vi "FS-EPR(FDMR)-main.vi"() -> ()   [LabVIEW 2022 SP3]
doc: "Demonstrates the fundamentals of the State Machine design pattern in LabVIEW. A state machine, in its simplest form, is a case structure within a while loop, with a state enum wired to a shift register on the loop to define the execution of different cases (or \"states\") of the case structure on different iterations of the loop."
uses:
  Subsystem modules/Messenger service/MessengerLib.lvlib
  Datatypes/TopStates.ctl
  Subsystem modules/Magnet module/ctl/Magnet Orders.ctl
  Subsystem modules/Magnet module/Magnet module.lvlib
  Subsystem modules/Magnet module/ctl/MSG to magnet.ctl
  Subsystem modules/Servo drive module/ctl/Axis names.ctl
  Subsystem modules/Servo drive module/Servo drive module.lvlib
  Subsystem modules/Servo drive module/ctl/Servo MSG.ctl
  Subsystem modules/Servo drive module/ctl/Servo commands.ctl
  Subsystem modules/Magnet module/ctl/SetField data.ctl
  Subsystem modules/Magnet module/ctl/RampingOutput.ctl
  Subsystem modules/Magnet module/ctl/Magnet mode.ctl
  Subsystem modules/Magnet module/ctl/Overall status.ctl
  Subsystem modules/Magnet module/ctl/TM Revision.ctl
  Subsystem modules/Servo drive module/ctl/Servo constants.ctl
  Subsystem modules/Servo drive module/ctl/Servo variables.ctl
  Subsystem modules/Servo drive module/ctl/Servo state.ctl
  Subsystem modules/Servo drive module/ctl/Status variable change.ctl
  Datatypes/Connected modules.ctl
  Subsystem modules/THz module/ctl/THz Message for module.ctl
  Subsystem modules/THz module/THz source modeule.lvlib
  Subsystem modules/Lock-in module/ctl/MFLI_command enum.ctl
  Subsystem modules/Lock-in module/Lock-in module.lvlib
  Subsystem modules/Lock-in module/ctl/MFLI_message for module.ctl
  Subsystem modules/Sample rotator/ctl/Rotator commands.ctl
  Subsystem modules/Sample rotator/SampleRotator.lvlib
  Subsystem modules/Magnet module/ctl/Magnet mode public.ctl
  Subsystem modules/Magnet module/ctl/Actual magnet state.ctl
  Subsystem modules/Sample rotator/ctl/Axis status.ctl
  Subsystem modules/Sample rotator/ctl/Positoin to set.ctl
  Subsystem modules/Sample rotator/ctl/Motion Properties.ctl
  Subsystem modules/Lock-in module/ctl/MFLI parameters.ctl
  <instrlib>/Zurich Instruments LabOne/Public/Data/ziTypeDemodSampleSingle.ctl
  <instrlib>/Zurich Instruments LabOne/Zurich Instruments LabOne.lvlib
  <instrlib>/Zurich Instruments LabOne/Public/ziTypeHandle.ctl
  Subsystem modules/THz module/ctl/THz sweep parameters.ctl
  Subsystem modules/Sample rotator/ctl/MSG to Rotator.ctl
  Subsystem modules/Temperature control module/ctl/TC sensors.ctl
  Subsystem modules/Temperature control module/Temperature controller.lvlib
  Subsystem modules/Temperature control module/ctl/MSG for VTI.ctl
  Subsystem modules/Magnet module/ctl/Cryostat temperature sensors.ctl
  Datatypes/experiment state.ctl
  Subsystem modules/Temperature control module/ctl/TC commands.ctl
  Subsystem modules/Lock-in module/ctl/ACQ info.ctl
  Datatypes/SampleHolders.ctl
  <userlib>/_OpenG.lib/variantconfig/variantconfig.llb/openg_variant_configuration_file.lvlib
  <vilib>/Utility/config.llb/NI_LVConfig.lvlib
  Datatypes/Instr Info.ctl
  Subsystem modules/Lock-in module/ctl/MFLI_parameter and value.ctl
  Datatypes/Single servo status.ctl
  Datatypes/Measurement info.ctl
  Subsystem modules/Temperature control module/ctl/Set point.ctl
  Datatypes/THz parameters.ctl
  Subsystem modules/Lock-in module/ctl/MFLI_node.ctl
  <vilib>/Utility/sysdir.llb/System Directory Type.ctl
  Datatypes/FDMR plus result.ctl
  Subsystem modules/Sample rotator/ctl/Rotator all.ctl
  Datatypes/FDMR+ script line.ctl
  Subsystem modules/Lock-in module/ctl/ADQ data.ctl
  Subsystem modules/THz module/ctl/THz commands enum.ctl
  <vilib>/Analysis/NI_AALPro.lvlib
  <vilib>/Analysis/2dsp.llb/Decimate (single shot, DBL).vi
  Subsystem modules/Lock-in module/ctl/OSC sampling rate.ctl
  Subsystem modules/Source meter/ctls/SMU status.ctl
  Subsystem modules/Source meter/Source meter.lvlib
  Subsystem modules/Source meter/ctls/SMU Commands.ctl
  Subsystem modules/Source meter/ctls/MSG to SMU.ctl
  Subsystem modules/THz module/ctl/THz MW generator constants.ctl
  Datatypes/Magnet controls.ctl
  Datatypes/Servo controls.ctl
  Subsystem modules/Temperature control module/ctl/Set temperature.ctl
  Subsystem modules/Source meter/ctls/SMU settings.ctl
  Datatypes/FDMR script generator options.ctl
  Datatypes/Rotator controls.ctl
  Datatypes/Acquisition controls.ctl
panel:
  out "Instr status":T1 caption="Connected instuments"
  out "Acummulated data":sgl[][](array[numeric])
  out "Lock-in data":T2
  out "FDMR plus results":T3[](array[typedef])
  out "tdms FDMR file ref":refnum<k34>
  out "Controls referencies":T4
  out "Tmp [K]":T5={"1st stage"=34.4, "2nd stage"=3.82, "InMag"=4.12, "OutMag"=4.31, "Plate"=7.68, "Switch"=8.53, "VTI"=55.04, "Sample"=59.48}
  out "Busy":bool
  in  "Stop":bool
  out "Magnetic\nfield state":bool
  out "data time":timestamp
  out "New data":bool
  out "Instr control refs":refnum<vi>[](array[refnum])
  out "Tmp reched time":dbl format="%<%H:%M:%S>T"
  out "VTI tmp reached":bool
  out "Running experiment":bool
  out "Temperature log ref":refnum<file>
  out "1 round\ntime":u32
  out "loggersRef":refnum<file>
  in  "Tab Control":T6(tab)
  out "Drift[K/min]":dbl[](array[numeric])
  in  "Log folder":path=path "C:/HFEPR logs"
  in  "Disconnect":bool
  in  "Select module":T7(ring)
  out "Logger":string[](array[string])
  in  "Re-connect instruments":bool
  in  "System config file path":path=path "M:/Instrument/HFEPR spectrometer/Software developement/Multi-EPR plus ultra/SystemData/config.ini"
  out "Instr info":T8 {"PwrMonitor"."Last update" format="%<%H:%M:%S>T"; "VTI"."Last update" format="%<%H:%M:%S>T"; "PMD"."Last update" format="%<%H:%M:%S>T"; "SMU"."Last update" format="%<%H:%M:%S>T"; "Servo"."Last update" format="%<%H:%M:%S>T"; "Rotator"."Axes"."Actuator" items=["Linear", "Roatator", "Goniometer"]; "Rotator"."Name" items=["ANC350res", "ANC350num", "ANC350fps", "Unknown"]; "Rotator"."Last update" format="%<%H:%M:%S>T"; "THz"."Last update" format="%<%H:%M:%S>T"; "MFLI"."Last update" format="%<%H:%M:%S>T"; "Magnet"."Last update" format="%<%H:%M:%S>T"}
  in  "Use previous settings":bool=TRUE
  out "Temperature monitor":T12(graph)
  in  "Real instruments":bool=TRUE
  in  "Password is admin":string
  in  "VTI control":T13={"VTI space [K]"=1.0, "Sample [K]"=0.0, "Heater3 [K]"=1.8, "Heater4 [K]"=1.8, "Out 1 [%]"=0.0, "Out 2 [%]"=0.0, "Range out 1"=1} {"Range out 1" items=["Off", "Range 1 (On)", "Range 2", "Range 3", "Range 4", "Range 5"]; "Heater4 [K]" min=1.8 max=300.0; "Heater3 [K]" min=1.8 max=300.0}
  in  "Acquisition controls":T14={"ACQ parameters"={"Filter order"=7.0, "Filter tau [ms]"=10.0, "F_Mod [kHz]"=1.0, "Amp_Mod [mV]"=10.0, "Enable output"=0, "Phase [°]"=0.0}, "ACQ shot btn"=FALSE, "Modulation [A]"=0.0, "In50"=FALSE, "Out50"=FALSE, "DemEn"=FALSE, "Actual [G]"=0.0, "Sample holder"=enum."Simple", "Desired [G]"=0.0, "Adj mod"=FALSE, "Auto-modulation"=TRUE, "Autorange"=FALSE, "AuxIn0 [V]"=0.0, "AuxIn1 [V]"=0.0} {"AuxIn1 [V]" format="%#_3g"; "AuxIn0 [V]" format="%#_3g"; "Desired [G]" format="%.1g"; "ACQ parameters"."Enable output" items=["Disable", "Enable"]; "ACQ parameters"."Amp_Mod [mV]" min=0.0 max=10000.0; "ACQ parameters"."F_Mod [kHz]" min=0.1 max=500.0; "ACQ parameters"."Filter order" min=1.0 max=9.0 step=1.0; "ACQ parameters"."Filter tau [ms]" min=0.0 max=1000.0}
  in  "VID control":T17={"AMC"=9, "Multip"=1, "Base frequency [GHz]"=0.0, "End frequency [GHz]"=0.0, "Im frequency [MHz]"=1500.0, "Sweep up [ms]"=0.0, "Reset trigger?"=FALSE} {"Multip" items=["1"=1, "2"=2, "3"=3, "4"=4, "6"=6, "8"=8, "9"=9]; "AMC" items=["9"=9, "12"=12]; "End frequency [GHz]" min=0.00018 max=20000.0; "Base frequency [GHz]" min=162.0 max=252.0}
  in  "Servo controls":T18={"Y left"=FALSE, "Y right"=FALSE, "X backward"=FALSE, "X forward"=FALSE, "Zdown"=FALSE, "Zup"=FALSE, "Step\n[mm]"=5.0, "QO table"={"ZLdown"=FALSE, "ZLup"=FALSE, "ZRup"=FALSE, "ZRdown"=FALSE, "ZMdown"=FALSE, "ZMup"=FALSE}, "X"=0.0, "Y"=0.0, "ZL"=0.0, "ZR"=0.0, "ZM"=0.0, "Measure Position btn"=FALSE, "Eject position btn"=FALSE, "Stop servo btn"=FALSE, "Save position btn"=FALSE} {"Step\n[mm]" min=0.0 max=600.0 step=5.0}
  in  "Magnet controls":T19 {"Output\n[T]" scale=0.0..16.0; "Field\n[T]" scale=0.0..16.0; "Desired ramp\nrate [mT/s]" max=7.544966; "Set Field [T]" max=16.0}
  out "lookup":cluster{"X (Vrms)":dbl, "Y (Vrms)":dbl}(graph) caption="Waveform Chart - Dark"
  in  "SMU controls":T21={"Apply"=FALSE, "Measurement settings"={"Source Mode "=1, "Source Level"=0.1, "Source Limit"=0.3, "Measure Function"=0, "Remote sense"=TRUE, "Clear buffer?"=FALSE, "Beep"=TRUE, "High Capacity"=TRUE, "Terminals"=0, "PLCs"=1.0, "Fast measurement"=FALSE}, "Value"=0.1006, "Stop"=FALSE, "Record"=FALSE, "B[T]"=0.0, "Refresh"=FALSE} {"Value" format="%#_3e"; "Measurement settings"."Measure Function" items=["Volts", "Current", "Auto Resistance", "Manual Resistance", "Digitize Voltage", "Digitize Current"]; "Measurement settings"."Source Level" max=0.3; "Measurement settings"."Source Mode" items=["Voltage", "Current"]; "Measurement settings"."Terminals" items=["Front", "Rear"]}
  in  "Rotator controls":T22={"Motion properties"={"Frequency [Hz]"=1000.0, "MaxErr [µm|m°]"=100.0, "DC voltage [V]"=0.0, "Amplitude [V]"=25.0, "Position [mm|°]"=0.0, "EoF"=FALSE, "EoB"=FALSE, "Error"=FALSE, "Target [mm|°]"=0.0}, "Set position"={"Relative?"=FALSE, "Position [°]"=0.0, "Safe to move?"=FALSE}, "Actual \nangle[°]"=0.0, "Rot set properties btn"=FALSE, "Rot set position btn"=FALSE, "Stop btn"=FALSE, "EoF"=FALSE, "EoB"=FALSE, "Error"=FALSE} {"Motion properties"."Amplitude [V]" min=0.0 max=60.0 step=1.0; "Motion properties"."DC voltage [V]" min=0.0 max=60.0 step=1.0; "Motion properties"."MaxErr [µm|m°]" min=1.0 max=1000.0 step=1.0; "Motion properties"."Frequency [Hz]" min=0.1 max=5000.0 step=10.0}
  in  "Save data option":bool
  in  "Load from editor btn":bool
  out "Line":i32
  in  "Script array":T25[](array[typedef])=[{"F_start [GHz]"=180.0, "F_end [GHz]"=196.0, "Field [T]"=6.8, "Points [-]"=8000, "Sampling Rate"=13, "ModA [G]"=4.0, "ModF [kHz]"=40.1, "Time const [ms]"=0.5, "Angle [°]"=-1.0, "Tmp [K]"=55.0, "Wait [min]"=5.0, "Repeat [-]"=127, "Comment"="example comment", "Execute"=TRUE, "Auto-mod"=FALSE}] {"Sampling Rate" items=["117 ks/S"=9, "58.6 kS/s"=10, "29.3 kS/s"=11, "14.6 kS/s"=12, "7.32 kS/s"=13, "3.66 kS/s"=14, "1.83 kS/s"=15]; "Angle [°]" min=-1.0 max=330.0; "ModA [G]" min=0.0 max=50.0; "Repeat [-]" min=0 max=1048576; "Points [-]" min=4096 max=5000000 step=1; "Field [T]" min=-16.0 max=16.0}
  out "Live spectrum":dbl[][](graph) caption="Live Spectrum"
  in  "Folder path":path
  in  "Sample name":string="Unknown"
  in  "Run FDMR+ btn":bool
  in  "Direct stop meas. btn":bool
  out "Infobar":T27={"Remains"=0.0, "T_sample [K]"=59.48, "Last log"="Measurement has finished at 11:20:43", "Experiment state"=enum."Setup", "Field [T]"=6.8, "Sample holder"=enum."Simple", "Started"=timestamp(38104 s since 1904-01-01)} {"Started" format="%<%H:%M:%S>T"; "Remains" format="%<%H:%M:%S>t"}
  out "Accumulated Spectrum":dbl[][](graph)
  out "Round":i32
  in  "Load from measurement btn":bool
  in  "Save script btn":bool
  in  "Clear script btn":bool
  in  "Generate script btn":bool
  in  "Generator options":T29
  in  "Editor script":T25[](array[typedef]) {"Sampling Rate" items=["117 ks/S"=9, "58.6 kS/s"=10, "29.3 kS/s"=11, "14.6 kS/s"=12, "7.32 kS/s"=13, "3.66 kS/s"=14, "1.83 kS/s"=15]; "Angle [°]" min=-1.0 max=330.0; "ModA [G]" min=0.0 max=50.0; "Repeat [-]" max=1048576; "Points [-]" min=4096 max=5000000 step=1; "Field [T]" min=-16.0 max=16.0}
  in  "Prototype line":T25={"F_start [GHz]"=380.0, "F_end [GHz]"=400.0, "Field [T]"=0.0, "Points [-]"=1, "Sampling Rate"=15, "ModA [G]"=100.0, "ModF [kHz]"=10.0, "Time const [ms]"=1.0, "Angle [°]"=-1.0, "Tmp [K]"=295.0, "Wait [min]"=0.0, "Repeat [-]"=1, "Comment"="", "Execute"=FALSE, "Auto-mod"=FALSE} {"Sampling Rate" items=["117 ks/S"=9, "58.6 kS/s"=10, "29.3 kS/s"=11, "14.6 kS/s"=12, "7.32 kS/s"=13, "3.66 kS/s"=14, "1.83 kS/s"=15]; "Angle [°]" min=-1.0 max=330.0; "ModA [G]" min=0.0 max=50.0; "Repeat [-]" max=1048576; "Points [-]" min=4096 max=5000000 step=1; "Field [T]" min=-16.0 max=16.0}
  out "Opend review file path":path
  out "Current review graph parameters":T25={"F_start [GHz]"=380.0, "F_end [GHz]"=400.0, "Field [T]"=0.0, "Points [-]"=1, "Sampling Rate"=15, "ModA [G]"=1.0, "ModF [kHz]"=10.0, "Time const [ms]"=1.0, "Angle [°]"=-1.0, "Tmp [K]"=295.0, "Wait [min]"=0.0, "Repeat [-]"=0, "Comment"="", "Execute"=FALSE, "Auto-mod"=FALSE} {"Sampling Rate" items=["117 ks/S"=9, "58.6 kS/s"=10, "29.3 kS/s"=11, "14.6 kS/s"=12, "7.32 kS/s"=13, "3.66 kS/s"=14, "1.83 kS/s"=15]; "Time const [ms]" min=-1.0 max=330.0; "ModF [kHz]" min=0.2 max=120.0; "Repeat [-]" max=1048576; "Points [-]" max=50; "Wait [min]" max=1048576.0; "Field [T]" min=-16.0 max=16.0}
  out "Previous graph":sgl[][](graph)
  out "Current graph":sgl[][](graph)
  in  "Open measurement":bool
  in  "Data to show":u16(ring) items=["Empty", "Empty", "Empty", "Empty", "Empty", "Empty", "Empty", "Empty", "Empty", "Empty"]
  # "Action part"
  # "Status part"
  # "Option 1:\nchoice primary and secondary sweep\n\nOption 2:\nChoice measurement mode, and appropriate cluster will apear. Other clusters wil be hidden.\n\n\nOption 3:\nChoice measurement mode.\nInternal parts of single cluster will (dis)apear if needed.\n\nNote:\nPosibility to do an orientation/temperature deppendency."
  # "Tmp [K]"
  # "Position [mm]"
  # "Z"
  # "X/Y"
  # "This software was developed for HFEPR spectrometer in 2019 (2020) at CEITEC BUT by members of MOTES research group.\n\nQuick guide:\n1) Re-connect to all instruments.\n2) Check if necessary instruments are ready. (At least VTI, VDI, Lock-In, and Magnet has to work)\n3) Go to Adjustment tab and set up Lock-in parameters as well as VDI multipiers.\n4) Go to EPR measurement tab, select folder path, fill the sample description.\n5) Fill at least 1 line of the script and press Run script button.\n\n6) In case of a bug please report this to software developer or make a note into developement diary loaceted at:\n    RG-1-12/Instriments/HFEPR spectrometer/Software developement.\n\nLast update: 07.02. 2020 - Script editor is working, measurement review not yet.\n\nSpecial thanks to: Luke Skywalker, my mom, Tonda's mom, Pilsner, God, Oleksi, Vinicius, Petr from parallel universe.\n\n \nTODO: Invisible controls: referencies for: adjustment controls, meas results, loggerRef,"
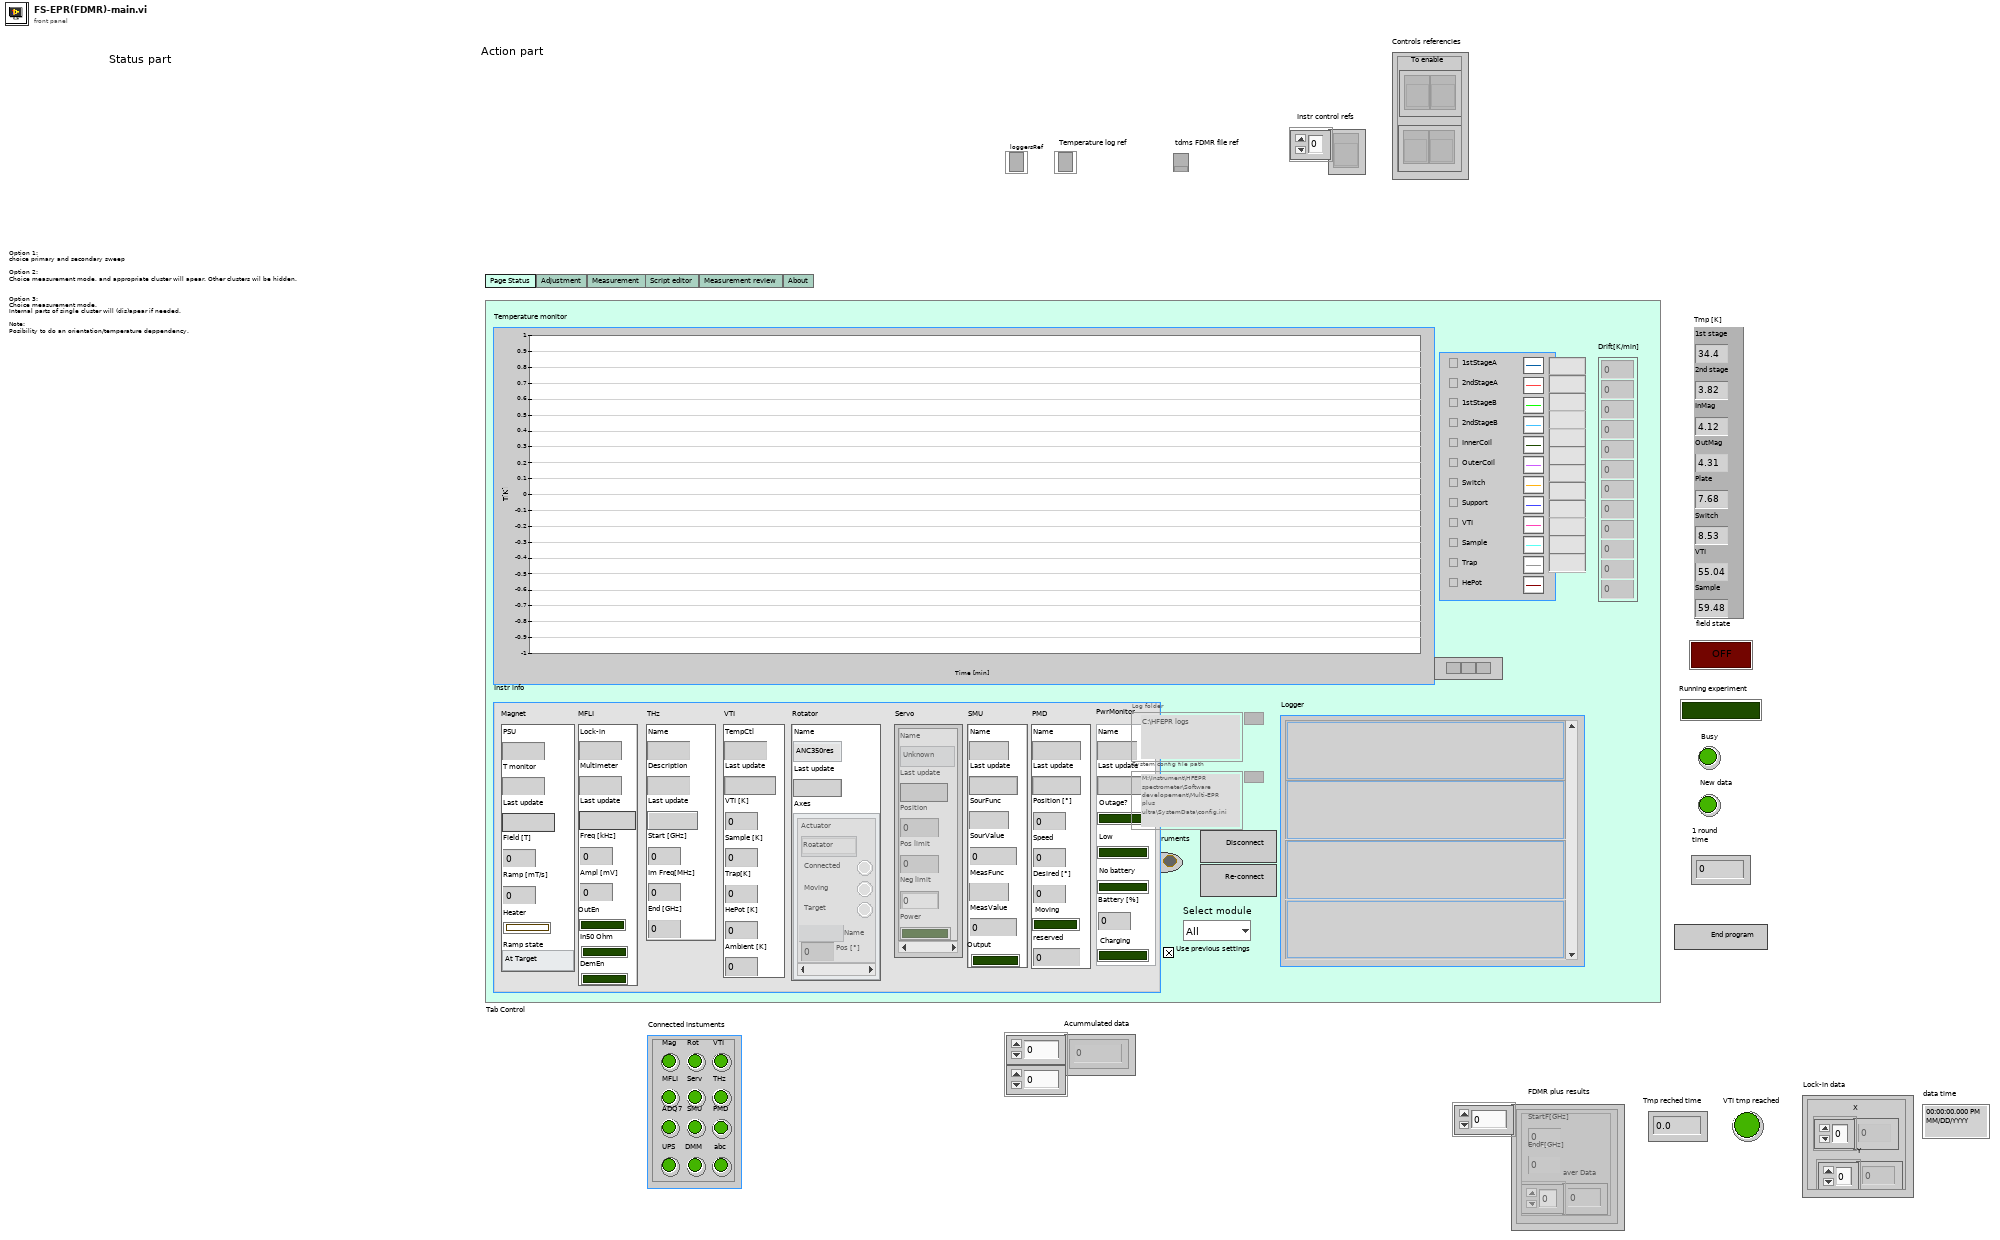
[diagram p1: front panel]
types:
  T1 = typedef "Connected modules.ctl" = cluster{"Mag":bool, "Rot":bool, "VTI":bool, "MFLI":bool, "Serv":bool, "THz":bool, "ADQ7":bool, "SMU":bool, "PMD":bool, "UPS":bool, "DMM":bool, "abc":bool}
  T2 = typedef "Lock-in module.lvlib/ADQ data.ctl" = cluster{"X":sgl[], "Y":sgl[]}
  T3 = typedef "FDMR plus result.ctl" = cluster{"StartF[GHz]":dbl, "EndF[GHz]":dbl, "aver Data":dbl[]}
  T4 = cluster{"To disable":refnum<vi>[], "To enable":refnum<vi>[]}
  T5 = cluster{"1st stage":dbl, "2nd stage":dbl, "InMag":dbl, "OutMag":dbl, "Plate":dbl, "Switch":dbl, "VTI":dbl, "Sample":dbl}
  T6 = enum32{"Page Status", "Adjustment", "Measurement", "Script editor", "Measurement review", "About"}
  T7 = enum16{"All", "None", "ACQ", "THz", "MAG", "SERV", "ROT", "VTI", "SMU"}
  T8 = typedef "Instr Info.ctl" = cluster{"Magnet":cluster{"PSU":string, "T monitor":string, "Last update":timestamp, "Field [T]":dbl, "Ramp [mT/s]":dbl, "Heater":bool, "Ramp state":T9}, "MFLI":cluster{"Lock-in":string, "Multimeter":string, "Last update":timestamp, "Freq [kHz]":dbl, "Ampl [mV]":dbl, "OutEn":bool, "In50 Ohm":bool, "DemEn":bool}, "THz":cluster{"Name":string, "Description":string, "Last update":timestamp, "Start [GHz]":dbl, "Im Freq[MHz]":dbl, "End [GHz]":dbl}, "VTI":cluster{"TempCtl":string, "Last update":timestamp, "VTI [K]":dbl, "Sample [K]":dbl, "Trap[K]":dbl, "HePot [K]":dbl, "Ambient [K]":dbl}, "Rotator":cluster{"Name":i32, "Last update":timestamp, "Axes":cluster{"Pos [°]":dbl, "Moving":bool, "Name":string, "Actuator":u16, "Target":bool, "Connected":bool}[]}, "Servo":T10[], "SMU":cluster{"Name":string, "Last update":timestamp, "SourFunc":string, "SourValue":dbl, "MeasFunc":string, "MeasValue":dbl, "Output":bool}, "PMD":cluster{"Name":string, "Last update":timestamp, "Position [°]":dbl, "Speed":dbl, "Desired [°]":dbl, "Moving":bool, "reserved":dbl}, "PwrMonitor":cluster{"Name":string, "Last update":timestamp, "Outage?":bool, "Low":bool, "No battery":bool, "Battery [%]":u8, "Charging":bool}}
  T9 = typedef "Magnet module.lvlib/RampingOutput.ctl" = enum16{"At Target", "Go up", "Go down"}
  T10 = typedef "Single servo status.ctl" = cluster{"Name":T11, "Last update":timestamp, "Position":dbl, "Pos limit":dbl, "Neg limit":dbl, "Power":bool}
  T11 = typedef "Servo drive module.lvlib/Axis names.ctl" = enum16{"Unknown", "AxisX", "AxisY", "AxisZ_left", "AxisZ_middle", "AxisZ_right"}
  T12 = cluster{"[0]":dbl, "[1]":dbl, "[2]":dbl, "[3]":dbl, "[4]":dbl, "[5]":dbl, "[6]":dbl, "[7]":dbl, "[8]":dbl, "[9]":dbl, "[10]":dbl, "[11]":dbl}
  T13 = typedef "Temperature controller.lvlib/Set temperature.ctl" = cluster{"VTI space [K]":dbl, "Sample [K]":dbl, "Heater3 [K]":dbl, "Heater4 [K]":dbl, "Out 1 [%]":dbl, "Out 2 [%]":dbl, "Range out 1":u16}
  T14 = typedef "Acquisition controls.ctl" = cluster{"ACQ parameters":T15, "ACQ shot btn":bool, "Modulation [A]":dbl, "In50":bool, "Out50":bool, "DemEn":bool, "Actual [G]":dbl, "Sample holder":T16, "Desired [G]":dbl, "Adj mod":bool, "Auto-modulation":bool, "Autorange":bool, "AuxIn0 [V]":dbl, "AuxIn1 [V]":dbl}
  T15 = typedef "Lock-in module.lvlib/MFLI parameters.ctl" = cluster{"Filter order":dbl, "Filter tau [ms]":dbl, "F_Mod [kHz]":dbl, "Amp_Mod [mV]":dbl, "Enable output":u16, "Phase [°]":dbl}
  T16 = typedef "SampleHolders.ctl" = enum16{"Simple", "Carousel", "Chip", "Rotator", "Liquid"}
  T17 = typedef "THz parameters.ctl" = cluster{"AMC":u16, "Multip":u16, "Base frequency [GHz]":dbl, "End frequency [GHz]":dbl, "Im frequency [MHz]":dbl, "Sweep up [ms]":dbl, "Reset trigger?":bool}
  T18 = typedef "Servo controls.ctl" = cluster{"Y left":bool, "Y right":bool, "X backward":bool, "X forward":bool, "Zdown":bool, "Zup":bool, "Step\n[mm]":dbl, "QO table":cluster{"ZLdown":bool, "ZLup":bool, "ZRup":bool, "ZRdown":bool, "ZMdown":bool, "ZMup":bool}, "X":dbl, "Y":dbl, "ZL":dbl, "ZR":dbl, "ZM":dbl, "Measure Position btn":bool, "Eject position btn":bool, "Stop servo btn":bool, "Save position btn":bool}
  T19 = typedef "Magnet controls.ctl" = cluster{"Set Field [T]":dbl, "Desired ramp\nrate [mT/s]":dbl, "Custom\nramp":bool, "Mode switch":bool, "Pause ramp":bool, "Field\n[T]":dbl, "Output\n[T]":dbl, "Equalize":bool, "Discharge":bool, "Switch \ntmp [K]":dbl, "Direction":bool}
  T20 = typedef "SMU settings.ctl" = cluster{"Source Mode ":u16, "Source Level":dbl, "Source Limit":dbl, "Measure Function":u16, "Remote sense":bool, "Clear buffer?":bool, "Beep":bool, "High Capacity":bool, "Terminals":u16, "PLCs":dbl, "Fast measurement":bool}
  T21 = cluster{"Apply":bool, "Measurement settings":T20, "Value":dbl, "Stop":bool, "Record":bool, "B[T]":dbl, "Refresh":bool}
  T22 = typedef "Rotator controls.ctl" = cluster{"Motion properties":T23, "Set position":T24, "Actual \nangle[°]":dbl, "Rot set properties btn":bool, "Rot set position btn":bool, "Stop btn":bool, "EoF":bool, "EoB":bool, "Error":bool}
  T23 = typedef "Motion Properties.ctl" = cluster{"Frequency [Hz]":dbl, "MaxErr [µm|m°]":dbl, "DC voltage [V]":dbl, "Amplitude [V]":dbl, "Position [mm|°]":dbl, "EoF":bool, "EoB":bool, "Error":bool, "Target [mm|°]":dbl}
  T24 = typedef "Positoin to set.ctl" = cluster{"Relative?":bool, "Position [°]":dbl, "Safe to move?":bool}
  T25 = typedef "FDMR+ script line.ctl" = cluster{"F_start [GHz]":dbl, "F_end [GHz]":dbl, "Field [T]":dbl, "Points [-]":u32, "Sampling Rate":T26, "ModA [G]":dbl, "ModF [kHz]":dbl, "Time const [ms]":dbl, "Angle [°]":dbl, "Tmp [K]":dbl, "Wait [min]":dbl, "Repeat [-]":i32, "Comment":string, "Execute":bool, "Auto-mod":bool}
  T26 = typedef "OSC sampling rate.ctl" = u16
  T27 = typedef "Measurement info.ctl" = cluster{"Remains":dbl, "T_sample [K]":dbl, "Last log":string, "Experiment state":T28, "Field [T]":dbl, "Sample holder":T16, "Started":timestamp}
  T28 = typedef "experiment state.ctl" = enum16{"Setup", "Preparation", "Stabilization", "Begin", "Acquisition", "Save"}
  T29 = typedef "FDMR script generator options.ctl" = cluster{"Field step [T]":dbl, "Angle step[°]":dbl, "Tmp step [K]":dbl, "Iterations[-]":u16, "Script generator option":bool}
  T30 = typedef "TopStates.ctl" = enum16{"Initialize GUI", "Wait for Event", "Check message", "Check measurement", "Stop", "Restart"}
  T31 = typedef "MessengerLib.lvlib/Messenger referencies.ctl" = cluster{"TOP":refnum<queue>, "Instr_M":refnum<queue>, "Field_C":refnum<queue>, "Tmp_M":refnum<queue>, "Tmp_C":refnum<queue>, "Table_C":refnum<queue>, "MW_C":refnum<queue>, "Data_Aq":refnum<queue>, "Mod_M":refnum<queue>, "Field_M":refnum<queue>, "Pwr_M":refnum<queue>, "Angle_C":refnum<queue>, "Sample_C":refnum<queue>, "Reserved":refnum<queue>}
  T32 = enum16{"All", "None", "ACQ", "THz", "MAG", "SERV", "ROT", "VTI"}
  T33 = enum8{"Enabled", "Disabled", "Disabled and Grayed Out"}
  T34 = typedef "Magnet module.lvlib/Magnet mode public.ctl" = enum16{"Persistant", "Ramping"}
  T35 = typedef "Magnet module.lvlib/SetField data.ctl" = cluster{"Field [T]":dbl, "Ramp [T/s]":dbl, "Custom Ramp?":bool, "Mode":T34}
  T36 = typedef "Magnet module.lvlib/Magnet Orders.ctl" = enum16{"Ignore", "Connect", "Update", "Switch mode", "Set field", "Stop ramping", "Equalize output", "Zero output", "Flip polarity", "Blackout", "Set timer", "Eval temperatures", "Disconnect"}
  T37 = typedef "Magnet module.lvlib/MSG to magnet.ctl" = cluster{"Command":T36, "Data":variant}
  T38 = typedef "Servo drive module.lvlib/Servo commands.ctl" = enum16{"Initialize", "Update", "Move by", "Move to", "Stop", "Ignore", "Disconnect", "End"}
  T39 = typedef "Servo drive module.lvlib/Servo MSG.ctl" = cluster{"Command":T38, "Data":variant}
  T40 = typedef "Source meter.lvlib/MSG to SMU.ctl" = cluster{"Command":T41, "Data":variant}
  T41 = typedef "Source meter.lvlib/SMU Commands.ctl" = enum16{"Ignore", "Connect", "Update", "Set measurement", "Start measurement", "Get actual results", "Stop measurement", "Disconnect", "End"}
  T42 = typedef "SampleRotator.lvlib/MSG to Rotator.ctl" = cluster{"Command":T43, "Data":variant}
  T43 = typedef "SampleRotator.lvlib/Rotator commands.ctl" = enum16{"Ignore", "Initialize", "Initialize axes", "Update", "Set parameters", "Stop movement", "Set position", "Disconnect", "End"}
  T44 = typedef "THz source modeule.lvlib/THz commands enum.ctl" = enum16{"Ignore", "Connect", "Update", "Set parameters", "Disconnect", "End"}
  T45 = typedef "THz source modeule.lvlib/THz sweep parameters.ctl" = cluster{"Start [GHz]":dbl, "End [GHz] ":dbl, "Sweep up\ntime [ms]":dbl, "Sweep down\ntime [ms]":dbl, "Intermidiate [MHz]":dbl, "Reset trigger":bool}
  T46 = typedef "THz source modeule.lvlib/THz Message for module.ctl" = cluster{"Command":T44, "Data":variant}
  T47 = typedef "Lock-in module.lvlib/MFLI_parameter and value.ctl" = cluster{"parameter":T48, "value":dbl}
  T48 = typedef "Lock-in module.lvlib/MFLI_node.ctl" = enum16{"None", "filter_order [-]", "filter_constant [ms]", "in_diff", "in_autorange", "in_imp50", "in_AC", "osc_freq [kHz]", "out_ampl [V]", "out_autorange", "out_imp50", "enable output", "enamble ampl", "scope_enable", "scope_rate", "scope_len", "scope_trigEn", "AuxOut_amplify", "Phase_deg", "AuxOut_select"}
  T49 = typedef "Lock-in module.lvlib/MFLI_command enum.ctl" = enum16{"Initialize", "Update", "Set parameters", "Set module", "Set individual parameters", "Get point", "Get array", "Disconnect", "End", "Ignore"}
  T50 = typedef "Lock-in module.lvlib/MFLI_message for module.ctl" = cluster{"Command":T49, "Data":variant}
  T51 = typedef "Temperature controller.lvlib/Set point.ctl" = cluster{"Heater":string, "Tmp [K]":dbl}
  T52 = typedef "Temperature controller.lvlib/TC commands.ctl" = enum16{"Initialize", "Update", "Stop tmp change", "Set temperature", "Set point", "Disconnect", "End", "Ignore"}
  T53 = typedef "Temperature controller.lvlib/MSG for VTI.ctl" = cluster{"Command":T52, "Data":variant}
  T54 = typedef "THz source modeule.lvlib/THz MW generator constants.ctl" = cluster{"Lower limit [GHz]":dbl, "Upper limit [GHz]":dbl, "Device name":string, "Connection":string, "Description":string, "Connected":bool, "Last settings":string, "Operation mode":enum16{"Disabled", "CW", "Arbitrary", "Sweep"}, "Enable ch 1":bool, "Enable ch 2":bool}
  T55 = typedef "Magnet module.lvlib/TM Revision.ctl" = cluster{"Instr Serial Number":string, "Instr Driver Revision":string, "Instr Firmware Revision":string, "Instr Model Number":string}
  T56 = typedef "Magnet module.lvlib/Overall status.ctl" = cluster{"Desired":T35, "Actual":T57}
  T57 = typedef "Magnet module.lvlib/Actual magnet state.ctl" = cluster{"Mode":T58, "Ramping output":T9, "Ready for change":bool, "Switch heater":bool, "Cooler Overheat":bool, "Coil overheat":bool, "Energized":bool, "Output [T]":dbl, "Field [T]":dbl, "Ramp[T/s]":dbl, "Switch\ntemperature [K]":dbl, "Voltage [V]":dbl, "Current direction":bool}
  T58 = typedef "Magnet module.lvlib/Magnet mode.ctl" = enum16{"Persistant", "Switching", "Ramping", "Quenched"}
  T59 = typedef "Magnet module.lvlib/Cryostat temperature sensors.ctl" = cluster{"First stage A [K]":dbl, "Second stage A [K]":dbl, "Firs stage B [K]":dbl, "Second stage B [K]":dbl, "Inner magnet [K]":dbl, "Outer Magnet [K]":dbl, "Switch [K]":dbl, "Support plate [K]":dbl, "Time stamp":dbl}
  T60 = typedef "Lock-in module.lvlib/ACQ info.ctl" = cluster{"In50":bool, "InAC":bool, "InDiff":bool, "Out50":bool, "OutEN":bool, "OutF[Hz]":dbl, "OutA[V]":dbl, "DemEN":bool, "Const[ms]":dbl, "Order[-]":i32, "Phase [°]":dbl}
  T61 = enum32{"Page Status", "Adjustment", "EPR measurement", "About"}
  T62 = typedef "Zurich Instruments LabOne.lvlib/ziTypeDemodSampleSingle.ctl" = cluster{"Timestamps (ticks)":u64, "X (Vrms)":dbl, "Y (Vrms)":dbl, "Osc Phase (deg)":dbl, "Freq (Hz)":dbl, "DIO":u32, "AuxIn0 (V)":dbl, "AuxIn1 (V)":dbl, "Trigger":u32}
  T63 = typedef "Zurich Instruments LabOne.lvlib/ziTypeHandle.ctl" = cluster{"handleValid":bool, "Conn":u64, "Path Prefix":string, "Handle":u64, "Connected":bool, "Clockbase(s)":dbl}
  T64 = typedef "Source meter.lvlib/SMU status.ctl" = cluster{"VISA name":refnum<visa-resource-name>, "Connected":bool, "Name":string, "Message":string, "Error message":string, "Min voltage":dbl, "Max voltage":dbl, "Min Current":dbl, "Max Current":dbl, "Measurement value":dbl, "Source Voltage":dbl, "Measurement":bool, "Source Current":dbl, "Source Mode":u16, "Measure Function":u16}
  T65 = typedef "Temperature controller.lvlib/TC sensors.ctl" = cluster{"VTI space":dbl, "Sample":dbl, "He pot":dbl, "Trap":dbl, "Ambient":dbl, "SetP_VTI":dbl, "SetP_Smp":dbl, "SetP_Pot":dbl, "SetP_Trap":dbl, "Range out 1":u16, "Out 1 [%]":dbl, "Out 2 [%]":dbl}
  T66 = typedef "Servo drive module.lvlib/Servo state.ctl" = cluster{"Servo variables":T67, "Servo constants":T68, "Connection":variant}
  T67 = typedef "Servo drive module.lvlib/Servo variables.ctl" = cluster{"Terget reached":bool, "Connected":bool, "Power ON":bool, "Operation mode":bool, "Actual position":dbl, "Target position":dbl}
  T68 = typedef "Servo drive module.lvlib/Servo constants.ctl" = cluster{"Name":T11, "Pos position limit [mm]":dbl, "Neg position limit [mm]":dbl, "Pos velocity limit":dbl, "Neg velocity limit":dbl, "Acceleration limit":dbl}
  T69 = typedef "Servo drive module.lvlib/Status variable change.ctl" = cluster{"Property":string, "Value":variant, "Name":T11}
  T70 = typedef "SampleRotator.lvlib/Rotator all.ctl" = cluster{"Controller info":cluster{"deviceNumber":i32, "DeviceType":i32, "ID":u32, "Serial":string, "Address":string, "connected":bool}, "Handle":u64, "FW-Version":i32, "Features":u32, "Axes":T71[], "Path to DLL":path}
  T71 = typedef "SampleRotator.lvlib/Axis status.ctl" = cluster{"Axis status":cluster{"Connected":bool, "Enabled":bool, "Moving":bool, "Target":bool, "EndForward":bool, "EndBackarwd":bool, "Error":bool}, "Position [°]":dbl, "Frequency [Hz]":dbl, "Voltage [V]":dbl, "Capacitance[uF]":dbl, "Name":string, "ActuatorType":u16, "DC offset [V]":dbl, "Tolerance [m°]":dbl, "Index":u8}
  T72 = enum16{"None", "Unity norm", "Mean norm", "Standardization"}
  T73 = enum16{"open", "open or create", "create or replace", "create", "open (read-only)"}
  T74 = typedef "NI_LVConfig.lvlib/Config Data RefNum.ctl" = refnum<k1>
  T75 = typedef "System Directory Type.ctl" = i32
  T76 = typedef "Mudules status.ctl" = cluster{"Mag":bool, "Rot":bool, "VTI":bool, "MFLI":bool, "Serv":bool, "THz":bool, "ADQ7":bool, "SMU":bool, "PMD":bool, "UPS":bool, "DMM":bool, "abc":bool}
  T77 = typedef "Magnet module.lvlib/Magnet config constants.ctl" = cluster{"Switch resistant [K]":dbl, "Switch superconducting [K]":dbl, "First stage critical temperature [K]":dbl, "Second stage critical temperature [K]":dbl, "Inner magnet critical temperature [K]":dbl, "Outer magnet critical temperature [K]":dbl, "Field Constant [T/A]":dbl, "Maximum Current [A]":dbl, "Maximum field [T]":dbl, "Maximum source ramp [A/s]":dbl, "Source precision [T]":dbl, "Ramp limits [A/s]":dbl[], "Field limits [T]":dbl[], "SMS":refnum<visa-resource-name>, "LSC218":refnum<visa-resource-name>}
  T78 = typedef "MessengerLib.lvlib/MSG to TOP.ctl" = cluster{"Module":T79, "Response":string, "Data":variant, "Time":timestamp}
  T79 = typedef "Module name.ctl" = enum16{"Emty", "Magnet", "VTI", "Excitation", "Servo", "Acquisition", "Rotator", "Digitizer", "SMU2450", "Carousel", "Multimeter", "Tmp monitor", "Power monitor"}
  T80 = cluster{"PSU":string, "T monitor":string, "Last update":timestamp, "Field [T]":dbl, "Ramp [mT/s]":dbl, "Heater":bool, "Ramp state":T9}
  T81 = cluster{"TC":string, "Last update":timestamp, "VTI [K]":dbl, "Sample [K]":dbl, "Trap[K]":dbl, "HePot [K]":dbl, "Ambient [K]":dbl}
  T82 = cluster{"Name":string, "Description":string, "Last update":timestamp, "Start [GHz]":dbl, "Im Freq[MHz]":dbl, "End [GHz]":dbl}
  T83 = cluster{"Lock-in":string, "Multimeter":string, "Last update":timestamp, "Freq [kHz]":dbl, "Ampl [mV]":dbl, "OutEn":bool, "In50 Ohm":bool, "DemEn":bool}
  T84 = cluster{"Name":string, "Last update":timestamp, "SourFunc":string, "SourValue":dbl, "MeasFunc":string, "MeasValue":dbl, "Output":bool}
  T85 = cluster{"TempCtl":string, "Last update":timestamp, "VTI [K]":dbl, "Sample [K]":dbl, "Trap[K]":dbl, "HePot [K]":dbl, "Ambient [K]":dbl}
  T86 = cluster{"Name":i32, "Last update":timestamp, "Axes":cluster{"Pos [°]":dbl, "Moving":bool, "Name":string, "Actuator":u16, "Target":bool, "Connected":bool}[]}
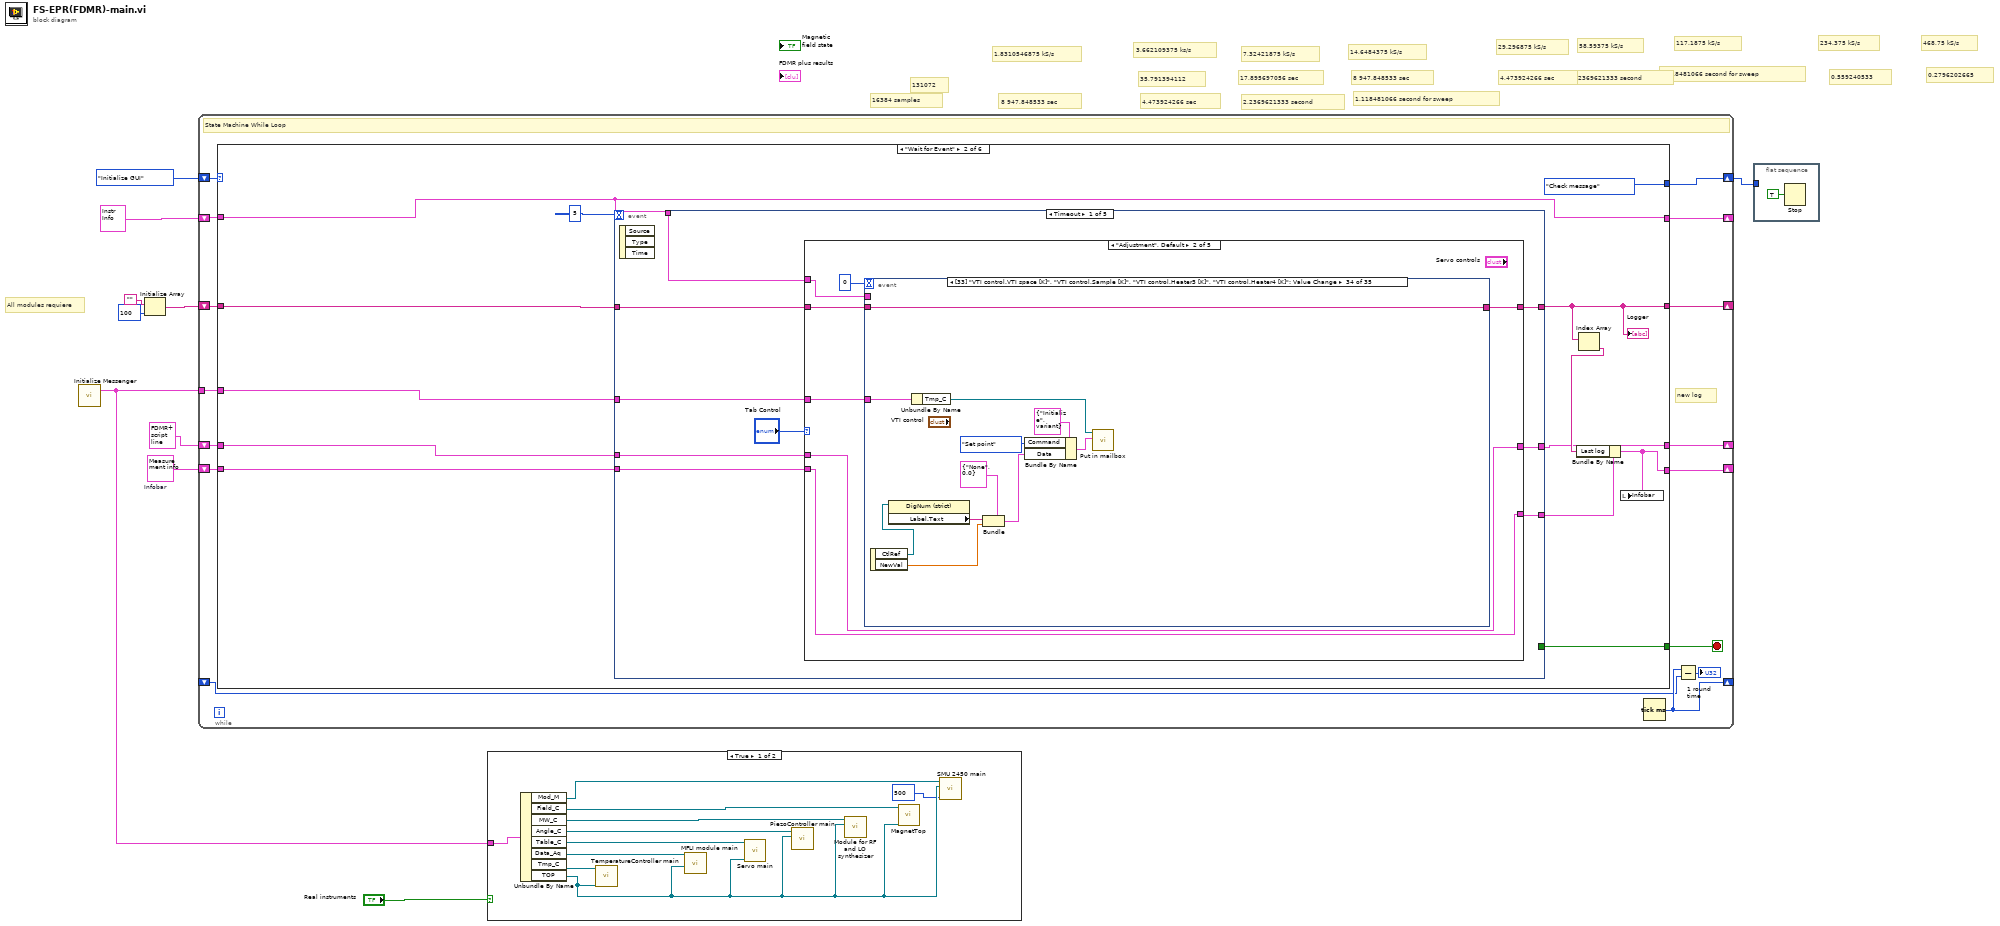
[diagram p0: block diagram]
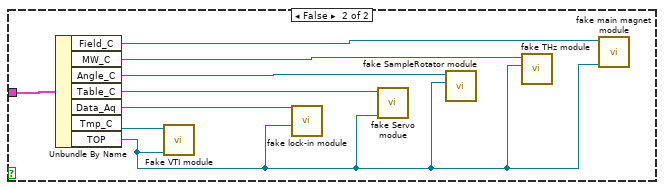
[diagram p2: hidden frame]
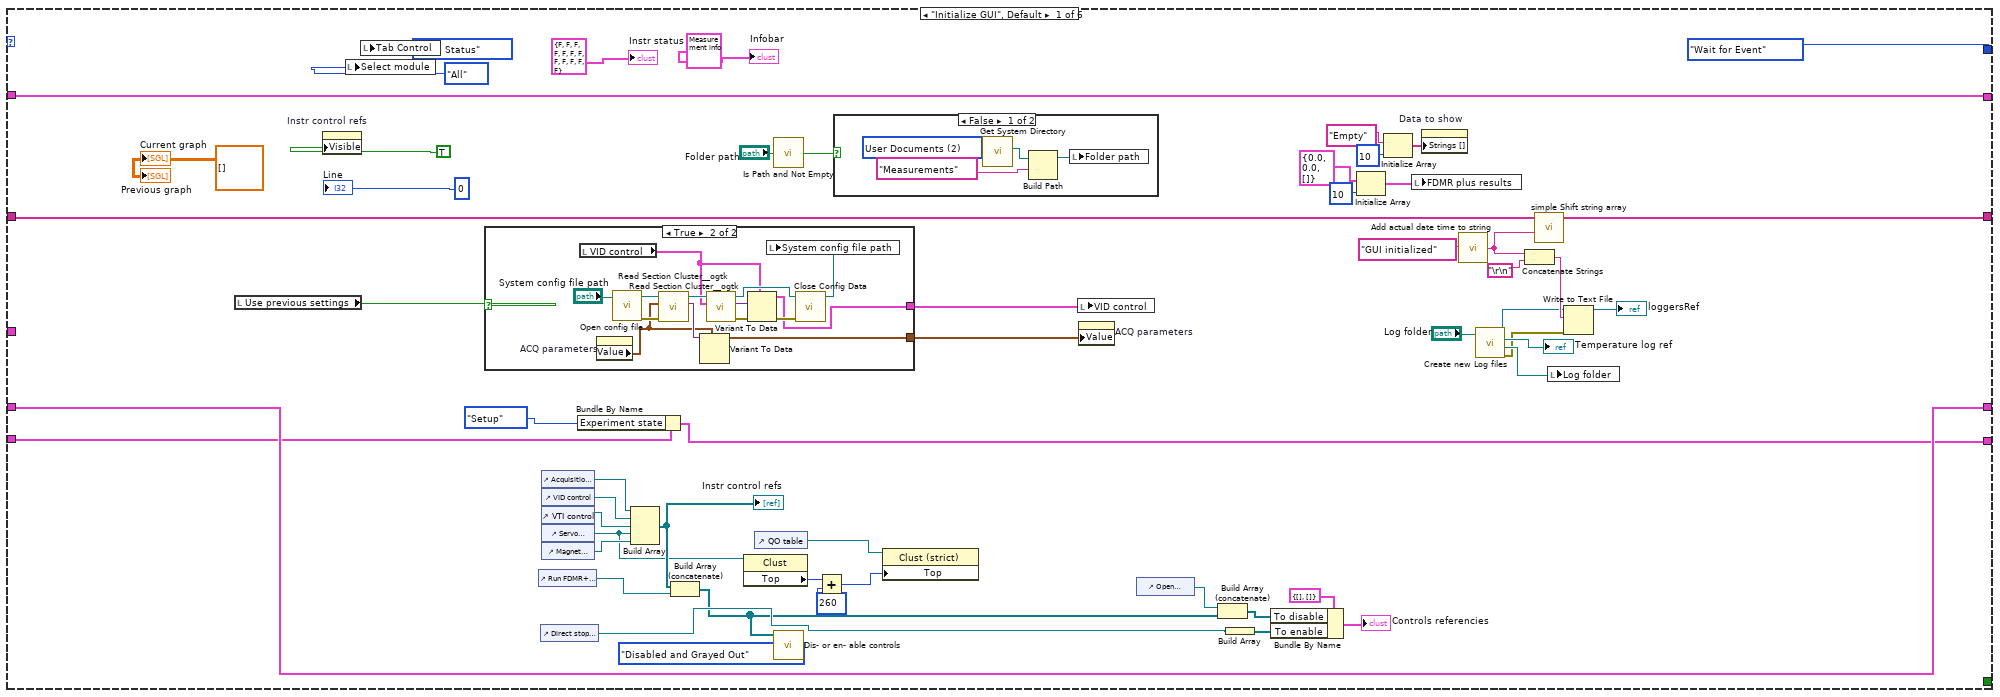
[diagram p3: hidden frame]
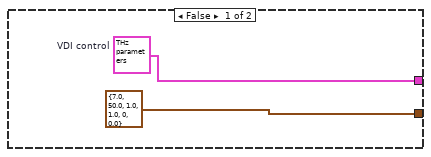
[diagram p5: hidden frame]
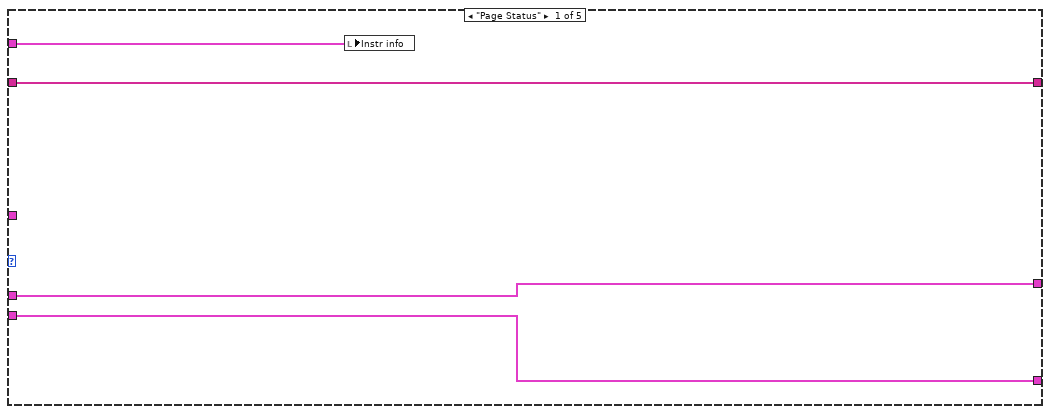
[diagram p6: hidden frame]
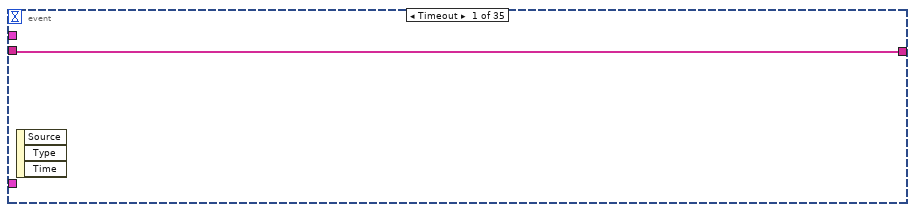
[diagram p7: hidden frame]
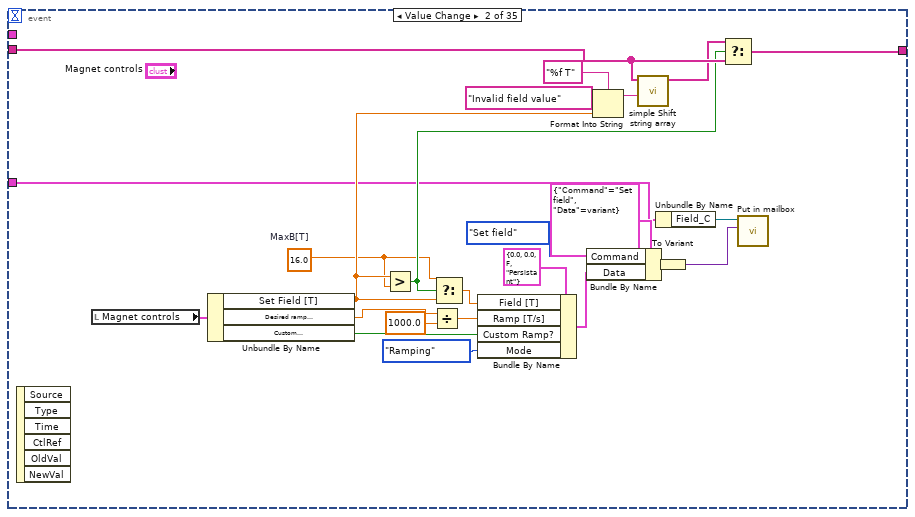
[diagram p8: hidden frame]
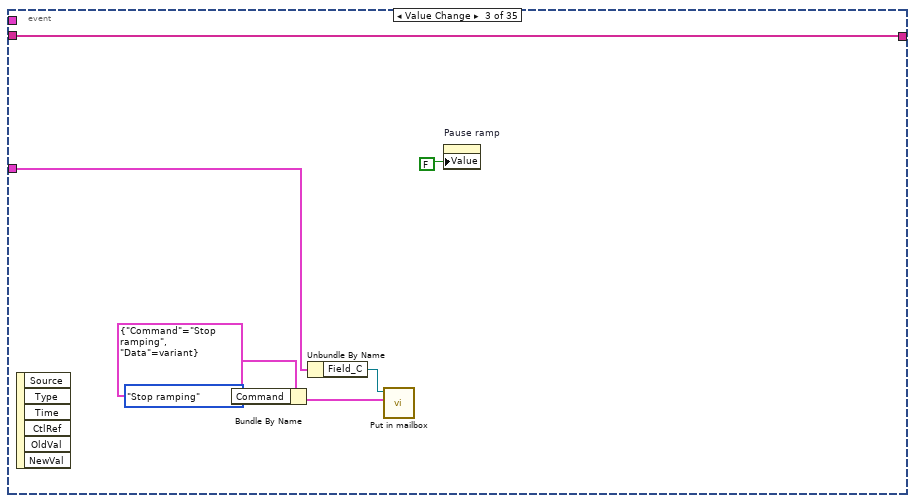
[diagram p9: hidden frame]
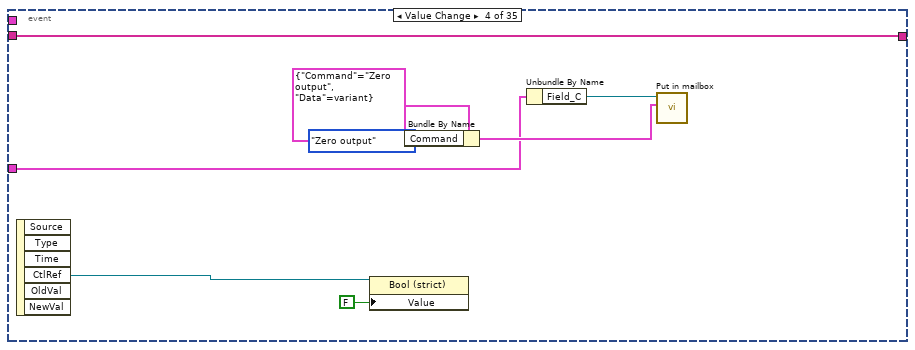
[diagram p10: hidden frame]
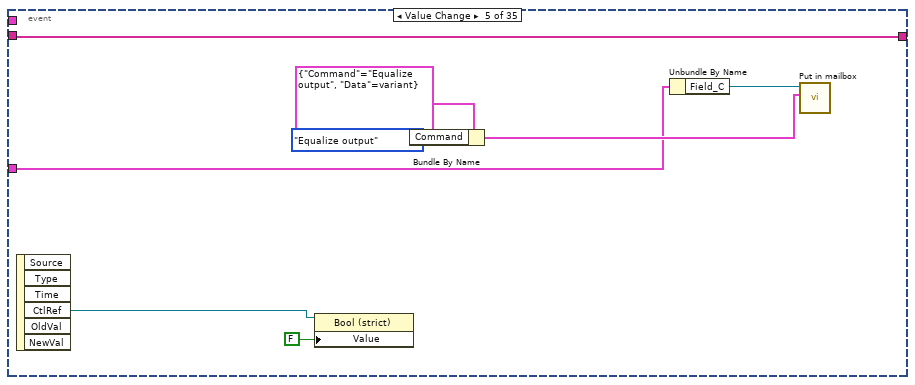
[diagram p11: hidden frame]
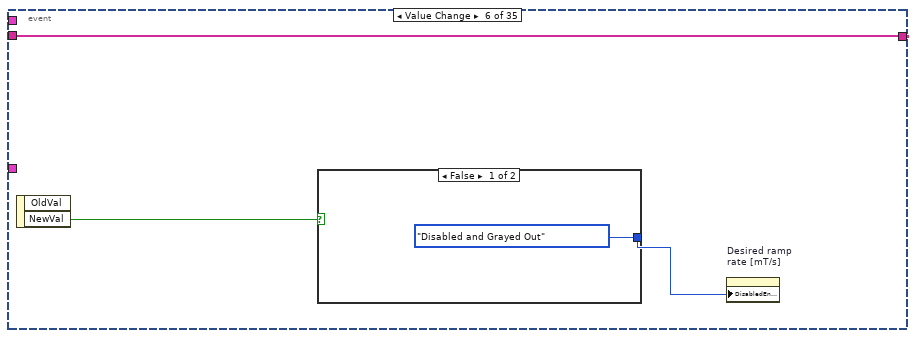
[diagram p12: hidden frame]
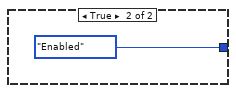
[diagram p13: hidden frame]
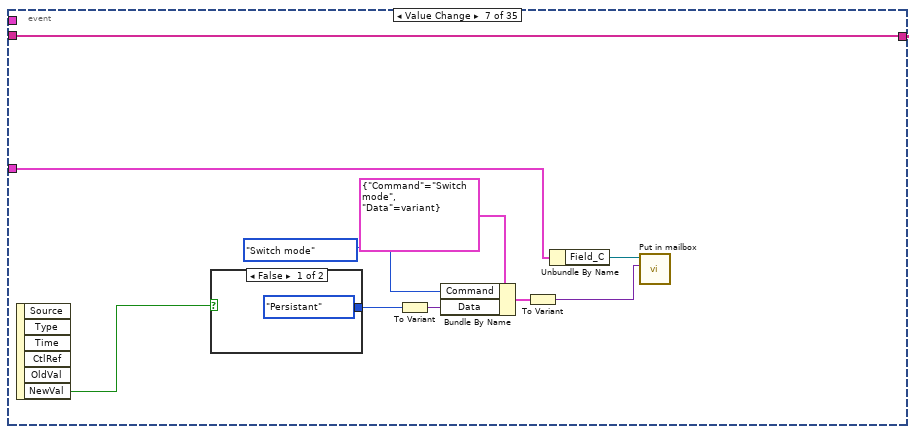
[diagram p14: hidden frame]
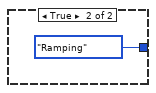
[diagram p15: hidden frame]
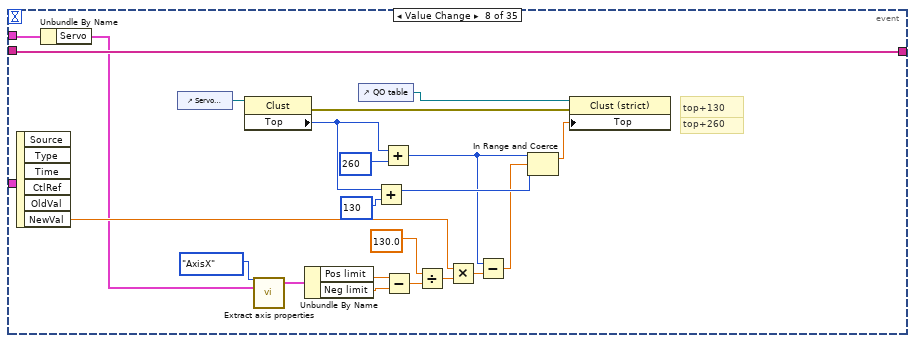
[diagram p16: hidden frame]
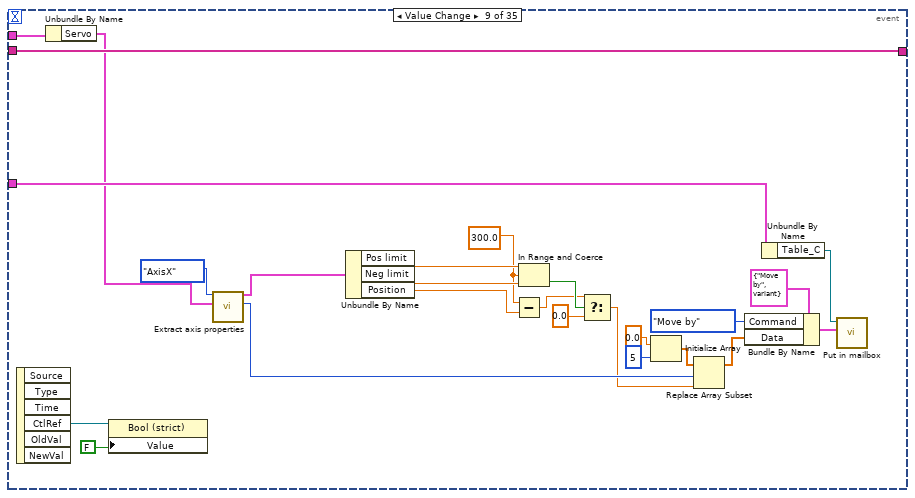
[diagram p17: hidden frame]
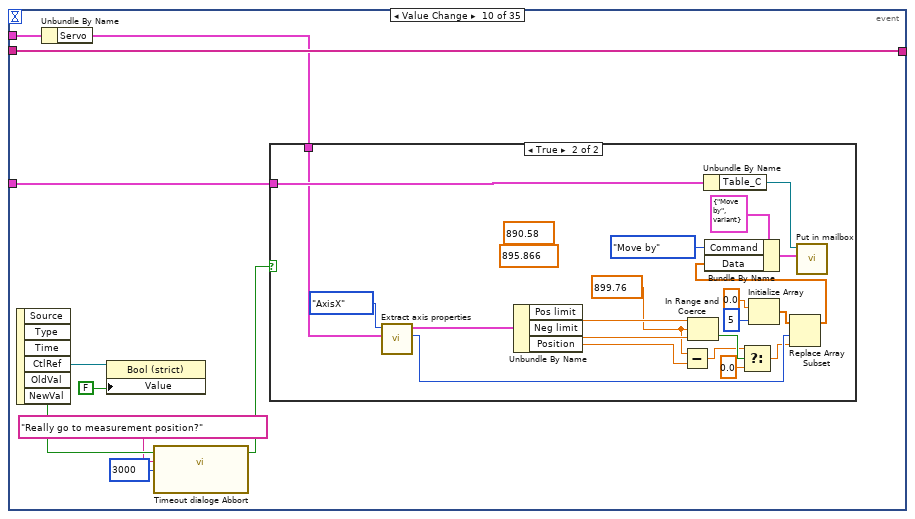
[diagram p18: hidden frame]
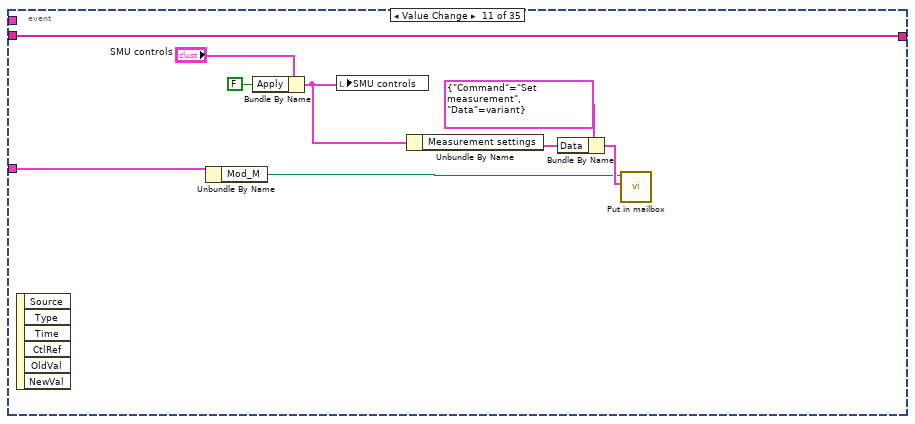
[diagram p20: hidden frame]
diagram:
  w4 = T27 {"Remains"=0.0, "T_sample [K]"=1.6, "Last log"="", "Experiment state"=enum."Setup", "Field [T]"=0.0, "Sample holder"=enum."Simple", "Started"=timestamp(0 s since 1904-01-01)}  # Infobar
  # "35,791394112"
  # "0.2796202665"
  # "0.559240533"
  # "468,75 kS/s"
  # "1,118481066 second for sweep"
  # "2,2369621333 second"
  # "4,473924266 sec"
  # "8 947,848533 sec"
  # "234.375 kS/s"
  # "117.1875 kS/s"
  # "29.296875 kS/s"
  # "58.59375 kS/s"
  # "17,895697056 sec"
  # "131072"
  # "8 947,848533 sec"
  # "1,8310546875 kS/s"
  # "3,662109375 ks/s"
  # "4,473924266 sec"
  # "2,2369621333 second"
  # "7,32421875 kS/s"
  # "1,118481066 second for sweep"
  # "16384 samples"
  # "14,6484375 kS/s"
  # "All modules requiere"
  n1 = call "Initialize Messenger.vi"() -> ("Referencies out"=w10:T31)  [unwired: 2 in, 1 out]
  n2 = Initialize Array("", 100 ("dimension size")) -> (w7:string[])
  n3 = while {
    tunnel: w10 -> [w25]
    shift-right: [w14] -> _
    shift-left: w7 -> [w24]
    shift-right: [w22] -> w5
    shift-left: TopStates."Initialize GUI" ("State") -> [w23]
    shift-right: [w20] -> _
    shift-left: _ -> [w19]
    shift-right: [w11] -> _
    shift-left: T25 {"F_start [GHz]"=380.0, "F_end [GHz]"=400.0, "Field [T]"=0.0, "Points [-]"=1, "Sampling Rate"=15, "ModA [G]"=100.0, "ModF [kHz]"=1.0, "Time const [ms]"=1.0, "Angle [°]"=-1.0, "Tmp [K]"=295.0, "Wait [min]"=1.0, "Repeat [-]"=8, "Comment"="", "Execute"=FALSE, "Auto-mod"=FALSE} ("Setup") -> [w17]
    shift-right: [w15] -> _
    shift-left: w4 -> [w16]
    shift-right: [w12] -> _
    shift-left: T8 {"Magnet"={"PSU"="None", "T monitor"="None", "Last update"=timestamp(0 s since 1904-01-01), "Field [T]"=0.0, "Ramp [mT/s]"=0.0, "Heater"=FALSE, "Ramp state"=enum."At Target"}, "MFLI"={"Lock-in"="None", "Multimeter"="None", "Last update"=timestamp(0 s since 1904-01-01), "Freq [kHz]"=0.0, "Ampl [mV]"=0.0, "OutEn"=FALSE, "In50 Ohm"=FALSE, "DemEn"=FALSE}, "THz"={"Name"="None", "Description"="None", "Last update"=timestamp(0 s since 1904-01-01), "Start [GHz]"=0.0, "Im Freq[MHz]"=0.0, "End [GHz]"=0.0}, "VTI"={"TempCtl"="None", "Last update"=timestamp(0 s since 1904-01-01), "VTI [K]"=0.0, "Sample [K]"=0.0, "Trap[K]"=0.0, "HePot [K]"=0.0, "Ambient [K]"=0.0}, "Rotator"={"Name"=3, "Last update"=timestamp(0 s since 1904-01-01), "Axes"=[]}, "Servo"=[{"Name"=enum."Unknown", "Last update"=timestamp(0 s since 1904-01-01), "Position"=0.0, "Pos limit"=0.0, "Neg limit"=0.0, "Power"=FALSE}], "SMU"={"Name"="", "Last update"=timestamp(0 s since 1904-01-01), "SourFunc"="", "SourValue"=0.0, "MeasFunc"="", "MeasValue"=0.0, "Output"=FALSE}, "PMD"={"Name"="", "Last update"=timestamp(0 s since 1904-01-01), "Position [°]"=0.0, "Speed"=0.0, "Desired [°]"=0.0, "Moving"=FALSE, "reserved"=0.0}, "PwrMonitor"={"Name"="", "Last update"=timestamp(0 s since 1904-01-01), "Outage?"=FALSE, "Low"=FALSE, "No battery"=FALSE, "Battery [%]"=0, "Charging"=FALSE}} ("Instr info") -> [w13]
    stop <- w21 stop-if-true
    # "new log"
    # "State Machine While Loop"
    n4 = case shown="\"Wait for Event\"" w23 {
      tunnel: w25 -> [_ w113 w1259 w2449 _ _]
      tunnel: w24 -> [w79 w112 w1273 w2448 w2762 _]
      tunnel: [w78 w101 w1272 w2447 w2761 w2767] -> w14
      tunnel: [TopStates."Wait for Event" ("State") TopStates."Check message" ("State") w1262 TopStates."Wait for Event" ("State") TopStates."Stop" ("State") TopStates."Initialize GUI" ("State")] -> w22
      tunnel: [_ w110 _ _ _ _] -> w21
      tunnel: [w67 w102 w1260 w2445 w2759 w2766] -> w11
      tunnel: w17 -> [w67 w108 w1260 w2446 w2759 w2766]
      tunnel: [w65 w103 w1261 w2441 w2758 w2765] -> w15
      tunnel: w16 -> [w66 w107 w1256 w2442 w2758 w2765]
      tunnel: w13 -> [w57 w104 w1258 w2440 w2757 w2764]
      tunnel: [w57 w104 w1257 w2440 w2757 w2764] -> w12
      frame "Initialize GUI", Default {
        w31 = sgl[][] [] ("Current graph")
        n5 = local read "Use previous settings"() -> (w51:bool)
        n6 = property on="Instr control refs" class="Arr (strict)"("Visible"=TRUE) -> ()  [unwired: 2 in, 2 out]
        n7 = local write "Select module"(T32."All" ("Module")) -> ()
        n8 = local write "Tab Control"(T6."Page Status" ("Tab Control")) -> ()
        n9 = case shown="True" w51 {
          tunnel: [w86 w88] -> w54
          tunnel: [T15 {"Filter order"=7.0, "Filter tau [ms]"=50.0, "F_Mod [kHz]"=1.0, "Amp_Mod [mV]"=1.0, "Enable output"=0, "Phase [°]"=0.0} ("ACQ parameters") w91] -> w50
          frame False {
            w86 = T17 {"AMC"=9, "Multip"=1, "Base frequency [GHz]"=90.0, "End frequency [GHz]"=90.0, "Im frequency [MHz]"=10.0, "Sweep up [ms]"=0.0, "Reset trigger?"=FALSE}  # VDI control
          }
          frame True {
            n10 = local read "VID control"() -> (w90:T17)
            n11 = property on="ACQ parameters" class="Clust (strict)"() -> ("Value"=w89:T15)  [unwired: 2 in, 2 out]
            n12 = call "Open config file.vi"("MAG config file path"="System config file path") -> ("error out"=w99:errorcluster, "Refnum out"=w100:T74)  [unwired: 7 in, 2 out]
            n13 = call <userlib>:"Read Section Cluster__ogtk.vi"("error in (no error)"=w99, "Section Formatted Cluster Type"=w89, "refnum"=w100) -> ("Section Formatted Cluster"=w98:variant, "dup refnum"=w95:T74)  [unwired: 4 in, 3 out]
            n14 = Variant To Data(type=w89, Variant=w98) -> (data=w91:T15)  [unwired: 1 in, 1 out]
            n15 = call <userlib>:"Read Section Cluster__ogtk.vi"("Section Formatted Cluster Type"=w90, "refnum"=w95) -> ("error out"=w97:errorcluster, "Section Formatted Cluster"=w96:variant, "dup refnum"=w94:T74)  [unwired: 5 in, 2 out]
            n16 = Variant To Data(error in=w97, type=w90, Variant=w96) -> (data=w88:T17, error out=w92:errorcluster)
            n17 = call <vilib>:"Close Config Data.vi"("error in (no error)"=w92, "refnum"=w94) -> ("file path"=w87:path)  [unwired: 8 in, 1 out]
            n18 = local write "System config file path"(w87) -> ()
          }
        }
        n19 = control-ref of="Run FDMR+ btn"() -> (w49:refnum<vi>)
        n20 = control-ref of="Direct stop meas. btn"() -> (w41:refnum<vi>)
        n21 = control-ref of="Acquisition controls"() -> (w69:refnum<vi>)
        n22 = control-ref of="VID control"() -> (w52:refnum<vi>)
        n23 = control-ref of="VTI control"() -> (w53:refnum<vi>)
        n24 = control-ref of="Servo controls"() -> (w58:refnum<vi>)
        n25 = control-ref of="Magnet controls"() -> (w68:refnum<vi>)
        n26 = Bundle By Name(cluster=w66, "Experiment state"=experiment_state."Setup" ("Value")) -> (w65:T27)
        n27 = Build Array(w69, w52, w53, w58, w68) -> (w59:refnum<vi>[])
        "Instr control refs" <- w59
        n28 = Build Array (concatenate)(w59, w49) -> (w37:refnum<vi>[])
        n29 = property class="Clust"(reference=w58) -> ("Top"=w62:i32)  [unwired: 1 in, 2 out]
        n30 = control-ref of="QO table"() -> (w61:refnum<vi>)
        n31 = call <vilib>:"Is Path and Not Empty.vi"("path"="Folder path") -> ("Is Path and Not Empty?"=w36:bool)  [unwired: 4 in]
        n32 = call "Dis- or en- able controls.vi"("Disabled"=T33."Disabled and Grayed Out", "Control referencies"=w37) -> ()  [unwired: 9 in, 1 out]
        n33 = Add(x=w62, y=260 ("Position:Top")) -> (x+y=w63:i32)
        n34 = case shown="False" w36 {
          frame False {
            w82 = T75 2 items=["User Home"=0, "User Desktop"=1, "User Documents"=2, "User Application Data"=3, "User Preferences"=4, "User Temporary"=5, "Public Documents"=6, "Public Application Data"=7, "Public Preferences"=8, "Public Cache"=13, "System Core Libraries"=9, "System Installed Libraries"=10, "Application Files"=11, "Boot Volume Root"=12] ("system directory type")
            n35 = call <vilib>:"Get System Directory.vi"("system directory type"=w82) -> ("system directory"=w84:path)  [unwired: 10 in]
            n36 = Build Path(base path=w84, name or relative path="Measurements") -> (appended path=w83:path)
            n37 = local write "Folder path"(w83) -> ()
          }
          frame True {
          }
        }
        n38 = property class="Clust (strict)"(reference=w61, "Top"=w63) -> ()  [unwired: 1 in, 2 out]
        n39 = local write "VID control"(w54) -> ()
        n40 = property on="ACQ parameters" class="Clust (strict)"("Value"=w50) -> ()  [unwired: 2 in, 2 out]
        n41 = control-ref of="Open measurement"() -> (w38:refnum<vi>)
        n42 = Build Array (concatenate)(w38, w37) -> (w39:refnum<vi>[])
        n43 = Build Array(w41) -> (w40:refnum<vi>[])
        n44 = Bundle By Name(cluster=T4 {"To disable"=[], "To enable"=[]} ("Controls referencies"), "To disable"=w39, "To enable"=w40) -> (→"Controls referencies":T4)
        n45 = Initialize Array(T3 {"StartF[GHz]"=0.0, "EndF[GHz]"=0.0, "aver Data"=[]} ("Cluster"), 10 ("dimension size")) -> (w34:T3[])
        n46 = Initialize Array("Empty", 10 ("dimension size")) -> (w45:string[])
        n47 = local write "FDMR plus results"(w34) -> ()
        n48 = property on="Data to show" class="Ring (strict)"("Strings []"=w45) -> ()  [unwired: 2 in, 2 out]
        n49 = call "Add actual date time to string.vi"("String in"="GUI initialized") -> ("String out"=w74:string)  [unwired: 4 in]
        n50 = call "Create new Log files.vi"("Log folder"="Log folder") -> ("error out"=w26:errorcluster, "dup path"=w27:path, "tmp logfile out"=→"Temperature log ref":refnum<file>, "event logfile out"=w29:refnum<file>)  [unwired: 7 in]
        n51 = Concatenate Strings(w74, "\r\n") -> (w73:string)
        n52 = call "simple Shift string array.vi"("Element in"=w74, "Array in"=w79) -> ("Array out"=w78:string[])  [unwired: 8 in, 1 out]
        n53 = local write "Log folder"(w27) -> ()
        n54 = Write to Text File(file (use dialog)=w29, text=w73, error in=w26) -> (refnum out=→"loggersRef":refnum<file>)  [unwired: 1 in, 2 out]
        "Instr status" <- T1 {"Mag"=FALSE, "Rot"=FALSE, "VTI"=FALSE, "MFLI"=FALSE, "Serv"=FALSE, "THz"=FALSE, "ADQ7"=FALSE, "SMU"=FALSE, "PMD"=FALSE, "UPS"=FALSE, "DMM"=FALSE, "abc"=FALSE} ("Instruments status 2")
        "Infobar" <- T27 {"Remains"=0.0, "T_sample [K]"=0.0, "Last log"="", "Experiment state"=enum."Setup", "Field [T]"=0.0, "Sample holder"=enum."Simple", "Started"=timestamp(0 s since 1904-01-01)} ("Infobar")
        "Line" <- 0 ("Line")
        "Current graph" <- w31
        "Previous graph" <- w31
      }
      frame "Wait for Event" {
        n55 = event shown="[0] Timeout" {
          selector: _ -> [_ _ _ _ _]
          dyn-events: _ -> [_ _ _ _ _]
          timeout: 5 -> [_ _ _ _ _]
          tunnel: w112 -> [w120 w987 w997 w1069 w1153]
          tunnel: [w122 w987 w997 w1069 w1152] -> w101
          tunnel: w113 -> [w115 _ w991 w1071 w1154]
          tunnel: [_ _ _ w1070 _] -> w110
          tunnel: [w119 w990 w996 w1068 w1151] -> w102
          tunnel: w108 -> [w118 w990 w996 w1068 w1151]
          tunnel: [w117 w989 w995 w1067 w1150] -> w105
          tunnel: w107 -> [w116 w989 w995 w1067 w1150]
          tunnel: w104 -> [w114 _ _ _ _]
          event Timeout {
            n56 = event-data() -> ()  [unwired: 1 in, 3 out]
            n57 = case shown="\"Adjustment\", Default" "Tab Control" {
              tunnel: [w126 w133 w810 w890 w933] -> w122
              tunnel: w120 -> [w126 w131 w811 w891 w933]
              tunnel: w115 -> [_ w130 w808 w888 _]
              tunnel: [w125 w129 w807 w887 w932] -> w119
              tunnel: w118 -> [w125 w129 w806 w886 w932]
              tunnel: [w124 w128 w804 w884 w931] -> w117
              tunnel: w116 -> [w124 w128 w805 w885 w931]
              tunnel: w114 -> [w123 w127 _ _ _]
              frame "Page Status" {
                n58 = local write "Instr info"(w123) -> ()
              }
              frame "Adjustment", Default {
                n59 = event shown="[33] \"VTI control.VTI space [K]\", \"VTI control.Sample [K]\", \"VTI control.Heater3 [K]\", \"VTI control.Heater4 [K]\": Value Change" {
                  selector: _ -> [_ _ _ _ _ _ _ _ _ _ _ _ _ _ _ _ _ _ _ _ _ _ _ _ _ _ _ _ _ _ _ _ _ _ _]
                  dyn-events: _ -> [_ _ _ _ _ _ _ _ _ _ _ _ _ _ _ _ _ _ _ _ _ _ _ _ _ _ _ _ _ _ _ _ _ _ _]
                  timeout: 0 -> [_ _ _ _ _ _ _ _ _ _ _ _ _ _ _ _ _ _ _ _ _ _ _ _ _ _ _ _ _ _ _ _ _ _ _]
                  tunnel: w131 -> [w134 w150 w165 w173 w181 w182 w191 w201 w245 w255 w285 w291 w297 w305 w319 w344 w370 w400 w435 w480 w509 w534 w560 w585 w611 w636 w666 w681 w689 w711 w720 w735 w784 w795 w801]
                  tunnel: [w134 w154 w165 w173 w181 w182 w191 w201 w245 w255 w285 w291 w297 w305 w319 w344 w370 w400 w435 w480 w509 w534 w560 w585 w611 w636 w666 w681 w689 w711 w720 w735 w784 w795 w801] -> w133
                  tunnel: w130 -> [_ w140 w159 w168 w176 _ w187 _ w235 w252 w277 w288 w294 w302 w310 w335 w361 w386 w411 w455 w500 w525 w551 w576 w602 w627 w650 w669 w687 w702 _ w734 w783 w794 _]
                  tunnel: w127 -> [_ _ _ _ _ _ _ w200 w222 w247 _ _ _ _ w307 w331 w357 w382 w408 w451 w497 w521 w547 w572 w598 w623 w649 _ _ _ _ _ _ _ _]
                  event Timeout {
                    (unwired) TopStates."Check message" ("State")
                    n60 = event-data() -> ()  [unwired: 1 in, 3 out]
                  }
                  event Value Change {
                    w135 = 16.0  # MaxB[T]
                    n61 = event-data() -> ()  [unwired: 1 in, 6 out]
                    n62 = local read "Magnet controls"() -> (w156:T19)
                    n63 = Unbundle By Name(w156) -> ("Set Field [T]"=w147:dbl, "Desired ramp\nrate [mT/s]"=w137:dbl, "Custom\nramp"=w143:bool)
                    n64 = Greater?(x=w147, y=w135) -> (0:w148:bool)
                    n65 = Divide(x=w137, y=1000.0) -> (x/y=w138:dbl)
                    n66 = Select(t=w135, s=w148, f=w147) -> (s? t:f=w145:dbl)
                    n67 = Bundle By Name(cluster=T35 {"Field [T]"=0.0, "Ramp [T/s]"=0.0, "Custom Ramp?"=FALSE, "Mode"=enum."Persistant"} ("Set Field"), "Field [T]"=w145, "Ramp [T/s]"=w138, "Custom Ramp?"=w143, "Mode"=Magnet_mode_public."Ramping") -> (w144:T35)
                    n68 = Bundle By Name(cluster=T37 {"Command"=enum."Set field", "Data"=variant(enum16{"Ramping", "Perzistant"} enum."Ramping")} ("MSG to magnet"), "Command"=Magnet_Orders."Set field" ("Order"), "Data"=w144) -> (w158:T37)
                    n69 = Format Into String(format string="%f T", initial string="Invalid field value" ("Element in"), w147) -> (resulting string=w151:string)  [unwired: 1 in, 1 out]
                    n70 = call "simple Shift string array.vi"("Element in"=w151, "Array in"=w150) -> ("Array out"=w149:string[])  [unwired: 8 in, 1 out]
                    n71 = Unbundle By Name(w140) -> ("Field_C"=w142:refnum<queue>)
                    n72 = To Variant(anything=w158) -> (Variant=w141:variant)
                    n73 = Select(t=w149, s=w148, f=w150) -> (s? t:f=w154:string[])
                    n74 = call "Put in mailbox.vi"("Message"=w141, "Queue in"=w142) -> ()  [unwired: 7 in, 3 out]
                  }
                  event Value Change {
                    n75 = event-data() -> ()  [unwired: 1 in, 6 out]
                    n76 = Bundle By Name(cluster=T37 {"Command"=enum."Stop ramping", "Data"=variant(enum16{"Ramping", "Perzistant"} enum."Ramping")} ("MSG to magnet"), "Command"=Magnet_Orders."Stop ramping" ("Order")) -> (w162:T37)
                    n77 = Unbundle By Name(w159) -> ("Field_C"=w163:refnum<queue>)
                    n78 = call "Put in mailbox.vi"("Message"=w162, "Queue in"=w163) -> ()  [unwired: 7 in, 3 out]
                    n79 = property on="Pause ramp" class="Bool (strict)"("Value"=FALSE) -> ()  [unwired: 2 in, 2 out]
                  }
                  event Value Change {
                    n80 = event-data() -> ("CtlRef"=w167:refnum<vi>)  [unwired: 1 in, 5 out]
                    n81 = property class="Bool (strict)"(reference=w167, "Value"=FALSE) -> ()  [unwired: 1 in, 2 out]
                    n82 = Bundle By Name(cluster=T37 {"Command"=enum."Zero output", "Data"=variant(enum16{"Ramping", "Perzistant"} enum."Ramping")} ("MSG to magnet"), "Command"=Magnet_Orders."Zero output" ("Order")) -> (w169:T37)
                    n83 = Unbundle By Name(w168) -> ("Field_C"=w170:refnum<queue>)
                    n84 = call "Put in mailbox.vi"("Message"=w169, "Queue in"=w170) -> ()  [unwired: 7 in, 3 out]
                  }
                  event Value Change {
                    n85 = event-data() -> ("CtlRef"=w174:refnum<vi>)  [unwired: 1 in, 5 out]
                    n86 = property class="Bool (strict)"(reference=w174, "Value"=FALSE) -> ()  [unwired: 1 in, 2 out]
                    n87 = Bundle By Name(cluster=T37 {"Command"=enum."Equalize output", "Data"=variant(enum16{"Ramping", "Perzistant"} enum."Ramping")} ("MSG to magnet"), "Command"=Magnet_Orders."Equalize output" ("Order")) -> (w177:T37)
                    n88 = Unbundle By Name(w176) -> ("Field_C"=w178:refnum<queue>)
                    n89 = call "Put in mailbox.vi"("Message"=w177, "Queue in"=w178) -> ()  [unwired: 7 in, 3 out]
                  }
                  event Value Change {
                    n90 = event-data() -> ("NewVal"=w184:bool)  [unwired: 1 in, 1 out]
                    n91 = case shown="False" w184 {
                      tunnel: [T33."Disabled and Grayed Out" ("Disabled") T33."Enabled" ("Disabled")] -> w183
                      frame False {
                      }
                      frame True {
                      }
                    }
                    n92 = property on="Desired ramp\nrate [mT/s]" class="DigNum (strict)"("DisabledEnum"=w183) -> ()  [unwired: 2 in, 2 out]
                  }
                  event Value Change {
                    n93 = event-data() -> ("NewVal"=w192:bool)  [unwired: 1 in, 5 out]
                    n94 = case shown="False" w192 {
                      tunnel: [Magnet_mode_public."Persistant" ("Operation mode") Magnet_mode_public."Ramping" ("Operation mode")] -> w193
                      frame False {
                      }
                      frame True {
                      }
                    }
                    n95 = To Variant(anything=w193) -> (Variant=w190:variant)
                    n96 = Bundle By Name(cluster=T37 {"Command"=enum."Switch mode", "Data"=variant(enum16{"Ramping", "Perzistant"} enum."Ramping")} ("MSG to magnet"), "Command"=Magnet_Orders."Switch mode" ("Order"), "Data"=w190) -> (w196:T37)
                    n97 = To Variant(anything=w196) -> (Variant=w188:variant)
                    n98 = Unbundle By Name(w187) -> ("Field_C"=w189:refnum<queue>)
                    n99 = call "Put in mailbox.vi"("Message"=w188, "Queue in"=w189) -> ()  [unwired: 7 in, 3 out]
                  }
                  event Value Change {
                    # "top+260"
                    # "top+130"
                    n100 = event-data() -> ("NewVal"=w212:dbl)  [unwired: 1 in, 5 out]
                    n101 = Unbundle By Name(w200) -> ("Servo"=w199:T10[])
                    n102 = control-ref of="Servo controls"() -> (w220:refnum<vi>)
                    n103 = property class="Clust"(reference=w220) -> (error out=w211:errorcluster, "Top"=w206:i32)  [unwired: 1 in, 1 out]
                    n104 = call "Extract axis properties.vi"("Name"=Axis_names."AxisX", "All servo status"=w199) -> ("Servo"=w217:T10)  [unwired: 6 in, 2 out]
                    n105 = Unbundle By Name(w217) -> ("Pos limit"=w215:dbl, "Neg limit"=w214:dbl)
                    n106 = control-ref of="QO table"() -> (w216:refnum<vi>)
                    n107 = Add(x=w206, y=130) -> (x+y=w208:i32)
                    n108 = Add(x=w206, y=260) -> (x+y=w205:i32)
                    n109 = Subtract(x=w215, y=w214) -> (x-y=w202:dbl)
                    n110 = Divide(x=130.0 ("y"), y=w202) -> (x/y=w213:dbl)
                    n111 = Multiply(x=w212, y=w213) -> (x*y=w209:dbl)
                    n112 = Subtract(x=w205, y=w209) -> (x-y=w204:dbl)
                    n113 = In Range and Coerce(upper limit=w205, x=w204, lower limit=w208) -> (coerced(x)=w219:dbl)  [unwired: 1 out]
                    n114 = property class="Clust (strict)"(reference=w216, error in=w211, "Top"=w219) -> ()  [unwired: 2 out]
                  }
                  event Value Change {
                    w227 = 300.0 ("x")
                    n115 = event-data() -> ("CtlRef"=w244:refnum<vi>)  [unwired: 1 in, 5 out]
                    n116 = Unbundle By Name(w222) -> ("Servo"=w221:T10[])
                    n117 = property class="Bool (strict)"(reference=w244, "Value"=FALSE) -> ()  [unwired: 1 in, 2 out]
                    n118 = call "Extract axis properties.vi"("Name"=Axis_names."AxisX", "All servo status"=w221) -> ("Servo"=w242:T10, "Index"=w233:i32)  [unwired: 6 in, 1 out]
                    n119 = Unbundle By Name(w242) -> ("Pos limit"=w229:dbl, "Neg limit"=w228:dbl, "Position"=w230:dbl)
                    n120 = Subtract(x=w227, y=w230) -> (x-y=w224:dbl)
                    n121 = In Range and Coerce(upper limit=w229, x=w227, lower limit=w228) -> (In Range?=w226:bool)  [unwired: 1 out]
                    n122 = Select(t=w224, s=w226, f=0.0) -> (s? t:f=w223:dbl)
                    n123 = Initialize Array(0.0 ("element"), 5 ("dimension size")) -> (w231:dbl[])
                    n124 = Replace Array Subset(array=w231, new element=w223, index=w233) -> (w232:dbl[])
                    n125 = Bundle By Name(cluster=T39 {"Command"=enum."Move by", "Data"=variant(dbl[] [])} ("MSG to Servo"), "Command"=Servo_commands."Move by", "Data"=w232) -> (w234:T39)
                    n126 = Unbundle By Name(w235) -> ("Table_C"=w236:refnum<queue>)
                    n127 = call "Put in mailbox.vi"("Message"=w234, "Queue in"=w236) -> ()  [unwired: 7 in, 3 out]
                  }
                  event Value Change {
                    n128 = event-data() -> ("CtlRef"=w254:refnum<vi>, "NewVal"=w251:bool)  [unwired: 1 in, 4 out]
                    n129 = Unbundle By Name(w247) -> ("Servo"=w246:T10[])
                    n130 = property class="Bool (strict)"(reference=w254, "Value"=FALSE) -> ()  [unwired: 1 in, 2 out]
                    n131 = call "Timeout dialoge Abbort.vi"("Enable"=w251, "Message to Display"="Really go to measurement position?", "timeout[ms]"=u32 3000) -> ("Yes"=w248:bool)  [unwired: 15 in, 1 out]
                    n132 = case shown="True" w248 {
                      tunnel: w252 -> [_ w269]
                      tunnel: w246 -> [_ w257]
                      frame False {
                      }
                      frame True {
                        w256 = 899.76 ("x")
                        (unwired) 890.58 ("x")
                        (unwired) 895.866 ("x")
                        n133 = call "Extract axis properties.vi"("Name"=Axis_names."AxisX", "All servo status"=w257) -> ("Servo"=w276:T10, "Index"=w267:i32)  [unwired: 6 in, 1 out]
                        n134 = Unbundle By Name(w276) -> ("Pos limit"=w263:dbl, "Neg limit"=w262:dbl, "Position"=w264:dbl)
                        n135 = Subtract(x=w256, y=w264) -> (x-y=w259:dbl)
                        n136 = In Range and Coerce(upper limit=w263, x=w256, lower limit=w262) -> (In Range?=w261:bool)  [unwired: 1 out]
                        n137 = Unbundle By Name(w269) -> ("Table_C"=w270:refnum<queue>)
                        n138 = Select(t=w259, s=w261, f=0.0) -> (s? t:f=w258:dbl)
                        n139 = Initialize Array(0.0 ("element"), 5 ("dimension size")) -> (w265:dbl[])
                        n140 = Replace Array Subset(array=w265, new element=w258, index=w267) -> (w266:dbl[])
                        n141 = Bundle By Name(cluster=T39 {"Command"=enum."Move by", "Data"=variant(dbl[] [])} ("MSG to Servo"), "Command"=Servo_commands."Move by", "Data"=w266) -> (w268:T39)
                        n142 = call "Put in mailbox.vi"("Message"=w268, "Queue in"=w270) -> ()  [unwired: 7 in, 3 out]
                      }
                    }
                  }
                  event "SMU controls.Apply": Value Change {
                    n143 = event-data() -> ()  [unwired: 1 in, 6 out]
                    n144 = Unbundle By Name(w277) -> ("Mod_M"=w280:refnum<queue>)
                    n145 = Bundle By Name(cluster="SMU controls", "Apply"=FALSE) -> (w281:T21)
                    n146 = local write "SMU controls"(w281) -> ()
                    n147 = Unbundle By Name(w281) -> ("Measurement settings"=w284:T20)
                    n148 = Bundle By Name(cluster=T40 {"Command"=enum."Set measurement", "Data"=variant} ("MSG to Source meter"), "Data"=w284) -> (w283:T40)
                    n149 = call "Put in mailbox.vi"("Message"=w283, "Queue in"=w280) -> ()  [unwired: 7 in, 3 out]
                  }
                  event "SMU controls.Record": Value Change {
                    n150 = event-data() -> ("CtlRef"=w287:refnum<vi>)  [unwired: 1 in, 5 out]
                    n151 = property class="Bool (strict)"(reference=w287, "Value"=FALSE) -> ()  [unwired: 1 in, 2 out]
                    n152 = Unbundle By Name(w288) -> ("Mod_M"=w289:refnum<queue>)
                    n153 = call "Put in mailbox.vi"("Message"=T40 {"Command"=enum."Start measurement", "Data"=variant} ("MSG to Source meter"), "Queue in"=w289) -> ()  [unwired: 7 in, 3 out]
                  }
                  event "SMU controls.Stop": Value Change {
                    n154 = event-data() -> ("CtlRef"=w293:refnum<vi>)  [unwired: 1 in, 5 out]
                    n155 = property class="Bool (strict)"(reference=w293, "Value"=FALSE) -> ()  [unwired: 1 in, 2 out]
                    n156 = Unbundle By Name(w294) -> ("Mod_M"=w295:refnum<queue>)
                    n157 = call "Put in mailbox.vi"("Message"=T40 {"Command"=enum."Stop measurement", "Data"=variant} ("MSG to Source meter"), "Queue in"=w295) -> ()  [unwired: 7 in, 3 out]
                  }
                  event Value Change {
                    n158 = event-data() -> ("CtlRef"=w304:refnum<vi>)  [unwired: 1 in, 5 out]
                    n159 = property class="Bool"(reference=w304, "Value"=FALSE) -> ()  [unwired: 1 in, 2 out]
                    n160 = Unbundle By Name(w302) -> ("Table_C"=w299:refnum<queue>)
                    n161 = Bundle By Name(cluster=T39 {"Command"=enum."Stop", "Data"=variant(dbl[] [])} ("MSG to Servo"), "Command"=Servo_commands."Stop") -> (w298:T39)
                    n162 = call "Put in mailbox.vi"("Message"=w298, "Queue in"=w299) -> ()  [unwired: 7 in, 3 out]
                  }
                  event Value Change {
                    # "X position limit"
                    n163 = event-data() -> ("CtlRef"=w308:refnum<vi>)  [unwired: 1 in, 5 out]
                    n164 = Unbundle By Name(w307) -> ("Servo"=w306:T10[])
                    n165 = call "Extract axis properties.vi"("Name"=Axis_names."AxisX", "All servo status"=w306) -> ("Servo"=w316:T10, "Index"=w313:i32)  [unwired: 6 in, 1 out]
                    n166 = Unbundle By Name(w316) -> ("Position"=w311:dbl, "Pos limit"=w314:dbl)
                    n167 = property on="Step\n[mm]" class="DigNum (strict)"() -> ("Value"=w312:dbl)  [unwired: 2 in, 2 out]
                    n168 = Subtract(x=w314, y=w312) -> (x-y=w318:dbl)
                    n169 = Less?(x=w311, y=w318) -> (x < y?=w317:bool)
                    n170 = case shown="True" w317 {
                      tunnel: w312 -> [_ w328]
                      tunnel: w313 -> [_ w324]
                      tunnel: w310 -> [_ w321]
                      frame False {
                      }
                      frame True {
                        n171 = Initialize Array(0.0 ("element"), 5 ("dimension size")) -> (w329:dbl[])
                        n172 = Replace Array Subset(array=w329, new element=w328, index=w324) -> (w325:dbl[])
                        n173 = Bundle By Name(cluster=T39 {"Command"=enum."Move by", "Data"=variant(dbl[] [])} ("MSG to Servo"), "Command"=Servo_commands."Move by", "Data"=w325) -> (w322:T39)
                        n174 = Unbundle By Name(w321) -> ("Table_C"=w323:refnum<queue>)
                        n175 = call "Put in mailbox.vi"("Message"=w322, "Queue in"=w323) -> ()  [unwired: 7 in, 3 out]
                      }
                    }
                    n176 = property class="Bool (strict)"(reference=w308, "Value"=FALSE) -> ()  [unwired: 1 in, 2 out]
                  }
                  event Value Change {
                    n177 = event-data() -> ("CtlRef"=w333:refnum<vi>)  [unwired: 1 in, 5 out]
                    n178 = Unbundle By Name(w331) -> ("Servo"=w332:T10[])
                    n179 = call "Extract axis properties.vi"("Name"=Axis_names."AxisX", "All servo status"=w332) -> ("Servo"=w341:T10, "Index"=w338:i32)  [unwired: 6 in, 1 out]
                    n180 = Unbundle By Name(w341) -> ("Position"=w336:dbl, "Neg limit"=w339:dbl)
                    n181 = property class="Bool (strict)"(reference=w333, "Value"=FALSE) -> ()  [unwired: 1 in, 2 out]
                    n182 = property on="Step\n[mm]" class="DigNum (strict)"() -> ("Value"=w337:dbl)  [unwired: 2 in, 2 out]
                    n183 = Add(x=w339, y=w337) -> (x+y=w342:dbl)
                    n184 = Greater?(x=w336, y=w342) -> (0:w343:bool)
                    n185 = case shown="True" w343 {
                      tunnel: w337 -> [_ w353]
                      tunnel: w338 -> [_ w349]
                      tunnel: w335 -> [_ w346]
                      frame False {
                      }
                      frame True {
                        n186 = Negate(x=w353) -> (-x=w355:dbl)
                        n187 = Initialize Array(0.0 ("element"), 5 ("dimension size")) -> (w354:dbl[])
                        n188 = Replace Array Subset(array=w354, new element=w355, index=w349) -> (w350:dbl[])
                        n189 = Unbundle By Name(w346) -> ("Table_C"=w347:refnum<queue>)
                        n190 = Bundle By Name(cluster=T39 {"Command"=enum."Move by", "Data"=variant(dbl[] [])} ("MSG to Servo"), "Command"=Servo_commands."Move by", "Data"=w350) -> (w345:T39)
                        n191 = call "Put in mailbox.vi"("Message"=w345, "Queue in"=w347) -> ()  [unwired: 7 in, 3 out]
                      }
                    }
                  }
                  event Value Change {
                    w367 = 0.5 ("y")
                    n192 = event-data() -> ("CtlRef"=w359:refnum<vi>)  [unwired: 1 in, 5 out]
                    n193 = Unbundle By Name(w357) -> ("Servo"=w358:T10[])
                    n194 = call "Extract axis properties.vi"("Name"=Axis_names."AxisY", "All servo status"=w358) -> ("Servo"=w366:T10, "Index"=w363:i32)  [unwired: 6 in, 1 out]
                    n195 = Unbundle By Name(w366) -> ("Position"=w362:dbl, "Pos limit"=w364:dbl)
                    n196 = Subtract(x=w364, y=w367) -> (x-y=w368:dbl)
                    n197 = Less?(x=w362, y=w368) -> (x < y?=w369:bool)
                    n198 = case shown="True" w369 {
                      tunnel: w367 -> [_ w379]
                      tunnel: w363 -> [_ w375]
                      tunnel: w361 -> [_ w371]
                      frame False {
                      }
                      frame True {
                        n199 = Initialize Array(0.0 ("element"), 5 ("dimension size")) -> (w380:dbl[])
                        n200 = Replace Array Subset(array=w380, new element=w379, index=w375) -> (w376:dbl[])
                        n201 = Bundle By Name(cluster=T39 {"Command"=enum."Move by", "Data"=variant(dbl[] [])} ("MSG to Servo"), "Command"=Servo_commands."Move by", "Data"=w376) -> (w372:T39)
                        n202 = Unbundle By Name(w371) -> ("Table_C"=w373:refnum<queue>)
                        n203 = call "Put in mailbox.vi"("Message"=w372, "Queue in"=w373) -> ()  [unwired: 7 in, 3 out]
                      }
                    }
                    n204 = property class="Bool (strict)"(reference=w359, "Value"=FALSE) -> ()  [unwired: 1 in, 2 out]
                  }
                  event Value Change {
                    w393 = 0.5 ("y")
                    n205 = event-data() -> ("CtlRef"=w384:refnum<vi>)  [unwired: 1 in, 5 out]
                    n206 = Unbundle By Name(w382) -> ("Servo"=w383:T10[])
                    n207 = call "Extract axis properties.vi"("Name"=Axis_names."AxisY", "All servo status"=w383) -> ("Servo"=w391:T10, "Index"=w388:i32)  [unwired: 6 in, 1 out]
                    n208 = Unbundle By Name(w391) -> ("Position"=w387:dbl, "Neg limit"=w390:dbl)
                    n209 = property class="Bool (strict)"(reference=w384, "Value"=FALSE) -> ()  [unwired: 1 in, 2 out]
                    n210 = Add(x=w390, y=w393) -> (x+y=w392:dbl)
                    n211 = Negate(x=w393) -> (-x=w394:dbl)
                    n212 = Initialize Array(0.0 ("element"), 5 ("dimension size")) -> (w398:dbl[])
                    n213 = Greater?(x=w387, y=w392) -> (0:w399:bool)
                    n214 = Replace Array Subset(array=w398, new element=w394, index=w388) -> (w395:dbl[])
                    n215 = case shown="True" w399 {
                      tunnel: w395 -> [_ w405]
                      tunnel: w386 -> [_ w402]
                      frame False {
                      }
                      frame True {
                        n216 = Unbundle By Name(w402) -> ("Table_C"=w403:refnum<queue>)
                        n217 = Bundle By Name(cluster=T39 {"Command"=enum."Move by", "Data"=variant(dbl[] [])} ("MSG to Servo"), "Command"=Servo_commands."Move by", "Data"=w405) -> (w401:T39)
                        n218 = call "Put in mailbox.vi"("Message"=w401, "Queue in"=w403) -> ()  [unwired: 7 in, 3 out]
                      }
                    }
                  }
                  event Value Change {
                    w430 = 0.5 ("y")
                    n219 = event-data() -> ("CtlRef"=w409:refnum<vi>)  [unwired: 1 in, 5 out]
                    n220 = Unbundle By Name(w408) -> ("Servo"=w407:T10[])
                    n221 = call "Extract axis properties.vi"("Name"=Axis_names."AxisZ_right", "All servo status"=w407) -> ("Servo"=w428:T10, "Index"=w419:i32)  [unwired: 6 in, 1 out]
                    n222 = call "Extract axis properties.vi"("Name"=Axis_names."AxisZ_middle", "All servo status"=w407) -> ("Servo"=w427:T10, "Index"=w418:i32)  [unwired: 6 in, 1 out]
                    n223 = call "Extract axis properties.vi"("Name"=Axis_names."AxisZ_left", "All servo status"=w407) -> ("Servo"=w429:T10, "Index"=w420:i32)  [unwired: 6 in, 1 out]
                    n224 = Unbundle By Name(w428) -> ("Position"=w414:dbl, "Pos limit"=w422:dbl)
                    n225 = Unbundle By Name(w427) -> ("Position"=w413:dbl, "Pos limit"=w421:dbl)
                    n226 = Unbundle By Name(w429) -> ("Position"=w412:dbl, "Pos limit"=w423:dbl)
                    n227 = Subtract(x=w422, y=w430) -> (x-y=w433:dbl)
                    n228 = Subtract(x=w421, y=w430) -> (x-y=w432:dbl)
                    n229 = Subtract(x=w423, y=w430) -> (x-y=w434:dbl)
                    n230 = property class="Bool (strict)"(reference=w409, "Value"=FALSE) -> ()  [unwired: 1 in, 2 out]
                    n231 = Less?(x=w413, y=w432) -> (x < y?=w417:bool)
                    n232 = Less?(x=w412, y=w434) -> (x < y?=w415:bool)
                    n233 = Less?(x=w414, y=w433) -> (x < y?=w416:bool)
                    n234 = Compound Arithmetic op=AND(w416, w417, w415) -> (w431:bool)
                    n235 = case shown="True" w431 {
                      tunnel: w430 -> [_ w442]
                      tunnel: w420 -> [_ w443]
                      tunnel: w419 -> [_ w441]
                      tunnel: w418 -> [_ w440]
                      tunnel: w411 -> [_ w437]
                      frame False {
                      }
                      frame True {
                        n236 = Initialize Array(0.0 ("element"), 5 ("dimension size")) -> (w449:dbl[])
                        n237 = Replace Array Subset(array=w449, new element=w442, index=w441) -> (w446:dbl[])
                        n238 = Replace Array Subset(array=w446, new element=w442, index=w440) -> (w445:dbl[])
                        n239 = Replace Array Subset(array=w445, new element=w442, index=w443) -> (w444:dbl[])
                        n240 = Unbundle By Name(w437) -> ("Table_C"=w439:refnum<queue>)
                        n241 = Bundle By Name(cluster=T39 {"Command"=enum."Move by", "Data"=variant(dbl[] [])} ("MSG to Servo"), "Command"=Servo_commands."Move by", "Data"=w444) -> (w438:T39)
                        n242 = call "Put in mailbox.vi"("Message"=w438, "Queue in"=w439) -> ()  [unwired: 7 in, 3 out]
                      }
                    }
                  }
                  event Value Change {
                    w472 = 0.5 ("y")
                    n243 = event-data() -> ("CtlRef"=w453:refnum<vi>)  [unwired: 1 in, 5 out]
                    n244 = Unbundle By Name(w451) -> ("Servo"=w452:T10[])
                    n245 = call "Extract axis properties.vi"("Name"=Axis_names."AxisZ_middle", "All servo status"=w452) -> ("Servo"=w468:T10, "Index"=w461:i32)  [unwired: 6 in, 1 out]
                    n246 = call "Extract axis properties.vi"("Name"=Axis_names."AxisZ_left", "All servo status"=w452) -> ("Servo"=w471:T10, "Index"=w460:i32)  [unwired: 6 in, 1 out]
                    n247 = call "Extract axis properties.vi"("Name"=Axis_names."AxisZ_right", "All servo status"=w452) -> ("Servo"=w469:T10, "Index"=w459:i32)  [unwired: 6 in, 1 out]
                    n248 = Unbundle By Name(w469) -> ("Position"=w457:dbl, "Neg limit"=w464:dbl)
                    n249 = Unbundle By Name(w471) -> ("Position"=w458:dbl, "Neg limit"=w465:dbl)
                    n250 = Unbundle By Name(w468) -> ("Position"=w456:dbl, "Neg limit"=w463:dbl)
                    n251 = property class="Bool (strict)"(reference=w453, "Value"=FALSE) -> ()  [unwired: 1 in, 2 out]
                    n252 = Add(x=w465, y=w472) -> (x+y=w479:dbl)
                    n253 = Add(x=w464, y=w472) -> (x+y=w478:dbl)
                    n254 = Add(x=w463, y=w472) -> (x+y=w477:dbl)
                    n255 = Greater?(x=w458, y=w479) -> (0:w476:bool)
                    n256 = Greater?(x=w457, y=w478) -> (0:w475:bool)
                    n257 = Greater?(x=w456, y=w477) -> (0:w473:bool)
                    n258 = Negate(x=w472) -> (-x=w462:dbl)
                    n259 = Compound Arithmetic op=AND(w476, w475, w473) -> (w474:bool)
                    n260 = case shown="True" w474 {
                      tunnel: w462 -> [_ w488]
                      tunnel: w461 -> [_ w487]
                      tunnel: w460 -> [_ w486]
                      tunnel: w459 -> [_ w485]
                      tunnel: w455 -> [_ w481]
                      frame False {
                      }
                      frame True {
                        n261 = Initialize Array(0.0 ("element"), 5 ("dimension size")) -> (w494:dbl[])
                        n262 = Replace Array Subset(array=w494, new element=w488, index=w487) -> (w491:dbl[])
                        n263 = Replace Array Subset(array=w491, new element=w488, index=w486) -> (w490:dbl[])
                        n264 = Replace Array Subset(array=w490, new element=w488, index=w485) -> (w489:dbl[])
                        n265 = Bundle By Name(cluster=T39 {"Command"=enum."Move by", "Data"=variant(dbl[] [])} ("MSG to Servo"), "Command"=Servo_commands."Move by", "Data"=w489) -> (w482:T39)
                        n266 = Unbundle By Name(w481) -> ("Table_C"=w483:refnum<queue>)
                        n267 = call "Put in mailbox.vi"("Message"=w482, "Queue in"=w483) -> ()  [unwired: 7 in, 3 out]
                      }
                    }
                  }
                  event Value Change {
                    w506 = 0.5 ("y")
                    n268 = event-data() -> ("CtlRef"=w498:refnum<vi>)  [unwired: 1 in, 5 out]
                    n269 = Unbundle By Name(w497) -> ("Servo"=w496:T10[])
                    n270 = call "Extract axis properties.vi"("Name"=Axis_names."AxisZ_left", "All servo status"=w496) -> ("Servo"=w505:T10, "Index"=w502:i32)  [unwired: 6 in, 1 out]
                    n271 = Unbundle By Name(w505) -> ("Position"=w501:dbl, "Pos limit"=w503:dbl)
                    n272 = Subtract(x=w503, y=w506) -> (x-y=w507:dbl)
                    n273 = property class="Bool (strict)"(reference=w498, "Value"=FALSE) -> ()  [unwired: 1 in, 2 out]
                    n274 = Less?(x=w501, y=w507) -> (x < y?=w508:bool)
                    n275 = case shown="False" w508 {
                      tunnel: w506 -> [_ w519]
                      tunnel: w502 -> [_ w514]
                      tunnel: w500 -> [_ w510]
                      frame False {
                      }
                      frame True {
                        n276 = Initialize Array(0.0 ("element"), 5 ("dimension size")) -> (w518:dbl[])
                        n277 = Replace Array Subset(array=w518, new element=w519, index=w514) -> (w515:dbl[])
                        n278 = Bundle By Name(cluster=T39 {"Command"=enum."Move by", "Data"=variant(dbl[] [])} ("MSG to Servo"), "Command"=Servo_commands."Move by", "Data"=w515) -> (w511:T39)
                        n279 = Unbundle By Name(w510) -> ("Table_C"=w512:refnum<queue>)
                        n280 = call "Put in mailbox.vi"("Message"=w511, "Queue in"=w512) -> ()  [unwired: 7 in, 3 out]
                      }
                    }
                  }
                  event Value Change {
                    w531 = 0.5 ("y")
                    n281 = event-data() -> ("CtlRef"=w523:refnum<vi>)  [unwired: 1 in, 5 out]
                    n282 = Unbundle By Name(w521) -> ("Servo"=w522:T10[])
                    n283 = call "Extract axis properties.vi"("Name"=Axis_names."AxisZ_left", "All servo status"=w522) -> ("Servo"=w530:T10, "Index"=w527:i32)  [unwired: 6 in, 1 out]
                    n284 = Unbundle By Name(w530) -> ("Position"=w526:dbl, "Neg limit"=w528:dbl)
                    n285 = property class="Bool (strict)"(reference=w523, "Value"=FALSE) -> ()  [unwired: 1 in, 2 out]
                    n286 = Add(x=w528, y=w531) -> (x+y=w532:dbl)
                    n287 = Greater?(x=w526, y=w532) -> (0:w533:bool)
                    n288 = case shown="True" w533 {
                      tunnel: w531 -> [_ w543]
                      tunnel: w527 -> [_ w539]
                      tunnel: w525 -> [_ w536]
                      frame False {
                      }
                      frame True {
                        n289 = Negate(x=w543) -> (-x=w545:dbl)
                        n290 = Initialize Array(0.0 ("element"), 5 ("dimension size")) -> (w544:dbl[])
                        n291 = Replace Array Subset(array=w544, new element=w545, index=w539) -> (w540:dbl[])
                        n292 = Bundle By Name(cluster=T39 {"Command"=enum."Move by", "Data"=variant(dbl[] [])} ("MSG to Servo"), "Command"=Servo_commands."Move by", "Data"=w540) -> (w535:T39)
                        n293 = Unbundle By Name(w536) -> ("Table_C"=w537:refnum<queue>)
                        n294 = call "Put in mailbox.vi"("Message"=w535, "Queue in"=w537) -> ()  [unwired: 7 in, 3 out]
                      }
                    }
                  }
                  event Value Change {
                    w557 = 0.5 ("y")
                    n295 = event-data() -> ("CtlRef"=w549:refnum<vi>)  [unwired: 1 in, 5 out]
                    n296 = Unbundle By Name(w547) -> ("Servo"=w548:T10[])
                    n297 = call "Extract axis properties.vi"("Name"=Axis_names."AxisZ_right", "All servo status"=w548) -> ("Servo"=w556:T10, "Index"=w553:i32)  [unwired: 6 in, 1 out]
                    n298 = property class="Bool (strict)"(reference=w549, "Value"=FALSE) -> ()  [unwired: 1 in, 2 out]
                    n299 = Unbundle By Name(w556) -> ("Position"=w552:dbl, "Pos limit"=w554:dbl)
                    n300 = Subtract(x=w554, y=w557) -> (x-y=w559:dbl)
                    n301 = Less?(x=w552, y=w559) -> (x < y?=w558:bool)
                    n302 = case shown="True" w558 {
                      tunnel: w557 -> [_ w569]
                      tunnel: w553 -> [_ w565]
                      tunnel: w551 -> [_ w561]
                      frame False {
                      }
                      frame True {
                        n303 = Initialize Array(0.0 ("element"), 5 ("dimension size")) -> (w570:dbl[])
                        n304 = Replace Array Subset(array=w570, new element=w569, index=w565) -> (w566:dbl[])
                        n305 = Bundle By Name(cluster=T39 {"Command"=enum."Move by", "Data"=variant(dbl[] [])} ("MSG to Servo"), "Command"=Servo_commands."Move by", "Data"=w566) -> (w562:T39)
                        n306 = Unbundle By Name(w561) -> ("Table_C"=w563:refnum<queue>)
                        n307 = call "Put in mailbox.vi"("Message"=w562, "Queue in"=w563) -> ()  [unwired: 7 in, 3 out]
                      }
                    }
                  }
                  event Value Change {
                    w581 = 0.5 ("y")
                    n308 = event-data() -> ("CtlRef"=w574:refnum<vi>)  [unwired: 1 in, 5 out]
                    n309 = Unbundle By Name(w572) -> ("Servo"=w573:T10[])
                    n310 = call "Extract axis properties.vi"("Name"=Axis_names."AxisZ_right", "All servo status"=w573) -> ("Servo"=w580:T10, "Index"=w578:i32)  [unwired: 6 in, 1 out]
                    n311 = property class="Bool (strict)"(reference=w574, "Value"=FALSE) -> ()  [unwired: 1 in, 2 out]
                    n312 = Unbundle By Name(w580) -> ("Position"=w577:dbl, "Neg limit"=w583:dbl)
                    n313 = Add(x=w583, y=w581) -> (x+y=w582:dbl)
                    n314 = Greater?(x=w577, y=w582) -> (0:w584:bool)
                    n315 = case shown="True" w584 {
                      tunnel: w581 -> [_ w594]
                      tunnel: w578 -> [_ w590]
                      tunnel: w576 -> [_ w586]
                      frame False {
                      }
                      frame True {
                        n316 = Negate(x=w594) -> (-x=w596:dbl)
                        n317 = Initialize Array(0.0 ("element"), 5 ("dimension size")) -> (w595:dbl[])
                        n318 = Replace Array Subset(array=w595, new element=w596, index=w590) -> (w591:dbl[])
                        n319 = Bundle By Name(cluster=T39 {"Command"=enum."Move by", "Data"=variant(dbl[] [])} ("MSG to Servo"), "Command"=Servo_commands."Move by", "Data"=w591) -> (w587:T39)
                        n320 = Unbundle By Name(w586) -> ("Table_C"=w588:refnum<queue>)
                        n321 = call "Put in mailbox.vi"("Message"=w587, "Queue in"=w588) -> ()  [unwired: 7 in, 3 out]
                      }
                    }
                  }
                  event Value Change {
                    w608 = 0.5 ("y")
                    n322 = event-data() -> ("CtlRef"=w600:refnum<vi>)  [unwired: 1 in, 5 out]
                    n323 = Unbundle By Name(w598) -> ("Servo"=w599:T10[])
                    n324 = call "Extract axis properties.vi"("Name"=Axis_names."AxisZ_middle", "All servo status"=w599) -> ("Servo"=w607:T10, "Index"=w604:i32)  [unwired: 6 in, 1 out]
                    n325 = Unbundle By Name(w607) -> ("Position"=w603:dbl, "Pos limit"=w605:dbl)
                    n326 = property class="Bool (strict)"(reference=w600, "Value"=FALSE) -> ()  [unwired: 1 in, 2 out]
                    n327 = Subtract(x=w605, y=w608) -> (x-y=w609:dbl)
                    n328 = Less?(x=w603, y=w609) -> (x < y?=w610:bool)
                    n329 = case shown="True" w610 {
                      tunnel: w608 -> [_ w620]
                      tunnel: w604 -> [_ w616]
                      tunnel: w602 -> [_ w612]
                      frame False {
                      }
                      frame True {
                        n330 = Initialize Array(0.0 ("element"), 5 ("dimension size")) -> (w621:dbl[])
                        n331 = Replace Array Subset(array=w621, new element=w620, index=w616) -> (w617:dbl[])
                        n332 = Bundle By Name(cluster=T39 {"Command"=enum."Move by", "Data"=variant(dbl[] [])} ("MSG to Servo"), "Command"=Servo_commands."Move by", "Data"=w617) -> (w613:T39)
                        n333 = Unbundle By Name(w612) -> ("Table_C"=w614:refnum<queue>)
                        n334 = call "Put in mailbox.vi"("Message"=w613, "Queue in"=w614) -> ()  [unwired: 7 in, 3 out]
                      }
                    }
                  }
                  event Value Change {
                    w633 = 0.5 ("y")
                    n335 = event-data() -> ("CtlRef"=w625:refnum<vi>)  [unwired: 1 in, 5 out]
                    n336 = Unbundle By Name(w623) -> ("Servo"=w624:T10[])
                    n337 = call "Extract axis properties.vi"("Name"=Axis_names."AxisZ_middle", "All servo status"=w624) -> ("Servo"=w631:T10, "Index"=w629:i32)  [unwired: 6 in, 1 out]
                    n338 = property class="Bool (strict)"(reference=w625, "Value"=FALSE) -> ()  [unwired: 1 in, 2 out]
                    n339 = Unbundle By Name(w631) -> ("Position"=w628:dbl, "Neg limit"=w630:dbl)
                    n340 = Add(x=w630, y=w633) -> (x+y=w634:dbl)
                    n341 = Greater?(x=w628, y=w634) -> (0:w635:bool)
                    n342 = case shown="True" w635 {
                      tunnel: w633 -> [_ w645]
                      tunnel: w629 -> [_ w641]
                      tunnel: w627 -> [_ w638]
                      frame False {
                      }
                      frame True {
                        n343 = Negate(x=w645) -> (-x=w647:dbl)
                        n344 = Initialize Array(0.0 ("element"), 5 ("dimension size")) -> (w646:dbl[])
                        n345 = Replace Array Subset(array=w646, new element=w647, index=w641) -> (w642:dbl[])
                        n346 = Bundle By Name(cluster=T39 {"Command"=enum."Move by", "Data"=variant(dbl[] [])} ("MSG to Servo"), "Command"=Servo_commands."Move by", "Data"=w642) -> (w637:T39)
                        n347 = Unbundle By Name(w638) -> ("Table_C"=w639:refnum<queue>)
                        n348 = call "Put in mailbox.vi"("Message"=w637, "Queue in"=w639) -> ()  [unwired: 7 in, 3 out]
                      }
                    }
                  }
                  event Value Change {
                    n349 = event-data() -> ()  [unwired: 1 in, 6 out]
                    n350 = Unbundle By Name(w649) -> ("Magnet.Ramp [mT/s]"=w651:dbl, "Magnet.Field [T]"=w652:dbl)
                    n351 = Unbundle By Name(w650) -> ("Angle_C"=w662:refnum<queue>)
                    n352 = Less?(x=w652, y=8.0) -> (x < y?=w654:bool)
                    n353 = Not Equal To 0?(x=w651) -> (x != 0?=w655:bool)
                    n354 = And(x=w655, y=w654) -> (x .and. y?=w656:bool)
                    n355 = Select(t=TRUE, s=w656, f=FALSE ("x .and. y?")) -> (s? t:f=w661:bool)
                    n356 = local read "Rotator controls"() -> (w659:T22)
                    n357 = Unbundle By Name(w659) -> ("Set position"=w660:T24)
                    n358 = Bundle By Name(cluster=w660, "Safe to move?"=w661) -> (w665:T24)
                    n359 = Bundle By Name(cluster=T42 {"Command"=enum."Set position", "Data"=variant} ("MSG to rotator"), "Data"=w665) -> (w664:T42)
                    n360 = call "Put in mailbox.vi"("Message"=w664, "Queue in"=w662) -> ()  [unwired: 7 in, 3 out]
                  }
                  event Value Change {
                    n361 = event-data() -> ("CtlRef"=w668:refnum<vi>)  [unwired: 1 in, 5 out]
                    n362 = Unbundle By Name(w669) -> ("Angle_C"=w673:refnum<queue>)
                    n363 = Unbundle By Name("Rotator controls") -> ("Motion properties"=w674:T23)
                    n364 = Unbundle By Name(w674) -> ("DC voltage [V]"=w679:dbl)
                    n365 = property class="Bool (strict)"(reference=w668, "Value"=FALSE) -> ()  [unwired: 1 in, 2 out]
                    n366 = Greater Than 0?(x=w679) -> (x > 0?=w675:bool)
                    n367 = case shown="True" w675 {
                      tunnel: [_ w682] -> w677
                      frame False {
                      }
                      frame True {
                        n368 = Two Button Dialog(message="DC Voltage is not zero.\nDo you realy want to set it?") -> (T button?=w682:bool)  [unwired: 2 in]
                      }
                    }
                    n369 = Select(t=w679, s=w677, f=0.0) -> (s? t:f=w678:dbl)
                    n370 = Bundle By Name(cluster=w674, "DC voltage [V]"=w678) -> (w676:T23)
                    n371 = Bundle By Name(cluster=T42 {"Command"=enum."Set parameters", "Data"=variant} ("MSG to rotator"), "Data"=w676) -> (w672:T42)
                    n372 = call "Put in mailbox.vi"("Message"=w672, "Queue in"=w673) -> ()  [unwired: 7 in, 3 out]
                  }
                  event Value Change {
                    n373 = event-data() -> ("CtlRef"=w684:refnum<vi>)  [unwired: 1 in, 5 out]
                    n374 = Unbundle By Name(w687) -> ("Angle_C"=w686:refnum<queue>)
                    n375 = property class="Bool (strict)"(reference=w684, "Value"=FALSE) -> ()  [unwired: 1 in, 2 out]
                    n376 = call "Put in mailbox.vi"("Message"=T42 {"Command"=enum."Stop movement", "Data"=variant} ("MSG to rotator"), "Queue in"=w686) -> ()  [unwired: 7 in, 3 out]
                  }
                  event Value Change {
                    n377 = event-data() -> ()  [unwired: 1 in, 6 out]
                    n378 = Unbundle By Name(w702) -> ("MW_C"=w701:refnum<queue>)
                    n379 = Unbundle By Name("VID control") -> ("AMC"=w700:u16, "Multip"=w699:u16, "Base frequency [GHz]"=w707:dbl, "End frequency [GHz]"=w708:dbl, "Im frequency [MHz]"=w709:dbl, "Sweep up [ms]"=w691:dbl, "Reset trigger?"=w693:bool)
                    n380 = Multiply(x=w700, y=w699) -> (x*y=w695:u16)
                    n381 = Divide(x=w707, y=w695) -> (x/y=w698:dbl)
                    n382 = Divide(x=w708, y=w695) -> (x/y=w697:dbl)
                    n383 = Divide(x=w709, y=w695) -> (x/y=w696:dbl)
                    n384 = Divide(x=w691, y=2.0) -> (x/y=w690:dbl)
                    n385 = Bundle By Name(cluster=T45 {"Start [GHz]"=8.0, "End [GHz] "=8.0, "Sweep up\ntime [ms]"=0.0, "Sweep down\ntime [ms]"=0.0, "Intermidiate [MHz]"=0.0, "Reset trigger"=FALSE} ("Sweep parameters"), "Start [GHz]"=w698, "End [GHz]"=w697, "Intermidiate [MHz]"=w696, "Sweep up\ntime [ms]"=w691, "Sweep down\ntime [ms]"=w690, "Reset trigger"=w693) -> (w704:T45)
                    n386 = Bundle By Name(cluster=T46 {"Command"=enum."Set parameters", "Data"=variant} ("Incoming msg"), "Command"=THz_commands_enum."Set parameters", "Data"=w704) -> (w705:T46)
                    n387 = call "Put in mailbox.vi"("Message"=w705, "Queue in"=w701) -> ()  [unwired: 7 in, 3 out]
                  }
                  event Value Change {
                    n388 = event-data() -> ()  [unwired: 1 in, 6 out]
                    n389 = local read "VID control"() -> (w719:T17)
                    n390 = Unbundle By Name(w719) -> ("AMC"=w716:u16, "Multip"=w715:u16)
                    n391 = Multiply(x=w716, y=w715) -> (x*y=w714:u16)
                    n392 = Multiply(x=14.0, y=w714) -> (x*y=w713:dbl)
                    n393 = Multiply(x=9.0, y=w714) -> (x*y=w712:dbl)
                    n394 = property on="AMC" class="Ring (strict)"("Minimum"=w712, "Maximum"=w713) -> ()  [unwired: 2 in, 2 out]
                    n395 = property on="Base frequency [GHz]" class="DigNum (strict)"("Minimum"=w712, "Maximum"=w713) -> ()  [unwired: 2 in, 2 out]
                  }
                  event Value Change {
                    n396 = event-data() -> ("CtlRef"=w727:refnum<vi>, "NewVal"=w724:dbl)  [unwired: 1 in]
                    n397 = property class="DigNum (strict)"(reference=w727) -> ("Label.Text"=w726:string)  [unwired: 1 in, 2 out]
                    n398 = Unbundle By Name(w734) -> ("Data_Aq"=w733:refnum<queue>)
                    n399 = case shown="\"Amp_Mod [mV]\"" w726 {
                      tunnel: [MFLI_node."None" ("parameter") MFLI_node."filter_constant [ms]" ("parameter") MFLI_node."filter_order [-]" ("parameter") MFLI_node."osc_freq [kHz]" ("parameter") MFLI_node."out_ampl [V]" ("parameter")] -> w722
                      tunnel: w724 -> [_ w738 w740 w742 w747]
                      tunnel: [_ w738 w740 w742 w758] -> w725
                      tunnel: "Acquisition controls" -> [_ _ _ _ w744]
                      tunnel: [_ _ _ _ w745] -> _
                      frame "Unknown", Default {
                      }
                      frame "Filter tau [ms]" {
                      }
                      frame "Filter order" {
                      }
                      frame "F_Mod [kHz]" {
                      }
                      frame "Amp_Mod [mV]" {
                        n400 = Unbundle By Name(w744) -> ("Sample holder"=w743:T16, "ACQ parameters.F_Mod [kHz]"=w754:dbl)
                        n401 = case shown="\"Rotator\"" w743 {
                          tunnel: [w762 w765 w768 w771] -> w756
                          tunnel: [w761 w764 w767 w770] -> w752
                          tunnel: [w760 w763 w766 w769] -> w746
                          frame "Simple", Default {
                            w760 = 0.0  # G/A
                            w761 = 8.9  # R
                            w762 = 0.0017  # L
                          }
                          frame "Carousel" {
                            w763 = 0.0  # G/A
                            w764 = 8.9  # R
                            w765 = 0.0017  # L
                          }
                          frame "Chip" {
                            w766 = 0.0  # G/A
                            w767 = 8.9  # R
                            w768 = 0.0017  # L
                          }
                          frame "Rotator" {
                            w769 = 0.0  # G/A
                            w770 = 8.9  # R
                            w771 = 0.0017  # L
                          }
                        }
                        n402 = Square(x=w752) -> (x^2=w750:dbl)
                        n403 = Divide(x=w747, y=1000.0) -> (x/y=w758:dbl)
                        n404 = Compound Arithmetic op=MULTIPLY(w754, 6.283185307179586, w756) -> (w753:dbl)
                        n405 = Square(x=w753) -> (x^2=w751:dbl)
                        n406 = Add(x=w751, y=w750) -> (x+y=w749:dbl)
                        n407 = Square Root(x=w749) -> (sqrt(x)=w748:dbl)
                        n408 = Compound Arithmetic op=MULTIPLY(w746, w748) -> (w745:dbl)
                      }
                    }
                    n409 = Bundle(cluster=T47 {"parameter"=enum."filter_order [-]", "value"=0.0} ("Parameter to set"), "parameter"=w722, "value"=w725) -> (w728:T47)
                    n410 = Build Array(w728) -> (w723:T47[])
                    n411 = Bundle By Name(cluster=T50 {"Command"=enum."Initialize", "Data"=variant} ("MSG for  ACQ"), "Command"=MFLI_command_enum."Set individual parameters", "Data"=w723) -> (w730:T50)
                    n412 = call "Put in mailbox.vi"("Message"=w730, "Queue in"=w733) -> ()  [unwired: 7 in, 3 out]
                  }
                  event Value Change {
                    w775 = T47 {"parameter"=enum."filter_order [-]", "value"=0.0} ("Parameter to set")
                    n413 = event-data() -> ("NewVal"=w773:u16)  [unwired: 1 in, 2 out]
                    n414 = Unbundle By Name(w783) -> ("Data_Aq"=w782:refnum<queue>)
                    n415 = Bundle(cluster=w775, "parameter"=MFLI_node."enable output", "value"=w773) -> (w778:T47)
                    n416 = Bundle(cluster=w775, "parameter"=MFLI_node."enamble ampl", "value"=w773) -> (w772:T47)
                    n417 = Build Array(w778, w772) -> (w777:T47[])
                    n418 = Bundle By Name(cluster=T50 {"Command"=enum."Initialize", "Data"=variant} ("MSG for  ACQ"), "Command"=MFLI_command_enum."Set individual parameters", "Data"=w777) -> (w779:T50)
                    n419 = call "Put in mailbox.vi"("Message"=w779, "Queue in"=w782) -> ()  [unwired: 7 in, 3 out]
                  }
                  event Value Change {
                    n420 = event-data() -> ("CtlRef"=w790:refnum<vi>, "NewVal"=w788:dbl)  [unwired: 1 in]
                    n421 = property class="DigNum (strict)"(reference=w790) -> ("Label.Text"=w789:string)  [unwired: 1 in, 2 out]
                    n422 = Unbundle By Name(w794) -> ("Tmp_C"=w791:refnum<queue>)
                    n423 = Bundle(cluster=T51 {"Heater"="None", "Tmp [K]"=0.0} ("Set point"), "Heater"=w789, "Tmp [K]"=w788) -> (w785:T51)
                    n424 = Bundle By Name(cluster=T53 {"Command"=enum."Initialize", "Data"=variant}, "Command"=TC_commands."Set point", "Data"=w785) -> (w792:T53)
                    n425 = call "Put in mailbox.vi"("Message"=w792, "Queue in"=w791) -> ()  [unwired: 7 in, 3 out]
                  }
                  event "Password is admin": Value Change {
                    n426 = event-data() -> ("NewVal"=w800:string)  [unwired: 1 in, 1 out]
                    n427 = Equal?(x="admin", y=w800) -> (x = y?=w796:bool)
                    n428 = case shown="True" w796 {
                      tunnel: [T33."Disabled and Grayed Out" ("Disabled") T33."Enabled" ("Disabled")] -> w797
                      frame False {
                      }
                      frame True {
                      }
                    }
                    n429 = local read "Instr control refs"() -> (w798:refnum<vi>[])
                    n430 = call "Dis- or en- able controls.vi"("Disabled"=w797, "Control referencies"=w798) -> ()  [unwired: 9 in, 1 out]
                  }
                }
              }
              frame "Measurement" {
                n431 = event shown="[3] \"Direct stop meas. btn\": Value Change" {
                  selector: _ -> [_ _ _ _ _]
                  dyn-events: _ -> [_ _ _ _ _]
                  timeout: 0 -> [_ _ _ _ _]
                  tunnel: w811 -> [w814 w817 w828 w855 w881]
                  tunnel: [w814 w817 w827 w855 w881] -> w810
                  tunnel: w808 -> [_ _ _ w854 _]
                  tunnel: [w813 w816 w823 w851 w878] -> w807
                  tunnel: w806 -> [w813 w816 _ w851 w878]
                  tunnel: w805 -> [w812 _ w821 w850 w875]
                  tunnel: [w812 _ w822 w847 w875] -> w804
                  event Timeout {
                    n432 = event-data() -> ()  [unwired: 1 in, 3 out]
                  }
                  event "Load from editor btn": Value Change {
                    n433 = event-data() -> ()  [unwired: 1 in, 6 out]
                    n434 = local read "Editor script"() -> (w815:T25[])
                    n435 = local write "Script array"(w815) -> ()
                  }
                  event "Run FDMR+ btn": Value Change {
                    n436 = event-data() -> ()  [unwired: 1 in, 6 out]
                    n437 = control-ref of="Direct stop meas. btn"() -> (w819:refnum<vi>)
                    n438 = Build Array(w819) -> (w820:refnum<vi>[])
                    n439 = call "Dis- or en- able controls.vi"("Disabled"=T33."Enabled", "Control referencies"=w820) -> ()  [unwired: 9 in, 1 out]
                    n440 = for {
                      tunnel: "Script array" -> [w843] mode=indexing
                      tunnel: [w843] -> w823
                      tunnel: [w841] -> w824
                      i -> [w842]
                      stop <- w841 stop-if-true
                      n441 = Build Array(w842) -> (w844:i32[])
                      n442 = Build Array(1) -> (w845:i32[])
                      n443 = Unbundle By Name(w843) -> ("Execute"=w841:bool)
                      n444 = property on="Script array" class="Arr (strict)"("Selection Size []"=w845, "Selection Start []"=w844) -> ()  [unwired: 2 in, 2 out]
                    }
                    n445 = case shown="True" w824 {
                      tunnel: w821 -> [w829 w839]
                      tunnel: [w829 w837] -> w822
                      frame False {
                      }
                      frame True {
                        n446 = local read "Folder path"() -> (w830:path)
                        n447 = local read "Instr control refs"() -> (w833:refnum<vi>[])
                        n448 = call "Create TDMS FDMR file.vi"("Sample name"="Sample name", "Folder path"=w830) -> ("tdms map file out"=→"tdms FDMR file ref":refnum<k34>)  [unwired: 8 in, 1 out]
                        n449 = control-ref of="Run FDMR+ btn"() -> (w836:refnum<vi>)
                        n450 = control-ref of="Open measurement"() -> (w835:refnum<vi>)
                        n451 = Bundle By Name(cluster=w839, "Experiment state"=experiment_state."Preparation" ("Value")) -> (w837:T27)
                        n452 = Build Array (concatenate)(w833, w836, w835) -> (w834:refnum<vi>[])
                        n453 = call "Dis- or en- able controls.vi"("Disabled"=T33."Disabled and Grayed Out", "Control referencies"=w834) -> ()  [unwired: 9 in, 1 out]
                      }
                    }
                    n454 = call "simple Shift string array.vi"("Element in"="Preparing for measurement.", "Array in"=w828) -> ("Array out"=w827:string[])  [unwired: 8 in, 1 out]
                  }
                  event "Direct stop meas. btn": Value Change {
                    n455 = event-data() -> ("NewVal"=w853:bool)  [unwired: 1 in, 5 out]
                    n456 = call "Timeout dialoge Abbort.vi"("Enable"=w853, "Message to Display"="Realy abbort measurement?", "timeout[ms]"=u32 5000) -> ("Yes"=w852:bool)  [unwired: 15 in, 1 out]
                    n457 = case shown="True" w852 {
                      tunnel: w854 -> [_ w874]
                      tunnel: w850 -> [w856 w861]
                      tunnel: [w856 w860] -> w847
                      frame False {
                      }
                      frame True {
                        n458 = Unbundle By Name(w874) -> ("Field_C"=w868:refnum<queue>, "Tmp_C"=w869:refnum<queue>, "Angle_C"=w870:refnum<queue>)
                        n459 = local write "Run FDMR+ btn"(FALSE ("Direct stop meas. btn")) -> ()
                        n460 = Bundle By Name(cluster=w861, "Experiment state"=experiment_state."Save" ("Value")) -> (w860:T27)
                        n461 = local read "Instr control refs"() -> (w863:refnum<vi>[])
                        n462 = control-ref of="Run FDMR+ btn"() -> (w857:refnum<vi>)
                        n463 = Build Array (concatenate)(w857, w863) -> (w864:refnum<vi>[])
                        n464 = call "Put in mailbox.vi"("Message"=T37 {"Command"=enum."Stop ramping", "Data"=variant} ("MSG to magnet"), "Queue in"=w868) -> ("error out"=w867:errorcluster)  [unwired: 7 in, 2 out]
                        n465 = call "Put in mailbox.vi"("error in (no error)"=w867, "Message"=T53 {"Command"=enum."Stop tmp change", "Data"=variant} ("MSG for VTI"), "Queue in"=w869) -> ("error out"=w866:errorcluster)  [unwired: 6 in, 2 out]
                        n466 = call "Put in mailbox.vi"("error in (no error)"=w866, "Message"=T42 {"Command"=enum."Stop movement", "Data"=variant} ("MSG to rotator"), "Queue in"=w870) -> ("error out"=w858:errorcluster)  [unwired: 6 in, 2 out]
                        n467 = call "Dis- or en- able controls.vi"("error in"=w858, "Disabled"=T33."Enabled", "Control referencies"=w864) -> ()  [unwired: 8 in, 1 out]
                      }
                    }
                  }
                  event "Sample name": Value Change {
                    n468 = event-data() -> ("CtlRef"=w877:refnum<vi>, "NewVal"=w880:string)  [unwired: 1 in, 4 out]
                    n469 = Search and Replace String(replace all?=TRUE ("replace all? (F)"), input string=w880, search string="[<>:\"/\\|?*%]" ("regular expression"), replace string="-" ("replace string (\"\")")) -> (result string=w876:string)  [unwired: 4 in, 3 out]
                    n470 = property class="Str"(reference=w877, "Value"=w876) -> ()  [unwired: 1 in, 2 out]
                  }
                }
              }
              frame "Script editor" {
                n471 = event shown="[1] \"Generate script btn\": Value Change" {
                  selector: _ -> [_ _ _ _ _]
                  dyn-events: _ -> [_ _ _ _ _]
                  timeout: 0 -> [_ _ _ _ _]
                  tunnel: w891 -> [w894 w903 w907 w915 w929]
                  tunnel: [w894 w902 w907 w915 w929] -> w890
                  tunnel: w888 -> [_ _ _ _ _]
                  tunnel: [w893 w896 w906 w914 w928] -> w887
                  tunnel: w886 -> [w893 w896 w906 w914 w928]
                  tunnel: w885 -> [w892 w897 w905 _ _]
                  tunnel: [w892 w897 w905 _ _] -> w884
                  event Timeout {
                    n472 = event-data() -> ()  [unwired: 1 in, 3 out]
                  }
                  event "Generate script btn": Value Change {
                    n473 = event-data() -> ()  [unwired: 1 in, 6 out]
                    n474 = local read "Editor script"() -> (w895:T25[])
                    n475 = call "FDMR script generator.vi"("Generator options"="Generator options", "Prototype line"="Prototype line", "Editor script"=w895) -> ("Array"=w898:T25[])  [unwired: 8 in]
                    n476 = local write "Editor script"(w898) -> ()
                    n477 = call "simple Shift string array.vi"("Element in"="Preparing for measurement.", "Array in"=w903) -> ("Array out"=w902:string[])  [unwired: 8 in, 1 out]
                  }
                  event "Clear script btn": Value Change {
                    n478 = event-data() -> ()  [unwired: 1 in, 6 out]
                    n479 = local write "Editor script"(T25[] [] ("Editor script")) -> ()
                  }
                  event "Save script btn": Value Change {
                    n480 = event-data() -> ()  [unwired: 1 in, 6 out]
                    n481 = Current VI's Path() -> (path=w913:path)
                    n482 = call "File Dialog"("start path"=w913, "prompt"="Create script", "default name"="FDMR+ script.scp", "pattern (all files)"="*.scp") -> ("selected path"=w909:path, "cancelled"=w908:bool)  [unwired: 8 in, 2 out]
                    n483 = case shown="False" w908 {
                      tunnel: w909 -> [w920 _]
                      frame False {
                        n484 = call <vilib>:"Open Config Data.vi"("configuration file path"=w920) -> ("refnum"=w919:T74)  [unwired: 8 in, 2 out]
                        n485 = for {
                          tunnel: w919 -> [w926]
                          tunnel: "Editor script" -> [w924] mode=indexing
                          tunnel: [w923] -> w917
                          tunnel: [w922] -> w918
                          i -> [w921]
                          n486 = Number To Decimal String(number=w921) -> (decimal integer string=w925:string)  [unwired: 1 in]
                          n487 = call <userlib>:"Write Section Cluster__ogtk.vi"("section (optional)"=w925, "Section Formatted Cluster"=w924, "refnum"=w926) -> ("error out"=w923:errorcluster, "dup refnum"=w922:T74)  [unwired: 7 in]
                        }
                        n488 = call <vilib>:"Close Config Data.vi"("error in (no error)"=w917, "refnum"=w918) -> ()  [unwired: 8 in, 2 out]
                      }
                      frame True {
                      }
                    }
                  }
                  event "Load from measurement btn": Value Change {
                    n489 = event-data() -> ()  [unwired: 1 in, 6 out]
                    n490 = local read "Script array"() -> (w927:T25[])
                    n491 = local write "Editor script"(w927) -> ()
                  }
                }
              }
              frame "Measurement review" {
                n492 = event shown="[2] \"Open measurement\": Value Change" {
                  selector: _ -> [_ _ _]
                  dyn-events: _ -> [_ _ _]
                  timeout: 0 -> [_ _ _]
                  event Timeout {
                    n493 = event-data() -> ()  [unwired: 1 in, 3 out]
                  }
                  event "Data to show": Value Change {
                    n494 = event-data() -> ("NewVal"=w938:u16)  [unwired: 1 in, 5 out]
                    n495 = local read "Opend review file path"() -> (w937:path)
                    n496 = property on="Data to show" class="Ring (strict)"() -> ("Strings []"=w939:string[])  [unwired: 2 in, 2 out]
                    n497 = TDMS Open(11:w937) -> (0:w934:errorcluster, 3:w936:refnum<k34>)  [unwired: 6 in]
                    n498 = Index Array(array=w939, index=w938) -> (element=w935:string)
                    n499 = case shown="No Error" w934 {
                      tunnel: w936 -> [w962 _]
                      tunnel: w935 -> [w961 _]
                      frame No Error {
                        w959 = dbl[] []
                        w965 = u8 1 ("Y Scale.Scale Fit")
                        n500 = TDMS Read(0:w962, 5:w961, 7:"Y sum", 12:w959) -> (4:w957:refnum<k34>, 6:w960:string, 10:w941:dbl[], 15:w958:errorcluster)  [unwired: 4 in, 2 out]
                        n501 = property on="Current graph" class="WFGraph (strict)"() -> (error out=w964:errorcluster, "Value"=w967:sgl[][], "XScale.Multiplier"=w966:dbl, "XScale.Offset"=w948:dbl)  [unwired: 2 in, 1 out]
                        n502 = TDMS Read(0:w957, 5:w960, 7:"X sum", 11:w958, 12:w959) -> (4:w945:refnum<k34>, 6:w946:string, 10:w956:dbl[], 15:w944:errorcluster)  [unwired: 3 in, 2 out]
                        n503 = call "FDMR+ read TDMS properties.vi"("error in (no error)"=w944, "cahnnel group name in"=w946, "TDMS ref in"=w945) -> ("error out"=w942:errorcluster, "FDMR+ measurement parameters"=w940:T25, "TDMS ref out"=w943:refnum<k34>)  [unwired: 5 in, 1 out]
                        n504 = Build Array(w956, w941) -> (w955:dbl[][])
                        n505 = property on="Previous graph" class="WFGraph (strict)"(error in=w964, "Value"=w967, "XScale.Multiplier"=w966, "XScale.Offset"=w948, "YScale.ScaleFit"=w965) -> (error out=w963:errorcluster)  [unwired: 1 in, 1 out]
                        n506 = Unbundle By Name(w940) -> ("F_end [GHz]"=w952:dbl, "F_start [GHz]"=w947:dbl)
                        n507 = TDMS Close(8:w942, 11:w943) -> ()  [unwired: 2 out]
                        n508 = Array Size(array=w941) -> (size(s)=w953:i32)
                        n509 = Subtract(x=w952, y=w947) -> (x-y=w954:dbl)
                        n510 = local write "Current review graph parameters"(w940) -> ()
                        n511 = Divide(x=w954, y=w953) -> (x/y=w949:dbl)
                        n512 = property on="Current graph" class="WFGraph (strict)"(error in=w963, "Value"=w955, "XScale.Multiplier"=w949, "XScale.Offset"=w947, "YScale.ScaleFit"=w965) -> ()  [unwired: 1 in, 2 out]
                      }
                      frame Error {
                      }
                    }
                  }
                  event "Open measurement": Value Change {
                    n513 = event-data() -> ()  [unwired: 1 in, 1 out]
                    n514 = local read "Folder path"() -> (w971:path)
                    n515 = call "Read FDMR+data file.vi"("Application Directory"=w971) -> ("Error Out"=w970:errorcluster, "group names"=w973:string[], "Measurement parameters"=w972:T25, "First acummulated spectrum"=w969:T2, "TDMS File Path"=w968:path)  [unwired: 6 in]
                    n516 = case shown="No Error" w970 {
                      tunnel: w973 -> [w978 _]
                      tunnel: w972 -> [w977 _]
                      tunnel: w969 -> [w982 _]
                      tunnel: w968 -> [w975 _]
                      frame No Error {
                        n517 = property on="Data to show" class="Ring (strict)"("Strings []"=w978) -> ()  [unwired: 2 in, 2 out]
                        n518 = Unbundle(w982) -> ("X"=w981:sgl[], "Y"=w979:sgl[])
                        n519 = Build Array(w981, w979) -> (w980:sgl[][])
                        n520 = Unbundle By Name(w977) -> ("F_end [GHz]"=w976:dbl, "F_start [GHz]"=w974:dbl)
                        n521 = Array Size(array=w979) -> (size(s)=w985:i32)
                        n522 = Subtract(x=w976, y=w974) -> (x-y=w986:dbl)
                        n523 = Divide(x=w986, y=w985) -> (x/y=w983:dbl)
                        n524 = property on="Current graph" class="WFGraph (strict)"("Value"=w980, "XScale.Offset"=w974, "XScale.Multiplier"=w983, "YScale.ScaleFit"=u8 1 ("Y Scale.Scale Fit")) -> ()  [unwired: 2 in, 2 out]
                        "Current review graph parameters" <- w977
                        "Opend review file path" <- w975
                      }
                      frame Error {
                      }
                    }
                  }
                }
              }
            }
          }
          event "Tab Control": Value Change {
            n525 = event-data() -> ("NewVal"=w988:T6)  [unwired: 1 in, 5 out]
            n526 = case shown="\"Adjustment\"" w988 {
              frame "Page Status", Default {
              }
              frame "Adjustment" {
              }
            }
          }
          event "Disconnect": Value Change {
            n527 = event-data() -> ()  [unwired: 1 in, 6 out]
            n528 = local read "Select module"() -> (w992:T7)
            n529 = Equal?(x=w992, y=T32."All") -> (x = y?=w993:bool)
            n530 = case shown="True" w993 {
              tunnel: w991 -> [w998 w1028]
              tunnel: w992 -> [w999 _]
              frame False {
                n531 = case shown="\"THz\"" w999 {
                  tunnel: w998 -> [w1003 w1007 w1011 w1015 w1016 w1023 w1027 _]
                  frame "MAG" {
                    n532 = Unbundle By Name(w1003) -> ("Field_C"=w1001:refnum<queue>)
                    n533 = call "Put in mailbox.vi"("Priority? (F)"=TRUE ("Priority?"), "Message"=T37 {"Command"=enum."Eval temperatures", "Data"=variant} ("MSG to magnet"), "Queue in"=w1001) -> ()  [unwired: 6 in, 3 out]
                  }
                  frame "SMU" {
                    n534 = Unbundle By Name(w1007) -> ("Mod_M"=w1005:refnum<queue>)
                    n535 = call "Put in mailbox.vi"("Priority? (F)"=TRUE ("Priority?"), "Message"=T40 {"Command"=enum."Disconnect", "Data"=variant} ("MSG to Source meter"), "Queue in"=w1005) -> ()  [unwired: 6 in, 3 out]
                  }
                  frame "VTI" {
                    n536 = Unbundle By Name(w1011) -> ("Tmp_C"=w1009:refnum<queue>)
                    n537 = call "Put in mailbox.vi"("Priority? (F)"=TRUE ("Priority?"), "Message"=T53 {"Command"=enum."End", "Data"=variant} ("MSG for VTI"), "Queue in"=w1009) -> ()  [unwired: 6 in, 3 out]
                  }
                  frame "THz" {
                    n538 = Unbundle By Name(w1015) -> ("MW_C"=w1013:refnum<queue>)
                    n539 = call "Put in mailbox.vi"("Priority? (F)"=TRUE ("Priority?"), "Message"=T46 {"Command"=enum."End", "Data"=variant} ("Incoming msg"), "Queue in"=w1013) -> ()  [unwired: 6 in, 3 out]
                  }
                  frame "ACQ" {
                    n540 = Unbundle By Name(w1016) -> ("Data_Aq"=w1018:refnum<queue>)
                    n541 = call "Put in mailbox.vi"("Priority? (F)"=TRUE ("Priority?"), "Message"=T50 {"Command"=enum."End", "Data"=variant} ("MSG for  ACQ"), "Queue in"=w1018) -> ()  [unwired: 6 in, 3 out]
                  }
                  frame "SERV" {
                    n542 = Unbundle By Name(w1023) -> ("Table_C"=w1021:refnum<queue>)
                    n543 = call "Put in mailbox.vi"("Priority? (F)"=TRUE ("Priority?"), "Message"=T39 {"Command"=enum."End", "Data"=variant(dbl[] [])} ("MSG to Servo"), "Queue in"=w1021) -> ()  [unwired: 6 in, 3 out]
                  }
                  frame "ROT" {
                    n544 = Unbundle By Name(w1027) -> ("Angle_C"=w1025:refnum<queue>)
                    n545 = call "Put in mailbox.vi"("Priority? (F)"=TRUE ("Priority?"), "Message"=cluster{"Command":T43, "Data":variant} {"Command"=enum."Disconnect", "Data"=variant} ("MSG to rotator"), "Queue in"=w1025) -> ()  [unwired: 6 in, 3 out]
                  }
                  frame "None", Default {
                  }
                }
              }
              frame True {
                n546 = control-ref of="Instr status"() -> (w1029:refnum<vi>)
                n547 = property class="Clust (strict)"(reference=w1029) -> ("Controls[]"=w1030:refnum<vi>[])  [unwired: 1 in, 2 out]
                n548 = for {
                  tunnel: w1030 -> [w1036] mode=indexing
                  tunnel: w1028 -> [w1034]
                  n549 = property class="Ctl"(reference=w1036) -> ("Label.Text"=w1035:string, "Value"=w1033:variant)  [unwired: 1 in, 2 out]
                  n550 = Variant To Data(type=FALSE, Variant=w1033) -> (data=w1031:bool)  [unwired: 1 in, 1 out]
                  n551 = case shown="True" w1031 {
                    tunnel: w1035 -> [_ w1038]
                    tunnel: w1034 -> [_ w1037]
                    frame False {
                    }
                    frame True {
                      n552 = case shown="\"MFLI\"" w1038 {
                        tunnel: w1037 -> [w1042 w1046 w1050 w1054 w1058 w1062 w1066 _]
                        frame "Mag" {
                          n553 = Unbundle By Name(w1042) -> ("Field_C"=w1040:refnum<queue>)
                          n554 = call "Put in mailbox.vi"("Priority? (F)"=TRUE ("Priority?"), "Message"=T37 {"Command"=enum."Disconnect", "Data"=variant} ("MSG to magnet"), "Queue in"=w1040) -> ()  [unwired: 6 in, 3 out]
                        }
                        frame "SMU" {
                          n555 = Unbundle By Name(w1046) -> ("Mod_M"=w1044:refnum<queue>)
                          n556 = call "Put in mailbox.vi"("Priority? (F)"=TRUE ("Priority?"), "Message"=T40 {"Command"=enum."Disconnect", "Data"=variant} ("MSG to Source meter"), "Queue in"=w1044) -> ()  [unwired: 6 in, 3 out]
                        }
                        frame "VTI" {
                          n557 = Unbundle By Name(w1050) -> ("Tmp_C"=w1048:refnum<queue>)
                          n558 = call "Put in mailbox.vi"("Priority? (F)"=TRUE ("Priority?"), "Message"=T53 {"Command"=enum."Disconnect", "Data"=variant} ("MSG for VTI"), "Queue in"=w1048) -> ()  [unwired: 6 in, 3 out]
                        }
                        frame "THz" {
                          n559 = Unbundle By Name(w1054) -> ("MW_C"=w1052:refnum<queue>)
                          n560 = call "Put in mailbox.vi"("Priority? (F)"=TRUE ("Priority?"), "Message"=T46 {"Command"=enum."Disconnect", "Data"=variant} ("Incoming msg"), "Queue in"=w1052) -> ()  [unwired: 6 in, 3 out]
                        }
                        frame "MFLI" {
                          n561 = Unbundle By Name(w1058) -> ("Data_Aq"=w1056:refnum<queue>)
                          n562 = call "Put in mailbox.vi"("Priority? (F)"=TRUE ("Priority?"), "Message"=T50 {"Command"=enum."Disconnect", "Data"=variant} ("MSG for  ACQ"), "Queue in"=w1056) -> ()  [unwired: 6 in, 3 out]
                        }
                        frame "Serv" {
                          n563 = Unbundle By Name(w1062) -> ("Table_C"=w1060:refnum<queue>)
                          n564 = call "Put in mailbox.vi"("Priority? (F)"=TRUE ("Priority?"), "Message"=T39 {"Command"=enum."Disconnect", "Data"=variant(dbl[] [])} ("MSG to Servo"), "Queue in"=w1060) -> ()  [unwired: 6 in, 3 out]
                        }
                        frame "Rot" {
                          n565 = Unbundle By Name(w1066) -> ("Angle_C"=w1064:refnum<queue>)
                          n566 = call "Put in mailbox.vi"("Priority? (F)"=TRUE ("Priority?"), "Message"=cluster{"Command":T43, "Data":variant} {"Command"=enum."Disconnect", "Data"=variant} ("MSG to rotator"), "Queue in"=w1064) -> ()  [unwired: 6 in, 3 out]
                        }
                        frame "Ignore", Default {
                        }
                      }
                    }
                  }
                }
              }
            }
          }
          event "Stop": Value Change {
            n567 = event-data() -> ("NewVal"=w1072:bool)  [unwired: 1 in, 5 out]
            n568 = case shown="True" w1072 {
              tunnel: w1071 -> [_ w1076]
              tunnel: [_ w1075] -> w1070
              frame False {
              }
              frame True {
                # "Can not stop application just like that,\nAll modules must respond first, that they are done."
                n569 = control-ref of="Instr status"() -> (w1078:refnum<vi>)
                n570 = property class="Clust (strict)"(reference=w1078) -> ("Value"=w1073:T76)  [unwired: 1 in, 2 out]
                n571 = property class="Clust (strict)"(reference=w1078) -> ("Controls[]"=w1079:refnum<vi>[])  [unwired: 1 in, 2 out]
                n572 = Cluster To Array(cluster=w1073) -> (array=w1077:bool[])
                n573 = Or Array Elements(Boolean array=w1077) -> (logical OR=w1074:bool)
                n574 = case shown="False" w1074 {
                  tunnel: w1073 -> [_ _]
                  tunnel: w1076 -> [w1138 _]
                  tunnel: [TRUE _] -> w1075
                  frame False {
                    n575 = Cluster To Array(cluster=w1138) -> (array=w1139:refnum<queue>[])
                    n576 = local read "loggersRef"() -> (w1130:refnum<file>)
                    n577 = for {
                      tunnel: w1139 -> [w1147] mode=indexing
                      tunnel: [w1140] -> w1135
                      n578 = Wait (ms)(milliseconds to wait=u32 100) -> ()  [unwired: 1 out]
                      n579 = Get Queue Status(queue=w1147) -> (queue out=w1146:refnum<queue>, error out=w1141:errorcluster, # elements in queue=w1144:i32)  [unwired: 2 in, 5 out]
                      n580 = Less Or Equal?(x=w1144, y=0) -> (x <= y?=w1142:bool)
                      n581 = Release Queue(queue=w1146, force destroy? (F)=w1142, error in (no error)=w1141) -> (error out=w1140:errorcluster)  [unwired: 2 out]
                    }
                    n582 = Wait (ms)(milliseconds to wait=u32 2000) -> ()  [unwired: 1 out]
                    n583 = local read "Temperature log ref"() -> (w1134:refnum<file>)
                    n584 = call "Add actual date time to string.vi"("String in"="Program ended") -> ("String out"=w1131:string)  [unwired: 4 in]
                    n585 = call "Write in logger.vi"("String in"=w1131, "logger refnum"=w1130) -> ("refnum out"=w1129:refnum<file>)  [unwired: 2 in, 1 out]
                    n586 = local read "System config file path"() -> (w1128:path)
                    n587 = local read "Acquisition controls"() -> (w1125:T14)
                    n588 = local read "VID control"() -> (w1124:T17)
                    n589 = Close File(refnum=w1129, error in=w1135) -> (error out=w1133:errorcluster)  [unwired: 1 out]
                    n590 = Close File(refnum=w1134, error in=w1133) -> ()  [unwired: 2 out]
                    n591 = call "Open config file.vi"("MAG config file path"=w1128) -> ("error out"=w1126:errorcluster, "Refnum out"=w1127:T74)  [unwired: 7 in, 2 out]
                    n592 = Unbundle By Name(w1125) -> ("ACQ parameters"=w1121:T15)
                    n593 = call <userlib>:"Write Section Cluster__ogtk.vi"("error in (no error)"=w1126, "Section Formatted Cluster"=w1124, "refnum"=w1127) -> ("error out"=w1123:errorcluster, "dup refnum"=w1122:T74)  [unwired: 7 in]
                    n594 = local read "Instr info"() -> (w1116:T8)
                    n595 = call <userlib>:"Write Section Cluster__ogtk.vi"("error in (no error)"=w1123, "Section Formatted Cluster"=w1121, "refnum"=w1122) -> ("error out"=w1118:errorcluster, "dup refnum"=w1120:T74)  [unwired: 7 in]
                    n596 = call <userlib>:"Write Section Cluster__ogtk.vi"("error in (no error)"=w1118, "Section Formatted Cluster"=w1116, "refnum"=w1120) -> ("error out"=w1117:errorcluster, "dup refnum"=w1119:T74)  [unwired: 7 in]
                    n597 = call <vilib>:"Close Config Data.vi"("error in (no error)"=w1117, "refnum"=w1119) -> ()  [unwired: 8 in, 2 out]
                  }
                  frame True {
                  }
                }
                n598 = for {
                  tunnel: w1079 -> [w1085] mode=indexing
                  tunnel: w1076 -> [w1083]
                  n599 = property class="Ctl"(reference=w1085) -> ("Label.Text"=w1084:string, "Value"=w1082:variant)  [unwired: 1 in, 2 out]
                  n600 = Variant To Data(type=FALSE, Variant=w1082) -> (data=w1080:bool)  [unwired: 1 in, 1 out]
                  n601 = case shown="True" w1080 {
                    tunnel: w1084 -> [_ w1087]
                    tunnel: w1083 -> [_ w1086]
                    frame False {
                    }
                    frame True {
                      n602 = case shown="\"Rot\"" w1087 {
                        tunnel: w1086 -> [w1091 w1095 w1099 w1103 w1107 w1111 w1115 _]
                        frame "Mag" {
                          n603 = Unbundle By Name(w1091) -> ("Field_C"=w1089:refnum<queue>)
                          n604 = call "Put in mailbox.vi"("Priority? (F)"=TRUE ("Priority?"), "Message"=T37 {"Command"=enum."Eval temperatures", "Data"=variant} ("MSG to magnet"), "Queue in"=w1089) -> ()  [unwired: 6 in, 3 out]
                        }
                        frame "SMU" {
                          n605 = Unbundle By Name(w1095) -> ("Mod_M"=w1093:refnum<queue>)
                          n606 = call "Put in mailbox.vi"("Priority? (F)"=TRUE ("Priority?"), "Message"=T40 {"Command"=enum."End", "Data"=variant} ("MSG to Source meter"), "Queue in"=w1093) -> ()  [unwired: 6 in, 3 out]
                        }
                        frame "VTI" {
                          n607 = Unbundle By Name(w1099) -> ("Tmp_C"=w1097:refnum<queue>)
                          n608 = call "Put in mailbox.vi"("Priority? (F)"=TRUE ("Priority?"), "Message"=T53 {"Command"=enum."End", "Data"=variant} ("MSG for VTI"), "Queue in"=w1097) -> ()  [unwired: 6 in, 3 out]
                        }
                        frame "THz" {
                          n609 = Unbundle By Name(w1103) -> ("MW_C"=w1101:refnum<queue>)
                          n610 = call "Put in mailbox.vi"("Priority? (F)"=TRUE ("Priority?"), "Message"=T46 {"Command"=enum."End", "Data"=variant} ("Incoming msg"), "Queue in"=w1101) -> ()  [unwired: 6 in, 3 out]
                        }
                        frame "ACQ" {
                          n611 = Unbundle By Name(w1107) -> ("Data_Aq"=w1105:refnum<queue>)
                          n612 = call "Put in mailbox.vi"("Priority? (F)"=TRUE ("Priority?"), "Message"=T50 {"Command"=enum."End", "Data"=variant} ("MSG for  ACQ"), "Queue in"=w1105) -> ()  [unwired: 6 in, 3 out]
                        }
                        frame "Serv" {
                          n613 = Unbundle By Name(w1111) -> ("Table_C"=w1109:refnum<queue>)
                          n614 = call "Put in mailbox.vi"("Priority? (F)"=TRUE ("Priority?"), "Message"=T39 {"Command"=enum."End", "Data"=variant(dbl[] [])} ("MSG to Servo"), "Queue in"=w1109) -> ()  [unwired: 6 in, 3 out]
                        }
                        frame "Rot" {
                          n615 = Unbundle By Name(w1115) -> ("Angle_C"=w1113:refnum<queue>)
                          n616 = call "Put in mailbox.vi"("Priority? (F)"=TRUE ("Priority?"), "Message"=cluster{"Command":T43, "Data":variant} {"Command"=enum."End", "Data"=variant} ("MSG to rotator"), "Queue in"=w1113) -> ()  [unwired: 6 in, 3 out]
                        }
                        frame "Ignore", Default {
                        }
                      }
                    }
                  }
                }
              }
            }
          }
          event "Re-connect instruments": Value Change {
            n617 = event-data() -> ()  [unwired: 1 in, 6 out]
            n618 = local read "System config file path"() -> (w1149:path)
            n619 = case shown="\"MAG\"" "Select module" {
              tunnel: w1154 -> [w1159 w1168 w1205 _ w1215 w1227 w1229 w1241 w1252]
              tunnel: w1149 -> [w1158 _ w1200 _ _ w1219 _ _ _]
              tunnel: w1153 -> [w1157 w1169 w1206 w1207 w1216 w1228 w1234 w1242 w1249]
              tunnel: [w1157 w1169 w1206 w1207 w1216 w1228 w1234 w1242 w1249] -> w1152
              tunnel: "Use previous settings" -> [_ w1160 _ _ _ _ _ _ _]
              frame "All", Default {
                n620 = call "Send message to initialize all modules.vi"("System config file path"=w1158, "Messenger referencies"=w1159) -> ()  [unwired: 10 in]
                n621 = property on="Select module" class="Enum (strict)"("DisabledEnum"=T33."Enabled" ("Disabled")) -> ()  [unwired: 2 in, 2 out]
              }
              frame "ACQ" {
                w1161 = T50 {"Command"=enum."Initialize", "Data"=variant} ("MSG for  ACQ")
                n622 = Unbundle By Name(w1168) -> ("Data_Aq"=w1165:refnum<queue>)
                n623 = Bundle By Name(cluster=w1161, "Command"=MFLI_command_enum."Initialize", "Data"="MF-DEV4029") -> (w1166:T50)
                n624 = call "Put in mailbox.vi"("Priority? (F)"=TRUE, "Message"=w1166, "Queue in"=w1165) -> ("Queue out"=w1162:refnum<queue>)  [unwired: 6 in, 2 out]
                n625 = case shown="True" w1160 {
                  tunnel: w1162 -> [_ w1191]
                  tunnel: w1161 -> [_ w1189]
                  frame False {
                  }
                  frame True {
                    w1178 = T47 {"parameter"=enum."filter_order [-]", "value"=0.0} ("Parameter to set")
                    n626 = local read "Acquisition controls"() -> (w1187:T14)
                    n627 = Unbundle By Name(w1187) -> ("ACQ parameters"=w1174:T15)
                    n628 = Unbundle By Name(w1174) -> ("Filter order"=w1186:dbl, "Filter tau [ms]"=w1185:dbl, "F_Mod [kHz]"=w1184:dbl, "Amp_Mod [mV]"=w1183:dbl)
                    n629 = Divide(x=w1183, y=1000.0) -> (x/y=w1182:dbl)
                    n630 = Bundle(cluster=w1178, "parameter"=MFLI_node."osc_freq [kHz]", "value"=w1184) -> (w1176:T47)
                    n631 = Bundle(cluster=w1178, "parameter"=MFLI_node."filter_constant [ms]", "value"=w1185) -> (w1177:T47)
                    n632 = Bundle(cluster=w1178, "parameter"=MFLI_node."out_ampl [V]", "value"=w1182) -> (w1180:T47)
                    n633 = Bundle(cluster=w1178, "parameter"=MFLI_node."filter_order [-]", "value"=w1186) -> (w1179:T47)
                    n634 = Build Array(w1179, w1177, w1176, w1180) -> (w1175:T47[])
                    n635 = Bundle By Name(cluster=w1189, "Command"=MFLI_command_enum."Set individual parameters", "Data"=w1175) -> (w1190:T50)
                    n636 = call "Put in mailbox.vi"("Message"=w1190, "Queue in"=w1191) -> ()  [unwired: 7 in, 3 out]
                  }
                }
              }
              frame "MAG" {
                n637 = call "Read magnet system configuration.vi"("MAG config file path"=w1200) -> ("error out"=w1202:errorcluster, "Magnet Constantsout"=w1198:T77)  [unwired: 8 in, 1 out]
                n638 = Unbundle By Name(w1205) -> ("Field_C"=w1201:refnum<queue>)
                n639 = Unbundle By Name(w1198) -> ("Maximum field [T]"=w1197:dbl, "Field Constant [T/A]"=w1195:dbl, "Ramp limits [A/s]"=w1196:dbl[])
                n640 = Bundle By Name(cluster=T37 {"Command"=enum."Connect", "Data"=variant(enum16{"Ramping", "Perzistant"} enum."Ramping")} ("MSG to magnet"), "Data"=w1198) -> (w1203:T37)
                n641 = Index Array(array=w1196) -> (element=w1194:dbl)  [unwired: 1 in]
                n642 = call "Put in mailbox.vi"("Priority? (F)"=TRUE, "error in (no error)"=w1202, "Message"=w1203, "Queue in"=w1201) -> ()  [unwired: 5 in, 3 out]
                n643 = Compound Arithmetic op=MULTIPLY(w1195, w1194, 1000.0 ("value")) -> (w1192:dbl)
                n644 = property on="Set Field [T]" class="DigNum (strict)"("Maximum"=w1197) -> ()  [unwired: 2 in, 2 out]
                n645 = property on="Desired ramp\nrate [mT/s]" class="DigNum (strict)"("Maximum"=w1192) -> ()  [unwired: 2 in, 2 out]
              }
              frame "None" {
              }
              frame "ROT" {
                n646 = disable-structure shown="TARGET_BITNESS==64, Default" {
                  disable-tunnel: [path "C:/Program Files/National Instruments/LabVIEW 2024/instr.lib/ANC350/Win32/anc350v4.dll" ("File Path Control") path "C:/Programs/Debug/ANC350 lib/Software_ANC350v4/Windows/ANC350_Library/lib64/anc350v4.dll" ("File Path Control")] -> w1208
                  frame condition #0 {
                  }
                  frame condition #1 (active) {
                  }
                }
                n647 = Unbundle By Name(w1215) -> ("Angle_C"=w1212:refnum<queue>)
                n648 = Build Array(w1208, path "C:/Programs/Debug/HFEPR spectrometer SW 2024/Multi-HFEPR app/SystemData/ANRv51-C4-124.LUT" ("File Path Control")) -> (w1209:path[])
                n649 = Bundle By Name(cluster=T42 {"Command"=enum."Initialize", "Data"=variant} ("MSG to rotator"), "Command"=Rotator_commands."Initialize", "Data"=w1209) -> (w1214:T42)
                n650 = call "Put in mailbox.vi"("Message"=w1214, "Queue in"=w1212) -> ()  [unwired: 7 in, 3 out]
              }
              frame "SERV" {
                n651 = Unbundle By Name(w1227) -> ("Table_C"=w1220:refnum<queue>)
                n652 = call "Servo Read system configuration.vi"("MAG config file path"=w1219) -> ("error out"=w1224:errorcluster, "IP addresses"=w1225:string[])  [unwired: 8 in, 1 out]
                n653 = Bundle By Name(cluster=T39 {"Command"=enum."Initialize", "Data"=variant(dbl[] [])} ("MSG to Servo"), "Command"=Servo_commands."Initialize", "Data"=w1225) -> (w1226:T39)
                n654 = call "Put in mailbox.vi"("Priority? (F)"=TRUE, "error in (no error)"=w1224, "Message"=w1226, "Queue in"=w1220) -> ()  [unwired: 5 in, 3 out]
              }
              frame "SMU" {
                n655 = Unbundle By Name(w1229) -> ("Mod_M"=w1230:refnum<queue>)
                n656 = Bundle By Name(cluster=T40 {"Command"=enum."Connect", "Data"=variant} ("MSG to Source meter"), "Data"="USB0::0x05E6::0x2450::04405250::INSTR") -> (w1232:T40)
                n657 = call "Put in mailbox.vi"("Message"=w1232, "Queue in"=w1230) -> ()  [unwired: 7 in, 3 out]
              }
              frame "THz" {
                n658 = case shown="False" TRUE {
                  tunnel: [w1244 T54[] [{"Lower limit [GHz]"=8.0, "Upper limit [GHz]"=20.0, "Device name"="VDIS0122", "Connection"="", "Description"="VDI Synth", "Connected"=FALSE, "Last settings"="", "Operation mode"=enum."Disabled", "Enable ch 1"=FALSE, "Enable ch 2"=FALSE}, {"Lower limit [GHz]"=8.0, "Upper limit [GHz]"=20.0, "Device name"="VDIYT7", "Connection"="", "Description"="VDI Tracking", "Connected"=FALSE, "Last settings"="", "Operation mode"=enum."Disabled", "Enable ch 1"=FALSE, "Enable ch 2"=FALSE}] ("Array")] -> w1236
                  frame False {
                    n659 = Bundle By Name(cluster=T54 {"Lower limit [GHz]"=0.0, "Upper limit [GHz]"=0.0, "Device name"="", "Connection"="", "Description"="", "Connected"=FALSE, "Last settings"="", "Operation mode"=enum."Disabled", "Enable ch 1"=FALSE, "Enable ch 2"=FALSE} ("Configuration"), "Connection"="USB0::0x03EB::0xAFFF::848-0B4424003-0065::INSTR") -> (w1243:T54)
                    n660 = Build Array(w1243) -> (w1244:T54[])
                  }
                  frame True {
                  }
                }
                n661 = Unbundle By Name(w1241) -> ("MW_C"=w1238:refnum<queue>)
                n662 = Bundle By Name(cluster=T46 {"Command"=enum."Connect", "Data"=variant} ("Incoming msg"), "Data"=w1236) -> (w1240:T46)
                n663 = call "Put in mailbox.vi"("Priority? (F)"=TRUE, "Message"=w1240, "Queue in"=w1238) -> ()  [unwired: 6 in, 3 out]
              }
              frame "VTI" {
                n664 = Unbundle By Name(w1252) -> ("Tmp_C"=w1251:refnum<queue>)
                n665 = Bundle By Name(cluster=T53 {"Command"=enum."Initialize", "Data"=variant} ("MSG for VTI"), "Command"=TC_commands."Initialize", "Data"="COM4") -> (w1250:T53)
                n666 = call "Put in mailbox.vi"("Message"=w1250, "Queue in"=w1251) -> ()  [unwired: 7 in, 3 out]
              }
            }
          }
        }
        "Logger" <- w101
        n667 = Index Array(array=w101) -> (element=w106:string)  [unwired: 1 in]
        n668 = Bundle By Name(cluster=w105, "Last log"=w106) -> (w103:T27)
        n669 = local write "Infobar"(w103) -> ()
      }
      frame "Check message" {
        # "actual measurement"
        n670 = Unbundle By Name(w1259) -> ("TOP"=w1276:refnum<queue>)
        n671 = call "Receive message by TOP.vi"("timeout (100)"=5 ("timeout in ms (-1)"), "Mailbox in"=w1276) -> ("error out"=w1269:errorcluster, "timed out?"=w1271:bool, "Unread"=w1268:i32, "MSG packet"=w1275:T78)  [unwired: 6 in]
        n672 = Or(x=w1271, y=w1269) -> (x .or. y?=w1270:bool)
        n673 = case shown="False" w1270 {
          tunnel: w1275 -> [w1298 _]
          tunnel: w1273 -> [w1295 w2439]
          tunnel: [w1294 w2439] -> w1272
          tunnel: w1256 -> [w1289 w2438]
          tunnel: [w1288 w2438] -> w1261
          tunnel: w1260 -> [w1291 _]
          tunnel: w1259 -> [w1290 _]
          tunnel: w1258 -> [w1287 w2437]
          tunnel: [w1286 w2437] -> w1257
          frame False {
            n674 = Unbundle By Name(w1298) -> ("Time"=w1293:timestamp, "Module"=w1297:T79, "Response"=w1296:string, "Data"=w1292:variant)
            n675 = case "Message from module:" shown="\"Acquisition\"" w1297 {
              selector: w1297 -> [_ _ _ _ _ _ w2256 w2433]
              tunnel: w1296 -> [w1310 w1567 w1686 w1814 w1951 w2050 w2260 w2431]
              tunnel: w1292 -> [w1309 w1564 w1685 w1815 w1950 w2053 w2259 _]
              tunnel: w1295 -> [w1308 w1566 w1682 w1812 w1949 w2052 w2258 w2436]
              tunnel: [w1307 w1565 w1681 w1813 w1948 w2051 w2257 w2435] -> w1294
              tunnel: w1293 -> [w1306 w1563 w1684 w1809 w1943 w2044 w2249 _]
              tunnel: w1289 -> [w1305 w1561 w1683 w1816 w1941 w2049 w2255 w2429]
              tunnel: [w1304 w1562 w1683 w1817 w1947 w2049 w2255 w2429] -> w1288
              tunnel: w1291 -> [_ w1560 _ _ _ _ _ _]
              tunnel: w1290 -> [w1299 w1555 w1676 _ _ _ _ _]
              tunnel: w1287 -> [w1303 w1559 w1677 w1811 w1946 w2048 w2253 w2428]
              tunnel: [w1301 w1557 w1678 w1808 w1945 w2047 w2251 w2428] -> w1286
              frame "Magnet" {
                # "list of responses:"
                n676 = Unbundle By Name(w1303) -> ("Magnet"=w1302:T80)
                n677 = case shown="\"Initialize\"" w1310 {
                  selector: w1310 -> [w1317 _ _ _ _ _ _ w1461 _ _ _ _]
                  tunnel: w1309 -> [w1313 w1360 w1374 w1385 w1407 w1436 w1446 w1465 w1497 w1527 _ _]
                  tunnel: w1308 -> [w1315 w1357 w1367 w1381 w1391 w1428 w1441 w1458 w1480 w1528 w1532 w1544]
                  tunnel: [w1316 w1340 w1368 w1380 w1390 w1427 w1442 w1457 w1481 w1528 w1531 w1543] -> w1307
                  tunnel: w1306 -> [_ _ _ _ w1394 _ _ _ w1473 w1523 _ _]
                  tunnel: w1305 -> [w1312 w1345 w1366 w1377 w1397 w1424 w1440 w1456 w1467 w1524 w1534 w1546]
                  tunnel: [w1312 w1345 w1366 w1377 w1396 w1424 w1440 w1456 w1478 w1524 w1534 w1546] -> w1304
                  tunnel: w1302 -> [w1311 w1344 w1365 w1375 w1395 w1423 w1439 w1455 w1477 w1513 w1530 w1542]
                  tunnel: [w1311 w1339 w1364 w1375 w1393 w1423 w1439 w1454 w1472 w1513 w1530 w1542] -> w1300
                  tunnel: w1299 -> [_ _ _ _ _ _ _ _ w1466 _ _ _]
                  frame "ignore", Default {
                    n678 = Match Pattern(string=w1317, regular expression="Error") -> (after substring=w1314:string, offset past match=w1319:i32)  [unwired: 1 in, 2 out]
                    n679 = Greater Or Equal To 0?(x=w1319) -> (x >= 0?=w1318:bool)
                    n680 = case shown="True" w1318 {
                      tunnel: w1315 -> [w1323 w1332]
                      tunnel: w1317 -> [w1322 w1331]
                      tunnel: [w1321 w1333] -> w1316
                      tunnel: w1314 -> [_ _]
                      tunnel: w1313 -> [_ w1329]
                      frame False {
                        n681 = call "simple Shift string array.vi"("Element in"=w1322, "Array in"=w1323) -> ("Array out"=w1321:string[])  [unwired: 8 in, 1 out]
                      }
                      frame True {
                        n682 = Variant To Data(type=errorcluster {"status"=FALSE, "code"=0, "source"=""} ("error constant"), Variant=w1329) -> (data=w1327:errorcluster)  [unwired: 1 in, 1 out]
                        n683 = Unbundle By Name(w1327) -> ("source"=w1326:string)
                        n684 = call <vilib>:"Space Constant.vi"() -> ("String"=w1330:string)
                        n685 = Concatenate Strings(w1331, w1330, w1326) -> (w1324:string)
                        n686 = local read "loggersRef"() -> (w1325:refnum<file>)
                        n687 = call "Write in logger.vi"("String in"=w1324, "logger refnum"=w1325) -> ()  [unwired: 2 in, 2 out]
                        n688 = call "simple Shift string array.vi"("Element in"=w1324, "Array in"=w1332) -> ("Array out"=w1333:string[])  [unwired: 8 in, 1 out]
                      }
                    }
                  }
                  frame "Initialize" {
                    w1352 = TRUE ("PSU")
                    w1351 = T33."Enabled" ("Disabled")
                    n689 = Variant To Data(type="", Variant=w1360) -> (data=w1334:string)  [unwired: 1 in, 1 out]
                    n690 = local read "Instr status"() -> (w1355:T1)
                    n691 = Bundle By Name(cluster=w1355, "Mag"=w1352) -> (w1359:T1)
                    n692 = Match Pattern(string=w1334, regular expression="SMS120") -> (match substring=w1337:string)  [unwired: 1 in, 3 out]
                    n693 = Unbundle By Name(w1355) -> ("THz"=w1354:bool, "MFLI"=w1353:bool)
                    n694 = local write "Instr status"(w1359) -> ()
                    n695 = control-ref of="Magnet controls"() -> (w1356:refnum<vi>)
                    n696 = Compound Arithmetic op=AND(w1354, w1353, w1352) -> (w1350:bool)
                    n697 = call "Add actual date time to string.vi"("String in"="Magnet module initialized") -> ("String out"=w1348:string)  [unwired: 4 in]
                    n698 = Select(t=w1351, s=w1350, f=T33."Disabled and Grayed Out" ("Disabled")) -> (s? t:f=w1346:T33)
                    n699 = local read "loggersRef"() -> (w1347:refnum<file>)
                    n700 = property class="Clust (strict)"(reference=w1356, "DisabledEnum"=w1351) -> ()  [unwired: 1 in, 2 out]
                    n701 = Concatenate Strings(w1348, "\r\n", w1334) -> (w1336:string)
                    n702 = call "simple Shift string array.vi"("Element in"=w1348, "Array in"=w1357) -> ("Array out"=w1341:string[])  [unwired: 8 in, 1 out]
                    n703 = call "Write in logger.vi"("String in"=w1336, "logger refnum"=w1347) -> ()  [unwired: 2 in, 2 out]
                    n704 = call "Add actual date time to string.vi"("String in"=w1334) -> ("String out"=w1342:string)  [unwired: 4 in]
                    n705 = call "simple Shift string array.vi"("Element in"=w1342, "Array in"=w1341) -> ("Array out"=w1340:string[])  [unwired: 8 in, 1 out]
                    n706 = property on="Run FDMR+ btn" class="Bool (strict)"("DisabledEnum"=w1346) -> ()  [unwired: 2 in, 2 out]
                    n707 = Bundle By Name(cluster=w1344, "PSU"=w1337) -> (w1339:T80)
                  }
                  frame "TM revision" {
                    n708 = Variant To Data(type=T55 {"Instr Serial Number"="", "Instr Driver Revision"="", "Instr Firmware Revision"="", "Instr Model Number"=""} ("TM Revision"), Variant=w1374) -> (data=w1372:T55)  [unwired: 1 in, 1 out]
                    n709 = Unbundle By Name(w1372) -> ("Instr Model Number"=w1363:string)
                    n710 = call <vilib>:"Space Constant.vi"() -> ("String"=w1370:string)
                    n711 = Concatenate Strings("Temperature monitor:" ("string"), w1370, w1363) -> (w1369:string)
                    n712 = Bundle By Name(cluster=w1365, "T monitor"=w1363) -> (w1364:T80)
                    n713 = call "Add actual date time to string.vi"("String in"=w1369) -> ("String out"=w1361:string)  [unwired: 4 in]
                    n714 = local read "loggersRef"() -> (w1362:refnum<file>)
                    n715 = call "simple Shift string array.vi"("Element in"=w1361, "Array in"=w1367) -> ("Array out"=w1368:string[])  [unwired: 8 in, 1 out]
                    n716 = call "Write in logger.vi"("String in"=w1361, "logger refnum"=w1362) -> ()  [unwired: 2 in, 2 out]
                  }
                  frame "Initialization error" {
                    n717 = Variant To Data(type=errorcluster {"status"=FALSE, "code"=0, "source"=""} ("error constant"), Variant=w1385) -> (data=w1383:errorcluster, error out=w1376:errorcluster)  [unwired: 1 in]
                    n718 = Unbundle By Name(w1383) -> ("source"=w1382:string)
                    n719 = call "Add actual date time to string.vi"("String in"=w1382) -> ("String out"=w1379:string)  [unwired: 4 in]
                    n720 = call "simple Shift string array.vi"("Element in"=w1379, "Array in"=w1381) -> ("Array out"=w1380:string[])  [unwired: 8 in, 1 out]
                    n721 = local read "loggersRef"() -> (w1378:refnum<file>)
                    n722 = call "Write in logger.vi"("error in"=w1376, "String in"=w1379, "logger refnum"=w1378) -> ()  [unwired: 1 in, 2 out]
                  }
                  frame "Update" {
                    n723 = Variant To Data(type=T56 {"Desired"={"Field [T]"=0.0, "Ramp [T/s]"=0.0, "Custom Ramp?"=TRUE, "Mode"=enum."Persistant"}, "Actual"={"Mode"=enum."Persistant", "Ramping output"=enum."At Target", "Ready for change"=FALSE, "Switch heater"=FALSE, "Cooler Overheat"=FALSE, "Coil overheat"=FALSE, "Energized"=FALSE, "Output [T]"=0.0, "Field [T]"=0.0, "Ramp[T/s]"=0.0, "Switch\ntemperature [K]"=1.0, "Voltage [V]"=0.0, "Current direction"=FALSE}} ("output cluster"), Variant=w1407) -> (data=w1389:T56)  [unwired: 1 in, 1 out]
                    n724 = Unbundle By Name(w1389) -> ("Actual.Ready for change"=w1386:bool, "Actual.Mode"=w1387:T58, "Actual.Field [T]"=w1388:dbl)
                    n725 = local read "Instr status"() -> (w1405:T1)
                    n726 = local read "Magnet controls"() -> (w1400:T19)
                    n727 = Bundle By Name(cluster=w1405, "Mag"=TRUE ("PSU")) -> (w1404:T1)
                    n728 = Bundle By Name(cluster=w1397, "Field [T]"=w1388) -> (w1396:T27)
                    n729 = local write "Instr status"(w1404) -> ()
                    n730 = call "Magnet update rewiring.vi"("output cluster"=w1389, "Time"=w1394, "Magnet in"=w1395, "Magnet controls in"=w1400) -> ("Magnet out"=w1393:T80, "Magnet controls out"=w1399:T19)  [unwired: 6 in]
                    n731 = local write "Magnet controls"(w1399) -> ()
                    n732 = case shown="\"Quenched\"" w1387 {
                      selector: w1387 -> [_ _ _ w1416]
                      tunnel: [w1409 w1410 w1413 w1418] -> w1390
                      tunnel: w1391 -> [w1409 w1410 w1413 w1417]
                      tunnel: [T33."Enabled" ("Disabled") T33."Disabled and Grayed Out" ("f") T33."Disabled and Grayed Out" ("f") T33."Disabled and Grayed Out" ("f")] -> w1392
                      frame "Persistant", Default {
                      }
                      frame "Switching" {
                      }
                      frame "Ramping" {
                      }
                      frame "Quenched" {
                        n733 = Format Into String(w1416) -> (resulting string=w1415:string)  [unwired: 3 in, 1 out]
                        n734 = call "Add actual date time to string.vi"("String in"=w1415) -> ("String out"=w1419:string)  [unwired: 4 in]
                        n735 = local read "loggersRef"() -> (w1420:refnum<file>)
                        n736 = call "simple Shift string array.vi"("Element in"=w1419, "Array in"=w1417) -> ("Array out"=w1418:string[])  [unwired: 8 in, 1 out]
                        n737 = call "Write in logger.vi"("String in"=w1419, "logger refnum"=w1420) -> ()  [unwired: 2 in, 2 out]
                      }
                    }
                    n738 = Select(t=T33."Enabled" ("Disabled"), s=w1386, f=T33."Disabled and Grayed Out") -> (s? t:f=w1398:T33)
                    n739 = property on="Mode switch" class="Bool (strict)"("DisabledEnum"=w1398) -> ()  [unwired: 2 in, 2 out]
                    n740 = property on="Equalize" class="Bool (strict)"("DisabledEnum"=w1392) -> ()  [unwired: 2 in, 2 out]
                    n741 = property on="Discharge" class="Bool (strict)"("DisabledEnum"=w1392) -> ()  [unwired: 2 in, 2 out]
                  }
                  frame "Update error" {
                    # "ReInitialize Magnet?"
                    n742 = Variant To Data(type=errorcluster {"status"=FALSE, "code"=0, "source"=""} ("error in (no error)"), Variant=w1436) -> (data=w1434:errorcluster)  [unwired: 1 in, 1 out]
                    n743 = Unbundle By Name(w1434) -> ("source"=w1431:string)
                    n744 = local read "Instr status"() -> (w1430:T1)
                    n745 = Bundle By Name(cluster=w1430, "Mag"=FALSE ("PSU")) -> (w1429:T1)
                    n746 = local write "Instr status"(w1429) -> ()
                    n747 = Concatenate Strings("Magnet Update error: " ("String in"), w1431) -> (w1432:string)
                    n748 = property on="Magnet controls" class="Clust (strict)"("DisabledEnum"=T33."Disabled and Grayed Out" ("Disabled")) -> ()  [unwired: 2 in, 2 out]
                    n749 = local read "loggersRef"() -> (w1422:refnum<file>)
                    n750 = call "Add actual date time to string.vi"("String in"=w1432) -> ("String out"=w1421:string)  [unwired: 4 in]
                    n751 = call "Write in logger.vi"("String in"=w1421, "logger refnum"=w1422) -> ()  [unwired: 2 in, 2 out]
                    n752 = call "simple Shift string array.vi"("Element in"=w1421, "Array in"=w1428) -> ("Array out"=w1427:string[])  [unwired: 8 in, 1 out]
                  }
                  frame "Switch mode acepted" {
                    n753 = Variant To Data(type=Magnet_mode_public."Ramping" ("Operation mode"), Variant=w1446) -> (data=w1444:T34)  [unwired: 1 in, 1 out]
                    n754 = case shown="\"Persistant\"" w1444 {
                      tunnel: ["Switching to ramping mode" "Switching to perzistant mode"] -> w1443
                      frame "Ramping", Default {
                      }
                      frame "Persistant" {
                      }
                    }
                    n755 = call "Add actual date time to string.vi"("String in"=w1443) -> ("String out"=w1437:string)  [unwired: 4 in]
                    n756 = local read "loggersRef"() -> (w1438:refnum<file>)
                    n757 = call "simple Shift string array.vi"("Element in"=w1437, "Array in"=w1441) -> ("Array out"=w1442:string[])  [unwired: 8 in, 1 out]
                    n758 = call "Write in logger.vi"("String in"=w1437, "logger refnum"=w1438) -> ()  [unwired: 2 in, 2 out]
                  }
                  frame "Ramping" {
                    n759 = Variant To Data(type=T35 {"Field [T]"=0.0, "Ramp [T/s]"=0.0, "Custom Ramp?"=TRUE, "Mode"=enum."Persistant"} ("Set Field"), Variant=w1465) -> (data=w1463:T35)  [unwired: 1 in, 1 out]
                    n760 = Unbundle By Name(w1463) -> ("Field [T]"=w1460:dbl, "Ramp [T/s]"=w1452:dbl)
                    n761 = Multiply(x=w1452, y=1000.0) -> (x*y=w1451:dbl)
                    n762 = Bundle By Name(cluster=w1455, "Ramp [mT/s]"=w1451) -> (w1454:T80)
                    n763 = Format Into String(format string=" B= %f [T] Ramp= %f [mT/s]", initial string=w1461, w1460, w1451) -> (resulting string=w1459:string)  [unwired: 1 in, 1 out]
                    n764 = call "Add actual date time to string.vi"("String in"=w1459) -> ("String out"=w1449:string)  [unwired: 4 in]
                    n765 = local read "loggersRef"() -> (w1450:refnum<file>)
                    n766 = call "simple Shift string array.vi"("Element in"=w1449, "Array in"=w1458) -> ("Array out"=w1457:string[])  [unwired: 8 in, 1 out]
                    n767 = call "Write in logger.vi"("String in"=w1449, "logger refnum"=w1450) -> ()  [unwired: 2 in, 2 out]
                  }
                  frame "Set field" {
                    n768 = Unbundle By Name(w1467) -> ("Experiment state"=w1479:T28)
                    n769 = Unbundle By Name(w1466) -> ()  [unwired: 1 out]
                    n770 = local read "Magnet controls"() -> (w1495:T19)
                    n771 = Variant To Data(type=T35 {"Field [T]"=0.0, "Ramp [T/s]"=0.0, "Custom Ramp?"=TRUE, "Mode"=enum."Persistant"} ("Set Field"), Variant=w1497) -> (data=w1494:T35, error out=w1468:errorcluster)  [unwired: 1 in]
                    n772 = Unbundle By Name(w1477) -> ("Field [T]"=w1483:dbl)
                    n773 = Unbundle By Name(w1494) -> ("Field [T]"=w1488:dbl, "Ramp [T/s]"=w1476:dbl, "Custom Ramp?"=w1493:bool)
                    n774 = Unbundle By Name(w1495) -> ("Desired ramp\nrate [mT/s]"=w1492:dbl)
                    n775 = Not(x=w1493) -> (.not. x?=w1491:bool)
                    n776 = call <userlib>:"MGI Approximately Equal.vi"("Numeric 2"=w1492, "Numeric 1"=w1476) -> ("approx = ?"=w1490:bool)
                    n777 = Multiply(x=w1476, y=1000.0 ("x")) -> (x*y=w1474:dbl)
                    n778 = Or(x=w1491, y=w1490) -> (x .or. y?=w1487:bool)
                    n779 = case shown="False" w1487 {
                      tunnel: ["Warning: Custom ramp was adjusted" ""] -> w1485
                      frame False {
                      }
                      frame True {
                      }
                    }
                    n780 = Format Into String(format string="Setting magnetic field from %f [T ] to %f [T] with ramp %f [mT/s]", error in=w1468, w1483, w1488, w1474) -> (resulting string=w1486:string, error out=w1469:errorcluster)  [unwired: 1 in]
                    n781 = Concatenate Strings(w1486, "\r", w1485) -> (w1470:string)
                    n782 = call "Add actual date time to string.vi"("String in"=w1470) -> ("String out"=w1482:string)  [unwired: 4 in]
                    n783 = local read "loggersRef"() -> (w1471:refnum<file>)
                    n784 = Bundle By Name(cluster=w1477, "Last update"=w1473, "Ramp [mT/s]"=w1474) -> (w1472:T80)
                    n785 = Bundle By Name(cluster=w1467, "Experiment state"=w1479) -> (w1478:T27)
                    n786 = call "simple Shift string array.vi"("Element in"=w1482, "Array in"=w1480) -> ("Array out"=w1481:string[])  [unwired: 8 in, 1 out]
                    n787 = call "Write in logger.vi"("error in"=w1469, "String in"=w1470, "logger refnum"=w1471) -> ()  [unwired: 1 in, 2 out]
                  }
                  frame "Temperatures" {
                    w1507 = 8 ("length")
                    n788 = local read "Drift[K/min]"() -> (w1502:dbl[])
                    n789 = local read "Temperature monitor"() -> (w1508:T12)
                    n790 = Variant To Data(type=T59 {"First stage A [K]"=0.0, "Second stage A [K]"=0.0, "Firs stage B [K]"=0.0, "Second stage B [K]"=0.0, "Inner magnet [K]"=0.0, "Outer Magnet [K]"=0.0, "Switch [K]"=0.0, "Support plate [K]"=0.0, "Time stamp"=0.0} ("LSC218 sensors"), Variant=w1527) -> (data=w1510:T59)  [unwired: 1 in, 1 out]
                    n791 = property on="VTI" class="Clust (strict)"() -> ("Value"=w1522:T81)  [unwired: 2 in, 2 out]
                    n792 = Cluster To Array(cluster=w1510) -> (array=w1519:dbl[])
                    n793 = Unbundle By Name(w1513) -> ("Field [T]"=w1512:dbl)
                    n794 = local read "Temperature log ref"() -> (w1525:refnum<file>)
                    n795 = Unbundle By Name(w1522) -> ("VTI [K]"=w1515:dbl, "Sample [K]"=w1514:dbl, "Trap[K]"=w1521:dbl, "HePot [K]"=w1520:dbl)
                    n796 = Array Subset(array=w1519, length=w1507) -> (w1501:dbl[])  [unwired: 1 in]
                    n797 = Cluster To Array(cluster=w1508) -> (array=w1509:dbl[])
                    n798 = Array Subset(array=w1509, length=w1507) -> (w1500:dbl[])  [unwired: 1 in]
                    n799 = Subtract(x=w1501, y=w1500) -> (x-y=w1504:dbl[])
                    n800 = Divide(x=w1504, y=2.5) -> (x/y=w1505:dbl[])
                    n801 = Replace Array Subset(array=w1502, new element=w1505) -> (→"Drift[K/min]":dbl[])  [unwired: 1 in]
                    n802 = call "Bundle temperatures.vi"("Sample"=w1514, "VTI space"=w1515, "LSC218 sensors"=w1510) -> ("Tmp [K]"=→"Tmp [K]":T5)  [unwired: 8 in]
                    n803 = Build Array (concatenate)(w1501, w1515, w1514, w1521, w1520) -> (w1518:dbl[])
                    n804 = call "Log temperatures.vi"("LSC218 sensors"=w1510, "Time"=w1523, "Tmp logfile in"=w1525, "VTI"=w1515, "Sample"=w1514, "Trap"=w1521, "HePot"=w1520, "Field [T]"=w1512) -> ("Tmp logfile ref"=w1511:refnum<file>)  [unwired: 5 in, 2 out]
                    n805 = Array To Cluster(array=w1518) -> (cluster=w1517:T12)
                    n806 = local write "Temperature log ref"(w1511) -> ()
                    n807 = flat-sequence {
                      tunnel: w1517 -> [w1529]
                      tunnel: w1500 -> [_]
                      frame #0 {
                        "Temperature monitor" <- w1529
                      }
                    }
                  }
                  frame "End" {
                    n808 = local read "loggersRef"() -> (w1536:refnum<file>)
                    n809 = local read "Instr status"() -> (w1540:T1)
                    n810 = call "Add actual date time to string.vi"("String in"="Magnet ended") -> ("String out"=w1533:string)  [unwired: 4 in]
                    n811 = Bundle By Name(cluster=w1540, "Mag"=FALSE ("PSU")) -> (w1541:T1)
                    n812 = call "Write in logger.vi"("String in"=w1533, "logger refnum"=w1536) -> ()  [unwired: 2 in, 2 out]
                    n813 = local write "Instr status"(w1541) -> ()
                    n814 = control-ref of="Magnet controls"() -> (w1538:refnum<vi>)
                    n815 = call "simple Shift string array.vi"("Element in"=w1533, "Array in"=w1532) -> ("Array out"=w1531:string[])  [unwired: 8 in, 1 out]
                    n816 = property class="Clust (strict)"(reference=w1538, "DisabledEnum"=T33."Disabled and Grayed Out" ("Disabled")) -> ()  [unwired: 1 in, 2 out]
                  }
                  frame "Disconnect" {
                    n817 = local read "loggersRef"() -> (w1548:refnum<file>)
                    n818 = local read "Instr status"() -> (w1552:T1)
                    n819 = call "Add actual date time to string.vi"("String in"="Magnet disconencted") -> ("String out"=w1545:string)  [unwired: 4 in]
                    n820 = Bundle By Name(cluster=w1552, "Mag"=FALSE ("PSU")) -> (w1553:T1)
                    n821 = call "Write in logger.vi"("String in"=w1545, "logger refnum"=w1548) -> ()  [unwired: 2 in, 2 out]
                    n822 = local write "Instr status"(w1553) -> ()
                    n823 = control-ref of="Magnet controls"() -> (w1550:refnum<vi>)
                    n824 = call "simple Shift string array.vi"("Element in"=w1545, "Array in"=w1544) -> ("Array out"=w1543:string[])  [unwired: 8 in, 1 out]
                    n825 = property class="Clust (strict)"(reference=w1550, "DisabledEnum"=T33."Disabled and Grayed Out" ("Disabled")) -> ()  [unwired: 1 in, 2 out]
                  }
                }
                n826 = Bundle By Name(cluster=w1303, "Magnet"=w1300) -> (w1301:T8)
              }
              frame "Excitation" {
                n827 = Unbundle By Name(w1559) -> ("THz"=w1558:T82)
                n828 = Unbundle By Name(w1555) -> ("Data_Aq"=w1554:refnum<queue>)
                n829 = case shown="\"Disconnect\"" w1567 {
                  selector: w1567 -> [_ w1585 _ _ _ _]
                  tunnel: w1566 -> [w1570 w1600 w1603 w1635 w1648 w1664]
                  tunnel: [w1570 w1599 w1603 w1636 w1649 w1665] -> w1565
                  tunnel: w1564 -> [_ w1586 _ w1634 w1650 w1666]
                  tunnel: w1563 -> [_ _ _ w1612 w1652 w1668]
                  tunnel: w1561 -> [w1569 w1584 w1602 w1607 w1656 w1672]
                  tunnel: [w1569 w1584 w1602 w1604 w1656 w1672] -> w1562
                  tunnel: w1560 -> [_ _ _ _ _ _]
                  tunnel: w1558 -> [w1568 w1577 w1601 w1614 w1655 w1671]
                  tunnel: [w1568 w1576 w1601 w1613 w1654 w1670] -> w1556
                  tunnel: w1554 -> [_ _ _ w1605 _ _]
                  frame "Ignore", Default {
                  }
                  frame "Connect", "Initialize" {
                    w1572 = T33."Disabled and Grayed Out" ("Disabled")
                    w1571 = T33."Enabled" ("Disabled")
                    n830 = Variant To Data(type=w1585, Variant=w1586) -> (data=w1583:string, error out=w1573:errorcluster)  [unwired: 1 in]
                    n831 = Match Pattern(string=w1583, regular expression="VDI Synth") -> (after substring=w1575:string, offset past match=w1598:i32)  [unwired: 1 in, 2 out]
                    n832 = Match Pattern(string=w1583, regular expression="VDI Tracking") -> (after substring=w1574:string, offset past match=w1595:i32)  [unwired: 1 in, 2 out]
                    n833 = Greater Or Equal To 0?(x=w1595) -> (x >= 0?=w1581:bool)
                    n834 = Greater Or Equal To 0?(x=w1598) -> (x >= 0?=w1589:bool)
                    n835 = Bundle By Name(cluster=w1577, "Name"=w1575, "Description"=w1574) -> (w1576:T82)
                    n836 = Select(t=T33."Enabled", s=w1581, f=w1572) -> ()  [unwired: 1 out]
                    n837 = local read "Instr status"() -> (w1593:T1)
                    n838 = Bundle By Name(cluster=w1593, "THz"=w1589) -> (w1594:T1)
                    n839 = Unbundle By Name(w1593) -> ("Mag"=w1592:bool, "MFLI"=w1591:bool)
                    n840 = local write "Instr status"(w1594) -> ()
                    n841 = Compound Arithmetic op=AND(w1592, w1591, w1589) -> (w1590:bool)
                    n842 = Select(t=w1571, s=w1590, f=w1572) -> (s? t:f=w1587:T33)
                    n843 = local read "loggersRef"() -> (w1588:refnum<file>)
                    n844 = property on="VID control" class="Clust (strict)"("DisabledEnum"=w1571) -> ()  [unwired: 2 in, 2 out]
                    n845 = property on="Run FDMR+ btn" class="Bool (strict)"(error in=w1573, "DisabledEnum"=w1587) -> (error out=w1579:errorcluster)  [unwired: 1 in, 1 out]
                    n846 = call "Add actual date time to string.vi"("String in"=w1583) -> ("String out"=w1582:string)  [unwired: 4 in]
                    n847 = call "Write in logger.vi"("error in"=w1579, "String in"=w1582, "logger refnum"=w1588) -> ("error out"=w1578:errorcluster)  [unwired: 1 in, 1 out]
                    n848 = call "simple Shift string array.vi"("Element in"=w1583, "Array in"=w1600) -> ("Array out"=w1599:string[])  [unwired: 8 in, 1 out]
                    n849 = call <vilib>:"Clear Errors.vi"("error in (no error)"=w1578) -> ()  [unwired: 5 in, 2 out]
                  }
                  frame "Update" {
                  }
                  frame "Set parameters" {
                    n850 = Variant To Data(type=T45 {"Start [GHz]"=8.0, "End [GHz] "=8.0, "Sweep up\ntime [ms]"=0.0, "Sweep down\ntime [ms]"=0.0, "Intermidiate [MHz]"=0.0, "Reset trigger"=FALSE} ("Sweep parameters"), Variant=w1634) -> (data=w1623:T45, error out=w1624:errorcluster)  [unwired: 1 in]
                    n851 = Unbundle By Name(w1607) -> ("Experiment state"=w1608:T28)
                    n852 = local read "VID control"() -> (w1630:T17)
                    n853 = Unbundle By Name(w1623) -> ("Start [GHz]"=w1620:dbl, "End [GHz]"=w1619:dbl, "Sweep up\ntime [ms]"=w1618:dbl, "Intermidiate [MHz]"=w1622:dbl)
                    n854 = Unbundle By Name(w1630) -> ("AMC"=w1631:u16, "Multip"=w1632:u16)
                    n855 = case shown="\"Begin\"" w1608 {
                      selector: w1608 -> [w1637 _]
                      tunnel: [w1637 experiment_state."Acquisition" ("Experiment state")] -> w1606
                      tunnel: w1605 -> [_ w1638]
                      frame "Setup", Default {
                      }
                      frame "Begin" {
                        n856 = Build Array(T47 {"parameter"=enum."scope_trigEn", "value"=1.0} ("Parameter to set")) -> (w1642:T47[])
                        n857 = Bundle By Name(cluster=T50 {"Command"=enum."Set individual parameters", "Data"=variant} ("MSG for  ACQ"), "Data"=w1642) -> (w1641:T50)
                        n858 = call "Put in mailbox.vi"("Message"=w1641, "Queue in"=w1638) -> ()  [unwired: 7 in, 3 out]
                      }
                    }
                    n859 = Multiply(x=w1631, y=w1632) -> (x*y=w1621:u16)
                    n860 = Multiply(x=w1620, y=w1621) -> (x*y=w1611:dbl)
                    n861 = Multiply(x=w1619, y=w1621) -> (x*y=w1610:dbl)
                    n862 = Multiply(x=w1618, y=w1621) -> (x*y=w1617:dbl)
                    n863 = Multiply(x=w1622, y=w1621) -> (x*y=w1609:dbl)
                    n864 = Equal To 0?(x=w1617) -> (x = 0?=w1628:bool)
                    n865 = Select(t="CW", s=w1628, f="Sweep") -> (s? t:f=w1625:string)
                    n866 = Format Into String(format string="VDI set to %s mode at %f GHz ", error in=w1624, w1625, w1611) -> (resulting string=w1616:string)  [unwired: 1 in, 1 out]
                    n867 = Bundle By Name(cluster=w1614, "Last update"=w1612, "Start [GHz]"=w1611, "End [GHz]"=w1610, "Im Freq[MHz]"=w1609) -> (w1613:T82)
                    n868 = call "Add actual date time to string.vi"("String in"=w1616) -> ("String out"=w1615:string)  [unwired: 4 in]
                    n869 = Bundle By Name(cluster=w1607, "Experiment state"=w1606) -> (w1604:T27)
                    n870 = call "simple Shift string array.vi"("Element in"=w1615, "Array in"=w1635) -> ("Array out"=w1636:string[])  [unwired: 8 in, 1 out]
                  }
                  frame "End" {
                    w1653 = "None" ("Master")
                    n871 = Variant To Data(type="", Variant=w1650) -> (data=w1645:string)  [unwired: 1 in, 1 out]
                    n872 = Bundle By Name(cluster=w1655, "Name"=w1653, "Description"=w1653, "Last update"=w1652) -> (w1654:T82)
                    n873 = property on="THz" class="Bool (strict)"("Value"=FALSE) -> ()  [unwired: 2 in, 2 out]
                    n874 = call "Add actual date time to string.vi"("String in"="Excitation module (VDI) ended") -> ("String out"=w1647:string)  [unwired: 4 in]
                    n875 = Concatenate Strings(w1647, "\r\n", w1645) -> (w1646:string)
                    n876 = local read "loggersRef"() -> (w1658:refnum<file>)
                    n877 = call "Write in logger.vi"("String in"=w1646, "logger refnum"=w1658) -> ()  [unwired: 2 in, 2 out]
                    n878 = call "simple Shift string array.vi"("Element in"=w1646, "Array in"=w1648) -> ("Array out"=w1649:string[])  [unwired: 8 in, 1 out]
                  }
                  frame "Disconnect" {
                    w1669 = "None" ("Master")
                    n879 = Variant To Data(type="", Variant=w1666) -> (data=w1661:string)  [unwired: 1 in, 1 out]
                    n880 = Bundle By Name(cluster=w1671, "Name"=w1669, "Description"=w1669, "Last update"=w1668) -> (w1670:T82)
                    n881 = property on="THz" class="Bool (strict)"("Value"=FALSE) -> ()  [unwired: 2 in, 2 out]
                    n882 = call "Add actual date time to string.vi"("String in"="Excitation module (VDI) Disconnected") -> ("String out"=w1663:string)  [unwired: 4 in]
                    n883 = Concatenate Strings(w1663, "\r\n", w1661) -> (w1662:string)
                    n884 = local read "loggersRef"() -> (w1674:refnum<file>)
                    n885 = call "Write in logger.vi"("String in"=w1662, "logger refnum"=w1674) -> ()  [unwired: 2 in, 2 out]
                    n886 = call "simple Shift string array.vi"("Element in"=w1662, "Array in"=w1664) -> ("Array out"=w1665:string[])  [unwired: 8 in, 1 out]
                  }
                }
                n887 = Bundle By Name(cluster=w1559, "THz"=w1556) -> (w1557:T8)
              }
              frame "Acquisition" {
                n888 = Unbundle By Name(w1677) -> ("MFLI"=w1680:T83)
                n889 = case shown="\"Get ModA\"" w1686 {
                  tunnel: w1685 -> [w1711 w1727 w1748 w1767 w1776 w1794 w1804 _]
                  tunnel: w1684 -> [w1690 w1719 w1742 w1764 w1775 _ _ _]
                  tunnel: [w1695 w1723 w1747 w1757 w1777 w1795 w1798 w1806] -> w1681
                  tunnel: w1682 -> [w1696 w1724 w1747 w1757 w1777 w1795 w1799 w1806]
                  tunnel: w1680 -> [w1691 w1720 w1745 w1755 w1773 w1791 w1796 w1805]
                  tunnel: [w1688 w1714 w1743 w1755 w1773 w1791 w1796 w1805] -> w1679
                  tunnel: w1676 -> [_ _ _ _ _ w1788 _ _]
                  frame "Initialize" {
                    w1703 = TRUE ("PSU")
                    w1702 = T33."Enabled" ("Disabled")
                    n890 = Variant To Data(type="", Variant=w1711) -> (data=w1689:string)  [unwired: 1 in, 1 out]
                    n891 = Bundle By Name(cluster=w1691, "Last update"=w1690, "Lock-in"=w1689, "Multimeter"="Unknown") -> (w1688:T83)
                    n892 = local read "Instr status"() -> (w1706:T1)
                    n893 = Bundle By Name(cluster=w1706, "MFLI"=w1703) -> (w1708:T1)
                    n894 = Unbundle By Name(w1706) -> ("THz"=w1705:bool, "Mag"=w1704:bool)
                    n895 = local write "Instr status"(w1708) -> ()
                    n896 = control-ref of="Acquisition controls"() -> (w1707:refnum<vi>)
                    n897 = Compound Arithmetic op=AND(w1705, w1704, w1703) -> (w1701:bool)
                    n898 = Concatenate Strings(w1689, " connected as ACQ" ("String in")) -> (w1693:string)
                    n899 = Select(t=w1702, s=w1701, f=T33."Disabled and Grayed Out" ("Disabled")) -> (s? t:f=w1697:T33)
                    n900 = property class="Clust (strict)"(reference=w1707, "DisabledEnum"=w1702) -> ()  [unwired: 1 in, 2 out]
                    n901 = local read "loggersRef"() -> (w1700:refnum<file>)
                    n902 = control-ref of="Run FDMR+ btn"() -> (w1699:refnum<vi>)
                    n903 = call "Add actual date time to string.vi"("String in"=w1693) -> ("String out"=w1692:string)  [unwired: 4 in]
                    n904 = Build Array(w1699) -> (w1698:refnum<vi>[])
                    n905 = call "Write in logger.vi"("String in"=w1692, "logger refnum"=w1700) -> ()  [unwired: 2 in, 2 out]
                    n906 = call "Dis- or en- able controls.vi"("Disabled"=w1697, "Control referencies"=w1698) -> ()  [unwired: 9 in, 1 out]
                    n907 = call "simple Shift string array.vi"("Element in"=w1692, "Array in"=w1696) -> ("Array out"=w1695:string[])  [unwired: 8 in, 1 out]
                  }
                  frame "Set parameters" {
                    n908 = Variant To Data(type=T15 {"Filter order"=1.0, "Filter tau [ms]"=1.0, "F_Mod [kHz]"=0.0, "Amp_Mod [mV]"=0.0, "Enable output"=0, "Phase [°]"=0.0} ("ACQ parameters"), Variant=w1727) -> (data=w1712:T15)  [unwired: 1 in, 1 out]
                    n909 = local read "Acquisition controls"() -> (w1713:T14)
                    n910 = Unbundle By Name(w1712) -> ("F_Mod [kHz]"=w1718:dbl, "Amp_Mod [mV]"=w1717:dbl, "Enable output"=w1716:u16)
                    n911 = property on="ACQ parameters" class="Clust (strict)"("Value"=w1712) -> ()  [unwired: 2 in, 2 out]
                    n912 = Bundle By Name(cluster=w1713, "ACQ parameters"=w1712) -> (w1725:T14)
                    n913 = Greater Or Equal To 0?(x=w1716) -> (x >= 0?=w1715:bool)
                    n914 = local write "Acquisition controls"(w1725) -> ()
                    n915 = call "Add actual date time to string.vi"("String in"="Lock-in: parameters set" ("Element in")) -> ("String out"=w1721:string)  [unwired: 4 in]
                    n916 = call "simple Shift string array.vi"("Element in"=w1721, "Array in"=w1724) -> ("Array out"=w1723:string[])  [unwired: 8 in, 1 out]
                    n917 = Bundle By Name(cluster=w1720, "Last update"=w1719, "Freq [kHz]"=w1718, "Ampl [mV]"=w1717, "OutEn"=w1715) -> (w1714:T83)
                  }
                  frame "Update" {
                    w1739 = 1000.0 ("x")
                    n918 = Variant To Data(type=T60 {"In50"=FALSE, "InAC"=FALSE, "InDiff"=FALSE, "Out50"=FALSE, "OutEN"=FALSE, "OutF[Hz]"=0.0, "OutA[V]"=0.0, "DemEN"=FALSE, "Const[ms]"=0.0, "Order[-]"=0, "Phase [°]"=0.0} ("Lock-in info"), Variant=w1748) -> (data=w1744:T60)  [unwired: 1 in, 1 out]
                    n919 = Unbundle By Name(w1744) -> ("OutF[Hz]"=w1741:dbl, "OutA[V]"=w1740:dbl, "OutEN"=w1735:bool, "Out50"=w1732:bool, "In50"=w1729:bool, "Order[-]"=w1731:i32, "Const[ms]"=w1730:dbl, "DemEN"=w1728:bool)
                    n920 = Divide(x=w1741, y=w1739) -> (x/y=w1734:dbl)
                    n921 = Multiply(x=w1740, y=w1739) -> (x*y=w1733:dbl)
                    n922 = Boolean To (0,1)(Boolean=w1735) -> (0, 1=w1736:i16)
                    n923 = local read "Acquisition controls"() -> (w1738:T14)
                    n924 = Bundle By Name(cluster=w1738, "ACQ parameters.Enable output"=w1736, "ACQ parameters.F_Mod [kHz]"=w1734, "ACQ parameters.Amp_Mod [mV]"=w1733, "Out50"=w1732, "In50"=w1729, "ACQ parameters.Filter order"=w1731, "ACQ parameters.Filter tau [ms]"=w1730, "DemEn"=w1728) -> (w1737:T14)
                    n925 = Bundle By Name(cluster=w1745, "Last update"=w1742, "Freq [kHz]"=w1734, "Ampl [mV]"=w1733, "OutEn"=w1735, "In50 Ohm"=w1729, "DemEn"=w1728) -> (w1743:T83)
                    n926 = local write "Acquisition controls"(w1737) -> ()
                  }
                  frame "Get point" {
                    n927 = local read "Acquisition controls"() -> (w1759:T14)
                    n928 = local read "Tab Control"() -> (w1762:T6)
                    n929 = Unbundle By Name(w1759) -> ("ACQ shot btn"=w1758:bool)
                    n930 = Variant To Data(type=T62 {"Timestamps (ticks)"=0, "X (Vrms)"=0.0, "Y (Vrms)"=0.0, "Osc Phase (deg)"=0.0, "Freq (Hz)"=0.0, "DIO"=0, "AuxIn0 (V)"=0.0, "AuxIn1 (V)"=0.0, "Trigger"=0} ("Update data"), Variant=w1767) -> (data=w1765:T62)  [unwired: 1 in, 1 out]
                    n931 = Unbundle By Name(w1765) -> ("X (Vrms)"=w1752:dbl, "Y (Vrms)"=w1751:dbl)  [unwired: 2 out]
                    n932 = Equal?(x=w1762, y=T61."Adjustment" ("Tab Control")) -> (x = y?=w1761:bool)
                    n933 = And(x=w1761, y=w1758) -> (x .and. y?=w1760:bool)
                    n934 = case shown="False" w1760 {
                      tunnel: w1752 -> [_ w1770]
                      tunnel: w1751 -> [_ w1769]
                      frame False {
                      }
                      frame True {
                        n935 = Bundle("X (Vrms)"=w1770, "Y (Vrms)"=w1769) -> (→"lookup":cluster{"X (Vrms)":dbl, "Y (Vrms)":dbl})  [unwired: 1 in]
                      }
                    }
                    n936 = Build Array(w1752) -> (w1750:dbl[])
                    n937 = Build Array(w1751) -> (w1749:dbl[])
                    n938 = Bundle By Name(cluster=T2 {"X"=[], "Y"=[]} ("Lock-in data"), "X"=w1750, "Y"=w1749) -> (w1753:T2)
                    n939 = local write "Lock-in data"(w1753) -> ()
                    "New data" <- TRUE ("New data")
                    "data time" <- w1764
                  }
                  frame "Get array" {
                    # "change this"
                    n940 = local write "data time"(w1775) -> ()
                    n941 = local write "New data"(TRUE ("New data")) -> ()
                    n942 = Variant To Data(type=T2 {"X"=[], "Y"=[]} ("ADQ data"), Variant=w1776) -> (data=→"Lock-in data":T2)  [unwired: 1 in, 1 out]
                  }
                  frame "Get ModA" {
                    n943 = Variant To Data(type=0.0, Variant=w1794) -> (data=w1790:dbl)  [unwired: 1 in, 1 out]
                    n944 = local read "Acquisition controls"() -> (w1786:T14)
                    n945 = Unbundle By Name(w1786) -> ("Desired [G]"=w1785:dbl, "ACQ parameters.Amp_Mod [mV]"=w1784:dbl, "Auto-modulation"=w1781:bool, "ACQ parameters.Enable output"=w1780:u16, "Sample holder"=w1782:T16)
                    n946 = call "Modulation current to field conversion.vi"("Sample holder"=w1782, "Modulation current (mA)"=w1790) -> ("Modulation field (G)"=w1783:dbl)  [unwired: 9 in]
                    n947 = Greater Than 0?(x=w1780) -> (x > 0?=w1778:bool)
                    n948 = And(x=w1781, y=w1778) -> (x .and. y?=w1779:bool)
                    n949 = Unbundle By Name(w1788) -> ("Data_Aq"=w1787:refnum<queue>)
                    n950 = call "Modulation amplitude auto adjustment.vi"("Amp_Mod [mV]"=w1784, "Enable auto adjustment"=w1779, "Actual [G]"=w1783, "Desired [G]"=w1785, "Queue in"=w1787) -> ("Adjusted"=w1789:bool)  [unwired: 6 in]
                    n951 = Bundle By Name(cluster=w1786, "Modulation [A]"=w1790, "Actual [G]"=w1783, "Adj mod"=w1789) -> (w1792:T14)
                    n952 = local write "Acquisition controls"(w1792) -> ()
                  }
                  frame "End" {
                    n953 = Variant To Data(type=T63 {"handleValid"=FALSE, "Conn"=0, "Path Prefix"="", "Handle"=0, "Connected"=FALSE, "Clockbase(s)"=0.0} ("Handle Out"), Variant=w1804) -> ()  [unwired: 1 in, 2 out]
                    n954 = local read "loggersRef"() -> (w1801:refnum<file>)
                    n955 = property on="MFLI" class="Bool (strict)"("Value"=FALSE) -> ()  [unwired: 2 in, 2 out]
                    n956 = call "Add actual date time to string.vi"("String in"="ACQ disconnected") -> ("String out"=w1797:string)  [unwired: 4 in]
                    n957 = call "Write in logger.vi"("String in"=w1797, "logger refnum"=w1801) -> ()  [unwired: 2 in, 2 out]
                    n958 = call "simple Shift string array.vi"("Element in"=w1797, "Array in"=w1799) -> ("Array out"=w1798:string[])  [unwired: 8 in, 1 out]
                  }
                  frame "Ignore", Default {
                  }
                }
                n959 = Bundle By Name(cluster=w1677, "MFLI"=w1679) -> (w1678:T8)
              }
              frame "SMU2450" {
                n960 = Unbundle By Name(w1811) -> ("SMU"=w1810:T84)
                n961 = case shown="\"Get actual results\"" w1814 {
                  tunnel: w1812 -> [w1820 w1841 w1844 w1865 w1878 w1912 w1931]
                  tunnel: [w1820 w1840 w1844 w1866 w1878 w1913 w1932] -> w1813
                  tunnel: w1815 -> [_ w1836 _ w1864 w1895 w1914 w1933]
                  tunnel: w1809 -> [_ w1826 _ w1860 w1892 w1915 w1934]
                  tunnel: w1816 -> [w1819 w1835 w1843 w1859 w1891 w1919 w1938]
                  tunnel: [w1819 w1835 w1843 w1859 w1891 w1919 w1938] -> w1817
                  tunnel: w1810 -> [w1818 w1833 w1842 w1862 w1894 w1918 w1937]
                  tunnel: [w1818 w1832 w1842 w1861 w1893 w1917 w1936] -> w1807
                  frame "Ignore", Default {
                  }
                  frame "Connect" {
                    n962 = Variant To Data(type=T64 {"VISA name"="", "Connected"=FALSE, "Name"="", "Message"="", "Error message"="", "Min voltage"=0.0, "Max voltage"=0.0, "Min Current"=0.0, "Max Current"=0.0, "Measurement value"=0.0, "Source Voltage"=0.0, "Measurement"=FALSE, "Source Current"=0.0, "Source Mode"=0, "Measure Function"=0} ("output cluster"), Variant=w1836) -> (data=w1828:T64, error out=w1829:errorcluster)  [unwired: 1 in]
                    n963 = Unbundle By Name(w1828) -> ("Name"=w1821:string, "Message"=w1823:string, "Connected"=w1827:bool)  [unwired: 1 out]
                    n964 = local read "Instr status"() -> (w1838:T1)
                    n965 = Bundle By Name(cluster=w1838, "SMU"=w1827) -> (w1839:T1)
                    n966 = local write "Instr status"(w1839) -> ()
                    n967 = Concatenate Strings(w1821, " connected. " ("string"), w1823) -> (w1822:string)
                    n968 = Bundle By Name(cluster=w1833, "Name"=w1821, "Last update"=w1826) -> (w1832:T84)
                    n969 = property on="SMU controls" class="Clust (strict)"("DisabledEnum"=T33."Enabled" ("Disabled")) -> ()  [unwired: 2 in, 2 out]
                    n970 = local read "loggersRef"() -> (w1837:refnum<file>)
                    n971 = call "Add actual date time to string.vi"("String in"=w1822) -> ("String out"=w1825:string)  [unwired: 4 in]
                    n972 = call "Write in logger.vi"("error in"=w1829, "String in"=w1825, "logger refnum"=w1837) -> ("error out"=w1834:errorcluster)  [unwired: 1 in, 1 out]
                    n973 = call "simple Shift string array.vi"("Element in"=w1825, "Array in"=w1841) -> ("Array out"=w1840:string[])  [unwired: 8 in, 1 out]
                    n974 = call <vilib>:"Clear Errors.vi"("error in (no error)"=w1834) -> ()  [unwired: 5 in, 2 out]
                  }
                  frame "Update" {
                  }
                  frame "Set measurement" {
                    # "add surce funcion and value"
                    n975 = Variant To Data(type=T64 {"VISA name"="", "Connected"=FALSE, "Name"="", "Message"="", "Error message"="", "Min voltage"=0.0, "Max voltage"=0.0, "Min Current"=0.0, "Max Current"=0.0, "Measurement value"=0.0, "Source Voltage"=0.0, "Measurement"=FALSE, "Source Current"=0.0, "Source Mode"=0, "Measure Function"=0} ("SMU status out"), Variant=w1864) -> (data=w1858:T64)  [unwired: 1 in, 1 out]
                    n976 = Unbundle By Name(w1858) -> ("Measurement value"=w1846:dbl, "Measurement"=w1856:bool, "Source Voltage"=w1854:dbl, "Source Current"=w1855:dbl, "Source Mode"=w1848:u16, "Measure Function"=w1852:u16)
                    n977 = case shown="0, Default" w1848 {
                      tunnel: w1855 -> [_ w1872]
                      tunnel: w1854 -> [w1870 _]
                      tunnel: [w1870 w1872] -> w1847
                      tunnel: ["Voltage" "Current"] -> w1853
                      frame 0, Default {
                      }
                      frame 1 {
                      }
                    }
                    n978 = case shown="0, Default" w1852 {
                      tunnel: ["Voltage" "Current"] -> w1851
                      frame 0, Default {
                      }
                      frame 1 {
                      }
                    }
                    n979 = local read "SMU controls"() -> (w1850:T21)
                    n980 = Bundle By Name(cluster=w1850, "Measurement settings.Source Mode"=w1848, "Measurement settings.Source Level"=w1847, "Value"=w1846) -> (w1849:T21)
                    n981 = Bundle By Name(cluster=w1862, "Last update"=w1860, "MeasValue"=w1846, "Output"=w1856, "SourFunc"=w1853, "SourValue"=w1847, "MeasFunc"=w1851) -> (w1861:T84)
                    n982 = local write "SMU controls"(w1849) -> ()
                    n983 = call "Add actual date time to string.vi"("String in"="SMU set") -> ("String out"=w1863:string)  [unwired: 4 in]
                    n984 = call "simple Shift string array.vi"("Element in"=w1863, "Array in"=w1865) -> ("Array out"=w1866:string[])  [unwired: 8 in, 1 out]
                  }
                  frame "Get actual results" {
                    # "add surce funcion and value"
                    n985 = Variant To Data(type=T64 {"VISA name"="", "Connected"=FALSE, "Name"="", "Message"="", "Error message"="", "Min voltage"=0.0, "Max voltage"=0.0, "Min Current"=0.0, "Max Current"=0.0, "Measurement value"=0.0, "Source Voltage"=0.0, "Measurement"=FALSE, "Source Current"=0.0, "Source Mode"=0, "Measure Function"=0} ("SMU status out"), Variant=w1895) -> (data=w1890:T64)  [unwired: 1 in, 1 out]
                    n986 = Unbundle By Name(w1890) -> ("Measurement value"=w1876:dbl, "Measurement"=w1888:bool, "Source Voltage"=w1886:dbl, "Source Current"=w1887:dbl, "Source Mode"=w1880:u16, "Measure Function"=w1879:u16)
                    n987 = Add(x=w1876, y=3.7e-06) -> (x+y=w1874:dbl)
                    n988 = case shown="1" w1880 {
                      tunnel: w1887 -> [_ w1901]
                      tunnel: w1886 -> [w1899 _]
                      tunnel: [w1899 w1901] -> w1885
                      tunnel: ["Voltage" "Current"] -> w1884
                      frame 0, Default {
                      }
                      frame 1 {
                      }
                    }
                    n989 = case shown="0, Default" w1879 {
                      tunnel: ["Voltage" "Current"] -> w1883
                      frame 0, Default {
                      }
                      frame 1 {
                      }
                    }
                    n990 = Divide(x=w1874, y=0.00998) -> (x/y=w1877:dbl)
                    n991 = local read "SMU controls"() -> (w1882:T21)
                    n992 = Bundle By Name(cluster=w1882, "Value"=w1874, "B[T]"=w1877) -> (w1881:T21)
                    n993 = Bundle By Name(cluster=w1894, "Last update"=w1892, "MeasValue"=w1876, "Output"=w1888, "SourFunc"=w1884, "SourValue"=w1885, "MeasFunc"=w1883) -> (w1893:T84)
                    n994 = local write "SMU controls"(w1881) -> ()
                  }
                  frame "End" {
                    n995 = Variant To Data(type=T64 {"VISA name"="", "Connected"=FALSE, "Name"="", "Message"="", "Error message"="", "Min voltage"=0.0, "Max voltage"=0.0, "Min Current"=0.0, "Max Current"=0.0, "Measurement value"=0.0, "Source Voltage"=0.0, "Measurement"=FALSE, "Source Current"=0.0, "Source Mode"=0, "Measure Function"=0} ("SMU status out"), Variant=w1914) -> (data=w1907:T64)  [unwired: 1 in, 1 out]
                    n996 = Unbundle By Name(w1907) -> ("Name"=w1905:string, "Measurement"=w1903:bool)
                    n997 = Bundle By Name(cluster=w1918, "Name"="None" ("Master"), "Output"=w1903, "Last update"=w1915) -> (w1917:T84)
                    n998 = property on="SMU" class="Bool (strict)"("Value"=FALSE) -> ()  [unwired: 2 in, 2 out]
                    n999 = Concatenate Strings("SMU module " ("String in"), w1905, " ended." ("string")) -> (w1906:string)
                    n1000 = call "Add actual date time to string.vi"("String in"=w1906) -> ("String out"=w1911:string)  [unwired: 4 in]
                    n1001 = Concatenate Strings(w1911, "\r\n") -> (w1910:string)
                    n1002 = local read "loggersRef"() -> (w1921:refnum<file>)
                    n1003 = call "Write in logger.vi"("String in"=w1910, "logger refnum"=w1921) -> ()  [unwired: 2 in, 2 out]
                    n1004 = call "simple Shift string array.vi"("Element in"=w1910, "Array in"=w1912) -> ("Array out"=w1913:string[])  [unwired: 8 in, 1 out]
                  }
                  frame "Disconnect" {
                    n1005 = Variant To Data(type=T64 {"VISA name"="", "Connected"=FALSE, "Name"="", "Message"="", "Error message"="", "Min voltage"=0.0, "Max voltage"=0.0, "Min Current"=0.0, "Max Current"=0.0, "Measurement value"=0.0, "Source Voltage"=0.0, "Measurement"=FALSE, "Source Current"=0.0, "Source Mode"=0, "Measure Function"=0} ("SMU status out"), Variant=w1933) -> (data=w1928:T64)  [unwired: 1 in, 1 out]
                    n1006 = Unbundle By Name(w1928) -> ("Name"=w1924:string, "Measurement"=w1923:bool)
                    n1007 = Bundle By Name(cluster=w1937, "Name"="None" ("Master"), "Output"=w1923, "Last update"=w1934) -> (w1936:T84)
                    n1008 = property on="SMU" class="Bool (strict)"("Value"=FALSE) -> ()  [unwired: 2 in, 2 out]
                    n1009 = Concatenate Strings(w1924, " SMU disconnected." ("String in")) -> (w1925:string)
                    n1010 = call "Add actual date time to string.vi"("String in"=w1925) -> ("String out"=w1930:string)  [unwired: 4 in]
                    n1011 = Concatenate Strings(w1930, "\r\n") -> (w1929:string)
                    n1012 = local read "loggersRef"() -> (w1940:refnum<file>)
                    n1013 = call "Write in logger.vi"("String in"=w1929, "logger refnum"=w1940) -> ()  [unwired: 2 in, 2 out]
                    n1014 = call "simple Shift string array.vi"("Element in"=w1929, "Array in"=w1931) -> ("Array out"=w1932:string[])  [unwired: 8 in, 1 out]
                  }
                }
                n1015 = Bundle By Name(cluster=w1811, "SMU"=w1807) -> (w1808:T8)
              }
              frame "VTI" {
                n1016 = Unbundle By Name(w1946) -> ("VTI"=w1944:T85)
                n1017 = case shown="\"Set point\"" w1951 {
                  tunnel: w1950 -> [_ w1971 w1991 w2007 _]
                  tunnel: w1949 -> [w1954 w1969 w1989 w2003 w2040]
                  tunnel: [w1954 w1968 w1989 w2002 w2039] -> w1948
                  tunnel: w1941 -> [w1953 w1959 w1987 w2005 w2035]
                  tunnel: [w1953 w1959 w1986 w2005 w2035] -> w1947
                  tunnel: w1944 -> [w1952 w1958 w1985 w2004 w2034]
                  tunnel: w1943 -> [_ _ w1974 _ _]
                  tunnel: [w1952 w1957 w1984 w2004 w2033] -> w1942
                  frame "Ignore", Default {
                  }
                  frame "Initialize" {
                    n1018 = Variant To Data(type="", Variant=w1971) -> (data=w1956:string)  [unwired: 1 in, 1 out]
                    n1019 = local read "Instr status"() -> (w1965:T1)
                    n1020 = Bundle By Name(cluster=w1965, "VTI"=TRUE) -> (w1964:T1)
                    n1021 = local write "Instr status"(w1964) -> ()
                    n1022 = Concatenate Strings("Temperature controller " ("string"), w1956, " initialized" ("string")) -> (w1960:string)
                    n1023 = local read "loggersRef"() -> (w1961:refnum<file>)
                    n1024 = call "Add actual date time to string.vi"("String in"=w1960) -> ("String out"=w1962:string)  [unwired: 4 in]
                    n1025 = call "Write in logger.vi"("String in"=w1962, "logger refnum"=w1961) -> ()  [unwired: 2 in, 2 out]
                    n1026 = property on="VTI control" class="Clust (strict)"("DisabledEnum"=T33."Enabled" ("Disabled")) -> ()  [unwired: 2 in, 2 out]
                    n1027 = Bundle By Name(cluster=w1958, "TempCtl"=w1956) -> (w1957:T85)
                    n1028 = call "simple Shift string array.vi"("Element in"=w1960, "Array in"=w1969) -> ("Array out"=w1968:string[])  [unwired: 8 in, 1 out]
                  }
                  frame "Update" {
                    n1029 = Variant To Data(type=T65 {"VTI space"=0.0, "Sample"=0.0, "He pot"=0.0, "Trap"=0.0, "Ambient"=0.0, "SetP_VTI"=0.0, "SetP_Smp"=0.0, "SetP_Pot"=0.0, "SetP_Trap"=0.0, "Range out 1"=1, "Out 1 [%]"=0.0, "Out 2 [%]"=0.0} ("TC sensors [K]"), Variant=w1991) -> (data=w1988:T65)  [unwired: 1 in, 1 out]
                    n1030 = Unbundle By Name(w1988) -> ("Ambient"=w1973:dbl, "VTI space"=w1972:dbl, "Sample"=w1983:dbl, "Trap"=w1982:dbl, "He pot"=w1981:dbl, "SetP_VTI"=w1978:dbl, "SetP_Smp"=w1977:dbl, "SetP_Pot"=w1976:dbl, "SetP_Trap"=w1975:dbl)
                    n1031 = local read "VTI control"() -> (w1980:T13)
                    n1032 = Bundle By Name(cluster=w1985, "Last update"=w1974, "Ambient [K]"=w1973, "VTI [K]"=w1972, "Sample [K]"=w1983, "Trap[K]"=w1982, "HePot [K]"=w1981) -> (w1984:T85)
                    n1033 = Bundle By Name(cluster=w1980, "VTI space [K]"=w1978, "Sample [K]"=w1977, "Heater3 [K]"=w1976, "Heater4 [K]"=w1975) -> (w1979:T13)
                    n1034 = Bundle By Name(cluster=w1987, "T_sample [K]"=w1972) -> (w1986:T27)
                    n1035 = local write "VTI control"(w1979) -> ()
                  }
                  frame "Set point" {
                    n1036 = Variant To Data(type=T51 {"Heater"="", "Tmp [K]"=0.0}, Variant=w2007) -> (data=w2006:T51)  [unwired: 1 in, 1 out]
                    n1037 = Unbundle By Name(w2006) -> ("Heater"=w1996:string, "Tmp [K]"=w1993:dbl)
                    n1038 = local read "VTI control"() -> (w1995:T13)
                    n1039 = case shown="\"Heater3 [K]\"" w1996 {
                      selector: w1996 -> [_ w2011 w2016 w2024 w2029]
                      tunnel: [u16 0 ("Output's Control Loop (1:1)") w2015 w2020 w2025 w2030] -> _
                      tunnel: w1993 -> [_ w2012 w2017 w2021 w2026]
                      tunnel: w1995 -> [w2009 w2014 w2019 w2023 w2028]
                      tunnel: [w2009 w2013 w2018 w2022 w2027] -> w1994
                      tunnel: ["Unknown setpoint" w2011 w2016 w2024 w2029] -> w1992
                      frame "None", Default {
                      }
                      frame "VTI space [K]" {
                        w2015 = u16 1 items=["1"=1, "2"=2, "3"=3, "4"=4] ("Output's Control Loop (1:1)")
                        n1040 = Bundle By Name(cluster=w2014, "VTI space [K]"=w2012) -> (w2013:T13)
                      }
                      frame "Sample [K]" {
                        w2020 = u16 2 items=["1"=1, "2"=2, "3"=3, "4"=4] ("Output's Control Loop (1:1)")
                        n1041 = Bundle By Name(cluster=w2019, "Sample [K]"=w2017) -> (w2018:T13)
                      }
                      frame "Heater3 [K]" {
                        w2025 = u16 3 items=["1"=1, "2"=2, "3"=3, "4"=4] ("Output's Control Loop (1:1)")
                        n1042 = Bundle By Name(cluster=w2023, "Heater3 [K]"=w2021) -> (w2022:T13)
                      }
                      frame "Heater4 [K]" {
                        w2030 = u16 4 items=["1"=1, "2"=2, "3"=3, "4"=4] ("Output's Control Loop (1:1)")
                        n1043 = Bundle By Name(cluster=w2028, "Heater4 [K]"=w2026) -> (w2027:T13)
                      }
                    }
                    n1044 = local write "VTI control"(w1994) -> ()
                    n1045 = Format Into String(format string="%f K", initial string=w1992, w1993) -> (resulting string=w2000:string)  [unwired: 1 in, 1 out]
                    n1046 = local read "loggersRef"() -> (w2001:refnum<file>)
                    n1047 = call "Add actual date time to string.vi"("String in"=w2000) -> ("String out"=w1998:string)  [unwired: 4 in]
                    n1048 = call "simple Shift string array.vi"("Element in"=w1998, "Array in"=w2003) -> ("Array out"=w2002:string[])  [unwired: 8 in, 1 out]
                    n1049 = call "Write in logger.vi"("String in"=w1998, "logger refnum"=w2001) -> ()  [unwired: 2 in, 2 out]
                  }
                  frame "End" {
                    w2037 = "VTI closed" ("Element in")
                    n1050 = local read "Instr status"() -> (w2043:T1)
                    n1051 = Bundle By Name(cluster=w2034, "TempCtl"="None" ("TC")) -> (w2033:T85)
                    n1052 = Bundle By Name(cluster=w2043, "VTI"=FALSE) -> (w2041:T1)
                    n1053 = local write "Instr status"(w2041) -> ()
                    n1054 = property on="VTI control" class="Clust (strict)"("DisabledEnum"=T33."Disabled and Grayed Out" ("Disabled")) -> ()  [unwired: 2 in, 2 out]
                    n1055 = call "Add actual date time to string.vi"("String in"=w2037) -> ("String out"=w2036:string)  [unwired: 4 in]
                    n1056 = local read "loggersRef"() -> (w2038:refnum<file>)
                    n1057 = call "simple Shift string array.vi"("Element in"=w2037, "Array in"=w2040) -> ("Array out"=w2039:string[])  [unwired: 8 in, 1 out]
                    n1058 = call "Write in logger.vi"("String in"=w2036, "logger refnum"=w2038) -> ()  [unwired: 2 in, 2 out]
                  }
                }
                n1059 = call "simple Shift string array.vi"() -> ()  [unwired: 10 in, 2 out]
                n1060 = Bundle By Name(cluster=w1946, "VTI"=w1942) -> (w1945:T8)
              }
              frame "Servo" {
                n1061 = Unbundle By Name(w2048) -> ("Servo"=w2046:T10[])
                n1062 = case shown="\"Update\"" w2050 {
                  selector: w2050 -> [w2070 w2118 w2171 _ w2244]
                  tunnel: w2053 -> [w2072 w2120 w2178 _ w2242]
                  tunnel: w2052 -> [w2068 w2116 w2174 w2229 w2247]
                  tunnel: [w2069 w2117 w2175 w2230 w2246] -> w2051
                  tunnel: w2046 -> [w2055 w2104 w2157 w2225 w2236]
                  tunnel: [w2054 w2106 w2156 w2224 w2236] -> w2045
                  tunnel: w2044 -> [w2056 _ w2154 _ _]
                  frame "Initialize" {
                    n1063 = Variant To Data(type=T66[] [] ("Servo status"), Variant=w2072) -> (data=w2058:T66[])  [unwired: 1 in, 1 out]
                    n1064 = Index Array(array=w2055) -> (element=w2057:T10)  [unwired: 1 in]
                    n1065 = for {
                      tunnel: w2058 -> [w2088] mode=indexing
                      tunnel: w2057 -> [w2084]
                      tunnel: w2056 -> [w2082]
                      tunnel: [w2076] -> w2054 mode=indexing
                      n1066 = Unbundle By Name(w2088) -> ("Servo constants.Name"=w2083:T11, "Servo variables.Actual position"=w2081:dbl, "Servo constants.Pos position limit [mm]"=w2078:dbl, "Servo constants.Neg position limit [mm]"=w2077:dbl, "Servo variables.Power ON"=w2079:bool, "Servo variables.Connected"=w2080:bool)
                      n1067 = Select(t=T33."Enabled" ("Disabled"), s=w2080, f=T33."Disabled and Grayed Out" ("Disabled")) -> (s? t:f=w2085:T33)
                      n1068 = Bundle By Name(cluster=w2084, "Name"=w2083, "Last update"=w2082, "Position"=w2081, "Pos limit"=w2078, "Neg limit"=w2077, "Power"=w2079) -> (w2076:T10)
                      n1069 = case shown="\"AxisX\", Default" w2083 {
                        tunnel: w2081 -> [w2090 w2092 w2094 w2096 w2098]
                        tunnel: w2080 -> [_ _ _ _ _]
                        tunnel: w2085 -> [w2089 w2091 w2093 w2095 w2097]
                        frame "AxisX", Default {
                          n1070 = property on="X backward" class="Bool (strict)"("DisabledEnum"=w2089) -> ()  [unwired: 2 in, 2 out]
                          n1071 = property on="X forward" class="Bool (strict)"("DisabledEnum"=w2089) -> ()  [unwired: 2 in, 2 out]
                          n1072 = property on="X" class="DigNum (strict)"("Value"=w2090) -> ()  [unwired: 2 in, 2 out]
                        }
                        frame "AxisY" {
                          n1073 = property on="Y left" class="Bool (strict)"("DisabledEnum"=w2091) -> ()  [unwired: 2 in, 2 out]
                          n1074 = property on="Y right" class="Bool (strict)"("DisabledEnum"=w2091) -> ()  [unwired: 2 in, 2 out]
                          n1075 = property on="Y" class="DigNum (strict)"("Value"=w2092) -> ()  [unwired: 2 in, 2 out]
                        }
                        frame "AxisZ_left" {
                          n1076 = property on="ZLup" class="Bool (strict)"("DisabledEnum"=w2093) -> ()  [unwired: 2 in, 2 out]
                          n1077 = property on="ZLdown" class="Bool (strict)"("DisabledEnum"=w2093) -> ()  [unwired: 2 in, 2 out]
                          n1078 = property on="ZL" class="DigNum (strict)"("Value"=w2094) -> ()  [unwired: 2 in, 2 out]
                        }
                        frame "AxisZ_middle" {
                          n1079 = property on="ZM" class="DigNum (strict)"("Value"=w2096) -> ()  [unwired: 2 in, 2 out]
                          n1080 = property on="ZMdown" class="Bool (strict)"("DisabledEnum"=w2095) -> ()  [unwired: 2 in, 2 out]
                          n1081 = property on="ZMup" class="Bool (strict)"("DisabledEnum"=w2095) -> ()  [unwired: 2 in, 2 out]
                        }
                        frame "AxisZ_right" {
                          n1082 = property on="ZRup" class="Bool (strict)"("DisabledEnum"=w2097) -> ()  [unwired: 2 in, 2 out]
                          n1083 = property on="ZRdown" class="Bool (strict)"("DisabledEnum"=w2097) -> ()  [unwired: 2 in, 2 out]
                          n1084 = property on="ZR" class="DigNum (strict)"("Value"=w2098) -> ()  [unwired: 2 in, 2 out]
                        }
                      }
                    }
                    n1085 = for {
                      tunnel: w2058 -> [w2100] mode=indexing
                      tunnel: [w2099] -> w2062 mode=indexing
                      n1086 = Unbundle By Name(w2100) -> ("Servo variables.Connected"=w2099:bool)
                    }
                    n1087 = And Array Elements(Boolean array=w2062) -> (logical AND=w2061:bool)
                    n1088 = call <vilib>:"Space Constant.vi"() -> ("String"=w2064:string)
                    n1089 = case shown="True" w2061 {
                      frame False {
                      }
                      frame True {
                        n1090 = control-ref of="Servo controls"() -> (w2075:refnum<vi>)
                        n1091 = Build Array(w2075) -> (w2074:refnum<vi>[])
                        n1092 = call "Dis- or en- able controls.vi"("Disabled"=T33."Enabled", "Control referencies"=w2074) -> ()  [unwired: 9 in, 1 out]
                      }
                    }
                    n1093 = local read "Instr status"() -> (w2067:T1)
                    n1094 = Concatenate Strings("Servo" ("string"), w2064, w2070, w2064) -> (w2071:string)
                    n1095 = local read "loggersRef"() -> (w2060:refnum<file>)
                    n1096 = Bundle By Name(cluster=w2067, "Serv"=w2061) -> (w2066:T1)
                    n1097 = call "Add actual date time to string.vi"("String in"=w2071) -> ("String out"=w2059:string)  [unwired: 4 in]
                    n1098 = local write "Instr status"(w2066) -> ()
                    n1099 = call "simple Shift string array.vi"("Element in"=w2059, "Array in"=w2068) -> ("Array out"=w2069:string[])  [unwired: 8 in, 1 out]
                    n1100 = call "Write in logger.vi"("String in"=w2059, "logger refnum"=w2060) -> ()  [unwired: 2 in, 2 out]
                  }
                  frame "Move by" {
                    n1101 = Variant To Data(type=T69 {"Property"="", "Value"=variant, "Name"=enum."AxisX"} ("Array"), Variant=w2120) -> (data=w2112:T69)  [unwired: 1 in, 1 out]
                    n1102 = Unbundle By Name(w2112) -> ("Property"=w2111:string, "Value"=w2110:variant, "Name"=w2109:T11)
                    n1103 = call "Extract axis properties.vi"("Name"=w2109, "All servo status"=w2104) -> ("Servo"=w2103:T10, "Index"=w2105:i32, "Found?"=w2107:bool)  [unwired: 6 in]
                    n1104 = case shown="True" w2107 {
                      tunnel: w2111 -> [w2122 w2131]
                      tunnel: w2110 -> [_ w2130]
                      tunnel: w2109 -> [_ w2129]
                      tunnel: w2103 -> [_ w2128]
                      tunnel: w2105 -> [_ w2127]
                      tunnel: w2104 -> [w2121 w2126]
                      tunnel: [w2122 w2124] -> w2108
                      tunnel: [w2121 w2123] -> w2106
                      frame False {
                      }
                      frame True {
                        n1105 = case shown="\"Power ON\"" w2131 {
                          selector: w2131 -> [w2132 w2135 w2147]
                          tunnel: w2130 -> [_ w2134 w2153]
                          tunnel: w2129 -> [_ w2137 _]
                          tunnel: w2128 -> [w2133 w2140 w2151]
                          tunnel: [w2133 w2139 w2150] -> w2125
                          tunnel: [w2132 w2138 w2149] -> w2124
                          frame "Nothing", Default {
                          }
                          frame "Actual position" {
                            n1106 = Variant To Data(type=0.0, Variant=w2134) -> (data=w2136:dbl)  [unwired: 1 in, 1 out]
                            n1107 = case shown="\"AxisZ_right\"" w2137 {
                              tunnel: w2136 -> [w2142 w2143 w2144 w2145 w2146]
                              frame "AxisX", Default {
                                n1108 = property on="X" class="DigNum (strict)"("Val(Sgnl)"=w2142) -> ()  [unwired: 2 in, 2 out]
                              }
                              frame "AxisY" {
                                n1109 = property on="Y" class="DigNum (strict)"("Value"=w2143) -> ()  [unwired: 2 in, 2 out]
                              }
                              frame "AxisZ_left" {
                                n1110 = property on="ZL" class="DigNum (strict)"("Value"=w2144) -> ()  [unwired: 2 in, 2 out]
                              }
                              frame "AxisZ_middle" {
                                n1111 = property on="ZM" class="DigNum (strict)"("Value"=w2145) -> ()  [unwired: 2 in, 2 out]
                              }
                              frame "AxisZ_right" {
                                n1112 = property on="ZR" class="DigNum (strict)"("Value"=w2146) -> ()  [unwired: 2 in, 2 out]
                              }
                            }
                            n1113 = Bundle By Name(cluster=w2140, "Position"=w2136) -> (w2139:T10)
                            n1114 = Format Into String(initial string=w2135, w2136) -> (resulting string=w2138:string)  [unwired: 2 in, 1 out]
                          }
                          frame "Power ON" {
                            n1115 = Variant To Data(type=FALSE ("Connected"), Variant=w2153) -> (data=w2148:bool)  [unwired: 1 in, 1 out]
                            n1116 = Bundle By Name(cluster=w2151, "Power"=w2148) -> (w2150:T10)
                            n1117 = Format Into String(initial string=w2147, w2148) -> (resulting string=w2149:string)  [unwired: 2 in, 1 out]
                          }
                        }
                        n1118 = Replace Array Subset(array=w2126, new element=w2125, index=w2127) -> (w2123:T10[])
                      }
                    }
                    n1119 = call <vilib>:"Space Constant.vi"() -> ("String"=w2114:string)
                    n1120 = local read "loggersRef"() -> (w2101:refnum<file>)
                    n1121 = Concatenate Strings("Servo" ("string"), w2114, w2118, w2114, w2108) -> (w2119:string)
                    n1122 = call "Add actual date time to string.vi"("String in"=w2119) -> ("String out"=w2102:string)  [unwired: 4 in]
                    n1123 = call "Write in logger.vi"("String in"=w2102, "logger refnum"=w2101) -> ()  [unwired: 2 in, 2 out]
                    n1124 = call "simple Shift string array.vi"("Element in"=w2102, "Array in"=w2116) -> ("Array out"=w2117:string[])  [unwired: 8 in, 1 out]
                  }
                  frame "Update" {
                    n1125 = Variant To Data(type=T69 {"Property"="", "Value"=variant, "Name"=enum."AxisX"} ("Array"), Variant=w2178) -> (data=w2170:T69)  [unwired: 1 in, 1 out]
                    n1126 = Unbundle By Name(w2170) -> ("Property"=w2164:string, "Value"=w2169:variant, "Name"=w2166:T11)
                    n1127 = call "Extract axis properties.vi"("Name"=w2166, "All servo status"=w2157) -> ("Servo"=w2168:T10, "Index"=w2167:i32, "Found?"=w2159:bool)  [unwired: 6 in]
                    n1128 = Format Into String(w2166) -> (resulting string=w2165:string)  [unwired: 3 in, 1 out]
                    n1129 = Bundle By Name(cluster=w2168, "Last update"=w2154) -> (w2155:T10)
                    n1130 = call <vilib>:"Space Constant.vi"() -> ("String"=w2161:string)
                    n1131 = Concatenate Strings(w2164, w2161, w2165, ":" ("string"), w2161) -> (w2163:string)
                    n1132 = case shown="False" w2159 {
                      tunnel: w2169 -> [_ w2195]
                      tunnel: w2155 -> [_ w2194]
                      tunnel: w2157 -> [w2179 w2193]
                      tunnel: w2167 -> [_ w2191]
                      tunnel: w2166 -> [w2185 w2190]
                      tunnel: w2164 -> [w2181 w2189]
                      tunnel: w2163 -> [_ w2188]
                      tunnel: [w2183 w2187] -> w2160
                      tunnel: [w2179 w2186] -> w2156
                      frame False {
                        n1133 = call <vilib>:"Space Constant.vi"() -> ("String"=w2180:string)
                        n1134 = Concatenate Strings(w2181, w2180, "Unknown driver" ("initial string")) -> (w2182:string)
                        n1135 = Format Into String(initial string=w2182, w2185) -> (resulting string=w2183:string)  [unwired: 2 in, 1 out]
                      }
                      frame True {
                        n1136 = case shown="\"Target position\"" w2189 {
                          tunnel: w2195 -> [_ w2205 w2216 w2223]
                          tunnel: w2190 -> [_ w2199 _ _]
                          tunnel: w2194 -> [w2197 w2203 w2214 w2221]
                          tunnel: [w2197 w2202 w2214 w2220] -> w2192
                          tunnel: w2188 -> [w2196 w2201 w2211 w2218]
                          tunnel: [w2196 w2200 w2213 w2219] -> w2187
                          frame "Nothing", Default {
                          }
                          frame "Actual position" {
                            n1137 = Variant To Data(type=0.0, Variant=w2205) -> (data=w2198:dbl)  [unwired: 1 in, 1 out]
                            n1138 = case shown="\"AxisZ_left\"" w2199 {
                              tunnel: w2198 -> [w2206 w2207 w2208 w2209 w2210]
                              frame "AxisX", Default {
                                n1139 = property on="X" class="DigNum (strict)"("Val(Sgnl)"=w2206) -> ()  [unwired: 2 in, 2 out]
                              }
                              frame "AxisY" {
                                n1140 = property on="Y" class="DigNum (strict)"("Value"=w2207) -> ()  [unwired: 2 in, 2 out]
                              }
                              frame "AxisZ_left" {
                                n1141 = property on="ZL" class="DigNum (strict)"("Value"=w2208) -> ()  [unwired: 2 in, 2 out]
                              }
                              frame "AxisZ_middle" {
                                n1142 = property on="ZM" class="DigNum (strict)"("Value"=w2209) -> ()  [unwired: 2 in, 2 out]
                              }
                              frame "AxisZ_right" {
                                n1143 = property on="ZR" class="DigNum (strict)"("Value"=w2210) -> ()  [unwired: 2 in, 2 out]
                              }
                            }
                            n1144 = Bundle By Name(cluster=w2203, "Position"=w2198) -> (w2202:T10)
                            n1145 = Format Into String(initial string=w2201, w2198) -> (resulting string=w2200:string)  [unwired: 2 in, 1 out]
                          }
                          frame "Target position" {
                            n1146 = Variant To Data(type=0.0, Variant=w2216) -> (data=w2212:dbl)  [unwired: 1 in, 1 out]
                            n1147 = Format Into String(initial string=w2211, w2212) -> (resulting string=w2213:string)  [unwired: 2 in, 1 out]
                          }
                          frame "Power ON" {
                            n1148 = Variant To Data(type=FALSE ("Connected"), Variant=w2223) -> (data=w2217:bool)  [unwired: 1 in, 1 out]
                            n1149 = Bundle By Name(cluster=w2221, "Power"=w2217) -> (w2220:T10)
                            n1150 = Format Into String(initial string=w2218, w2217) -> (resulting string=w2219:string)  [unwired: 2 in, 1 out]
                          }
                        }
                        n1151 = Replace Array Subset(array=w2193, new element=w2192, index=w2191) -> (w2186:T10[])
                      }
                    }
                    n1152 = call <vilib>:"Space Constant.vi"() -> ("String"=w2158:string)
                    n1153 = Concatenate Strings("Servo" ("string"), w2158, w2171, w2158, w2158, w2158, w2160, w2158) -> (w2172:string)
                    n1154 = call "Add actual date time to string.vi"("String in"=w2172) -> ("String out"=w2176:string)  [unwired: 4 in]
                    n1155 = call "simple Shift string array.vi"("Element in"=w2176, "Array in"=w2174) -> ("Array out"=w2175:string[])  [unwired: 8 in, 1 out]
                  }
                  frame "End" {
                    w2227 = "Servo disconnected" ("Element in")
                    n1156 = Array Size(array=w2225) -> (size(s)=w2226:i32)
                    n1157 = local read "Instr status"() -> (w2234:T1)
                    n1158 = control-ref of="Servo controls"() -> (w2232:refnum<vi>)
                    n1159 = Delete From Array(array=w2225, length=w2226) -> (array with subset deleted=w2224:T10[])  [unwired: 1 in, 1 out]
                    n1160 = Bundle By Name(cluster=w2234, "Serv"=FALSE ("PSU")) -> (w2235:T1)
                    n1161 = local write "Instr status"(w2235) -> ()
                    n1162 = property class="Clust"(reference=w2232, "DisabledEnum"=T33."Disabled and Grayed Out" ("Disabled")) -> ()  [unwired: 1 in, 2 out]
                    n1163 = local read "loggersRef"() -> (w2228:refnum<file>)
                    n1164 = call "simple Shift string array.vi"("Element in"=w2227, "Array in"=w2229) -> ("Array out"=w2230:string[])  [unwired: 8 in, 1 out]
                    n1165 = call "Write in logger.vi"("String in"=w2227, "logger refnum"=w2228) -> ()  [unwired: 2 in, 2 out]
                  }
                  frame "Error", Default {
                    n1166 = Variant To Data(type=errorcluster {"status"=FALSE, "code"=0, "source"=""} ("error constant"), Variant=w2242) -> (data=w2240:errorcluster)  [unwired: 1 in, 1 out]
                    n1167 = Unbundle By Name(w2240) -> ("source"=w2239:string)
                    n1168 = call <vilib>:"Space Constant.vi"() -> ("String"=w2245:string)
                    n1169 = Concatenate Strings(w2244, w2245, w2239) -> (w2243:string)
                    n1170 = local read "loggersRef"() -> (w2238:refnum<file>)
                    n1171 = call "Add actual date time to string.vi"("String in"=w2243) -> ("String out"=w2237:string)  [unwired: 4 in]
                    n1172 = call "simple Shift string array.vi"("Element in"=w2237, "Array in"=w2247) -> ("Array out"=w2246:string[])  [unwired: 8 in, 1 out]
                    n1173 = call "Write in logger.vi"("String in"=w2237, "logger refnum"=w2238) -> ()  [unwired: 2 in, 2 out]
                  }
                }
                n1174 = Bundle By Name(cluster=w2048, "Servo"=w2045) -> (w2047:T8)
              }
              frame "Rotator" {
                n1175 = Format Into String(w2256) -> (resulting string=w2254:string)  [unwired: 3 in, 1 out]
                n1176 = Unbundle By Name(w2253) -> ("Rotator"=w2252:T86, "Magnet.Field [T]"=w2248:dbl)
                n1177 = case shown="\"Initialize\"" w2260 {
                  selector: w2260 -> [_ _ _ w2327 _ w2376 _ _]
                  tunnel: w2259 -> [_ w2282 w2322 w2351 w2372 w2385 w2399 w2420]
                  tunnel: w2258 -> [w2262 w2281 w2317 w2325 w2353 w2383 w2388 w2409]
                  tunnel: [w2262 w2280 w2317 w2323 w2352 w2382 w2387 w2408] -> w2257
                  tunnel: w2254 -> [_ w2277 _ w2326 _ w2375 _ _]
                  tunnel: w2252 -> [w2261 w2278 w2315 w2348 w2370 w2381 w2401 w2422]
                  tunnel: [w2261 w2271 w2314 w2347 w2370 w2381 w2400 w2421] -> w2250
                  tunnel: w2249 -> [_ w2269 w2313 w2346 _ _ w2395 w2416]
                  tunnel: w2248 -> [_ _ w2302 w2335 _ _ _ _]
                  frame "Ignore", Default {
                  }
                  frame "Initialize" {
                    n1178 = Variant To Data(type=T70 {"Controller info"={"deviceNumber"=0, "DeviceType"=0, "ID"=0, "Serial"="", "Address"="", "connected"=FALSE}, "Handle"=0, "FW-Version"=0, "Features"=0, "Axes"=[], "Path to DLL"=path ""} ("Rotator"), Variant=w2282) -> (data=w2279:T70)  [unwired: 1 in, 1 out]
                    n1179 = Unbundle By Name(w2279) -> ("ActuatorType"=w2268:u16, "Controller info.DeviceType"=w2270:i32, "Controller info.connected"=w2267:bool, "moving"=w2266:bool, "target"=w2265:bool, "Capacitance[uF]"=w2264:dbl, "Position [°]"=w2272:dbl, "Voltage [V]"=w2273:dbl, "Freque [Hz]"=w2263:dbl)
                    n1180 = case shown="True" w2267 {
                      tunnel: w2281 -> [w2284 w2287]
                      tunnel: [w2284 w2288] -> w2280
                      tunnel: w2277 -> [_ w2286]
                      tunnel: w2270 -> [_ w2285]
                      tunnel: ["Unknown" w2289] -> _
                      frame False {
                      }
                      frame True {
                        n1181 = case shown="1" w2285 {
                          tunnel: ["ANC350res" "ANC350num" "ANC350fps" "Unknown"] -> w2289
                          frame 0, Default {
                          }
                          frame 1 {
                          }
                          frame 2 {
                          }
                          frame 3 {
                          }
                        }
                        n1182 = call <vilib>:"Space Constant.vi"() -> ("String"=w2292:string)
                        n1183 = local read "loggersRef"() -> (w2290:refnum<file>)
                        n1184 = Concatenate Strings(w2286, w2292, "Rotator" ("string"), w2292, w2289) -> (w2291:string)
                        n1185 = call "Add actual date time to string.vi"("String in"=w2291) -> ("String out"=w2294:string)  [unwired: 4 in]
                        n1186 = call "Write in logger.vi"("String in"=w2294, "logger refnum"=w2290) -> ()  [unwired: 2 in, 2 out]
                        n1187 = call "simple Shift string array.vi"("Element in"=w2294, "Array in"=w2287) -> ("Array out"=w2288:string[])  [unwired: 8 in, 1 out]
                      }
                    }
                    n1188 = property on="Rot" class="Bool (strict)"("Value"=w2267) -> ()  [unwired: 2 in, 2 out]
                    n1189 = local read "Rotator controls"() -> (w2274:T22)
                    n1190 = Bundle By Name(cluster=w2274, "Motion properties.Frequency [Hz]"=w2263, "Motion properties.Amplitude [V]"=w2273, "Actual \nangle[°]"=w2272) -> (w2275:T22)
                    n1191 = Bundle By Name(cluster=w2278, "Name"=w2270, "Last update"=w2269, "Actuator"=w2268, "Connected"=w2267, "Moving"=w2266, "Target"=w2265, "Cap [nF]"=w2264) -> (w2271:T86)
                    n1192 = local write "Rotator controls"(w2275) -> ()
                  }
                  frame "Update" {
                    n1193 = Variant To Data(type=T71 {"Axis status"={"Connected"=FALSE, "Enabled"=FALSE, "Moving"=FALSE, "Target"=FALSE, "EndForward"=FALSE, "EndBackarwd"=FALSE, "Error"=FALSE}, "Position [°]"=0.0, "Frequency [Hz]"=0.0, "Voltage [V]"=0.0, "Capacitance[uF]"=0.0, "Name"="", "ActuatorType"=0, "DC offset [V]"=0.0, "Tolerance [m°]"=0.0, "Index"=0} ("Axis status"), Variant=w2322) -> (data=w2316:T71)  [unwired: 1 in, 1 out]
                    n1194 = Unbundle By Name(w2316) -> ("Axis status.Connected"=w2318:bool, "Position [°]"=w2301:dbl, "Axis status.Connected"=w2310:bool, "Axis status.Moving"=w2311:bool, "Axis status.Target"=w2312:bool, "Axis status.EndForward"=w2303:bool, "Axis status.EndBackarwd"=w2304:bool, "Axis status.Error"=w2305:bool, "Frequency [Hz]"=w2300:dbl, "Voltage [V]"=w2299:dbl)
                    n1195 = Less Or Equal?(x=w2302, y=8.0) -> (x <= y?=w2308:bool)
                    n1196 = Select(t=T33."Enabled" ("Disabled"), s=w2318, f=T33."Disabled and Grayed Out" ("Disabled")) -> ()  [unwired: 1 out]
                    n1197 = local read "Rotator controls"() -> (w2306:T22)
                    n1198 = Bundle By Name(cluster=w2306, "Motion properties.Amplitude [V]"=w2299, "Motion properties.Frequency [Hz]"=w2300, "Actual \nangle[°]"=w2301, "Set position.Safe to move?"=w2308, "EoF"=w2303, "EoB"=w2304, "Error"=w2305) -> (w2307:T22)
                    n1199 = Bundle By Name(cluster=w2315, "Last update"=w2313, "Position [°]"=w2301, "Connected"=w2310, "Moving"=w2311, "Target"=w2312) -> (w2314:T86)
                    n1200 = local write "Rotator controls"(w2307) -> ()
                  }
                  frame "Stop movement" {
                    n1201 = Variant To Data(type=T71 {"Axis status"={"Connected"=FALSE, "Enabled"=FALSE, "Moving"=FALSE, "Target"=FALSE, "EndForward"=FALSE, "EndBackarwd"=FALSE, "Error"=FALSE}, "Position [°]"=0.0, "Frequency [Hz]"=0.0, "Voltage [V]"=0.0, "Capacitance[uF]"=0.0, "Name"="", "ActuatorType"=0, "DC offset [V]"=0.0, "Tolerance [m°]"=0.0, "Index"=0} ("Axis status"), Variant=w2351) -> (data=w2349:T71)  [unwired: 1 in, 1 out]
                    n1202 = Unbundle By Name(w2349) -> ("Position [°]"=w2329:dbl, "Axis status.Connected"=w2343:bool, "Axis status.Moving"=w2344:bool, "Axis status.Target"=w2345:bool, "Axis status.EndForward"=w2336:bool, "Axis status.EndBackarwd"=w2337:bool, "Axis status.Error"=w2338:bool, "Frequency [Hz]"=w2334:dbl, "Voltage [V]"=w2333:dbl)  [unwired: 1 out]
                    n1203 = Less Or Equal?(x=w2335, y=8.0) -> (x <= y?=w2341:bool)
                    n1204 = local read "loggersRef"() -> (w2331:refnum<file>)
                    n1205 = Format Into String(format string=": %s at %.1f°", initial string=w2326, w2327, w2329) -> (resulting string=w2332:string, error out=w2330:errorcluster)  [unwired: 1 in]
                    n1206 = local read "Rotator controls"() -> (w2339:T22)
                    n1207 = Bundle By Name(cluster=w2339, "Motion properties.Amplitude [V]"=w2333, "Motion properties.Frequency [Hz]"=w2334, "Actual \nangle[°]"=w2329, "Set position.Safe to move?"=w2341, "EoF"=w2336, "EoB"=w2337, "Error"=w2338) -> (w2340:T22)
                    n1208 = call "Add actual date time to string.vi"("String in"=w2332) -> ("String out"=w2324:string)  [unwired: 4 in]
                    n1209 = call "Write in logger.vi"("error in"=w2330, "String in"=w2324, "logger refnum"=w2331) -> ()  [unwired: 1 in, 2 out]
                    n1210 = Bundle By Name(cluster=w2348, "Last update"=w2346, "Position [°]"=w2329, "Connected"=w2343, "Moving"=w2344, "Target"=w2345) -> (w2347:T86)
                    n1211 = local write "Rotator controls"(w2340) -> ()
                    n1212 = call "simple Shift string array.vi"("Element in"=w2324, "Array in"=w2325) -> ("Array out"=w2323:string[])  [unwired: 8 in, 1 out]
                  }
                  frame "Set parameters" {
                    n1213 = Variant To Data(type=T23 {"Frequency [Hz]"=1000.0, "MaxErr [µm|m°]"=10.0, "DC voltage [V]"=1.0, "Amplitude [V]"=6.0, "Position [mm|°]"=0.0, "EoF"=FALSE, "EoB"=FALSE, "Error"=FALSE, "Target [mm|°]"=0.0} ("Motion parameters"), Variant=w2372) -> (data=w2356:T23)  [unwired: 1 in, 1 out]
                    n1214 = local read "Rotator controls"() -> (w2357:T22)
                    n1215 = Bundle By Name(cluster=w2357, "Motion properties"=w2356) -> (w2360:T22)
                    n1216 = Unbundle By Name(w2360) -> ("Motion properties.Frequency [Hz]"=w2362:dbl, "Motion properties.MaxErr [µm|m°]"=w2363:dbl, "Motion properties.DC voltage [V]"=w2364:dbl, "Motion properties.Amplitude [V]"=w2365:dbl)
                    n1217 = local write "Rotator controls"(w2360) -> ()
                    n1218 = local read "loggersRef"() -> (w2355:refnum<file>)
                    n1219 = Format Into String(format string="\\n%s %.1f,%s %.1f,%s %.1f,%s %.1f", initial string="Rotator: new parameters set" ("String in"), "Freq [Hz]" ("input 1"), w2362, "Range [m°]" ("input 1"), w2363, "DC voltage [V]" ("input 1"), w2364, "Amplitude [Hz]" ("input 1"), w2365) -> (resulting string=w2361:string)  [unwired: 1 in, 1 out]
                    n1220 = call "Add actual date time to string.vi"("String in"=w2361) -> ("String out"=w2358:string)  [unwired: 4 in]
                    n1221 = call "Write in logger.vi"("String in"=w2358, "logger refnum"=w2355) -> ()  [unwired: 2 in, 2 out]
                    n1222 = call "simple Shift string array.vi"("Element in"=w2358, "Array in"=w2353) -> ("Array out"=w2352:string[])  [unwired: 8 in, 1 out]
                  }
                  frame "Set position" {
                    n1223 = Variant To Data(type=T24 {"Relative?"=FALSE, "Position [°]"=0.0, "Safe to move?"=FALSE} ("Set position"), Variant=w2385) -> (data=w2378:T24)  [unwired: 1 in, 1 out]
                    n1224 = Unbundle By Name(w2378) -> ("Position [°]"=w2374:dbl)
                    n1225 = Format Into String(format string=": %s %.1f°", initial string=w2375, w2376, w2374) -> (resulting string=w2373:string)  [unwired: 1 in, 1 out]
                    n1226 = local read "Rotator controls"() -> (w2380:T22)
                    n1227 = Bundle By Name(cluster=w2380, "Set position"=w2378) -> (w2379:T22)
                    n1228 = local write "Rotator controls"(w2379) -> ()
                    n1229 = call "simple Shift string array.vi"("Element in"=w2373, "Array in"=w2383) -> ("Array out"=w2382:string[])  [unwired: 8 in, 1 out]
                  }
                  frame "End" {
                    n1230 = Variant To Data(type=T70 {"Controller info"={"deviceNumber"=0, "DeviceType"=0, "ID"=0, "Serial"="", "Address"="", "connected"=FALSE}, "Handle"=0, "FW-Version"=0, "Features"=0, "Axes"=[], "Path to DLL"=path ""} ("Rotator"), Variant=w2399) -> (data=w2397:T70)  [unwired: 1 in, 1 out]
                    n1231 = Unbundle By Name(w2397) -> ("Controller info.DeviceType"=w2396:i32, "ActuatorType"=w2393:u16, "Controller info.connected"=w2394:bool, "moving"=w2392:bool, "target"=w2391:bool, "Capacitance[uF]"=w2390:dbl, "Position [°]"=w2389:dbl)
                    n1232 = Bundle By Name(cluster=w2401, "Name"=w2396, "Last update"=w2395, "Actuator"=w2393, "Connected"=w2394, "Moving"=w2392, "Target"=w2391, "Cap [nF]"=w2390, "Position [°]"=w2389) -> (w2400:T86)
                    n1233 = local read "Instr status"() -> (w2405:T1)
                    n1234 = Bundle By Name(cluster=w2405, "Rot"=FALSE ("PSU")) -> (w2406:T1)
                    n1235 = call "Add actual date time to string.vi"("String in"="Rotator module ended") -> ("String out"=w2386:string)  [unwired: 4 in]
                    n1236 = local write "Instr status"(w2406) -> ()
                    n1237 = local read "loggersRef"() -> (w2403:refnum<file>)
                    n1238 = call "simple Shift string array.vi"("Element in"=w2386, "Array in"=w2388) -> ("Array out"=w2387:string[])  [unwired: 8 in, 1 out]
                    n1239 = call "Write in logger.vi"("String in"=w2386, "logger refnum"=w2403) -> ()  [unwired: 2 in, 2 out]
                  }
                  frame "Disconnect" {
                    n1240 = Variant To Data(type=T70 {"Controller info"={"deviceNumber"=0, "DeviceType"=0, "ID"=0, "Serial"="", "Address"="", "connected"=FALSE}, "Handle"=0, "FW-Version"=0, "Features"=0, "Axes"=[], "Path to DLL"=path ""} ("Rotator"), Variant=w2420) -> (data=w2418:T70)  [unwired: 1 in, 1 out]
                    n1241 = Unbundle By Name(w2418) -> ("Controller info.DeviceType"=w2417:i32, "ActuatorType"=w2414:u16, "Controller info.connected"=w2415:bool, "moving"=w2413:bool, "target"=w2412:bool, "Capacitance[uF]"=w2411:dbl, "Position [°]"=w2410:dbl)
                    n1242 = local read "Instr status"() -> (w2426:T1)
                    n1243 = Bundle By Name(cluster=w2422, "Name"=w2417, "Last update"=w2416, "Actuator"=w2414, "Connected"=w2415, "Moving"=w2413, "Target"=w2412, "Cap [nF]"=w2411, "Position [°]"=w2410) -> (w2421:T86)
                    n1244 = Bundle By Name(cluster=w2426, "Rot"=FALSE ("PSU")) -> (w2427:T1)
                    n1245 = call "Add actual date time to string.vi"("String in"="Rotator module disconnected") -> ("String out"=w2407:string)  [unwired: 4 in]
                    n1246 = local write "Instr status"(w2427) -> ()
                    n1247 = local read "loggersRef"() -> (w2424:refnum<file>)
                    n1248 = call "Write in logger.vi"("String in"=w2407, "logger refnum"=w2424) -> ()  [unwired: 2 in, 2 out]
                    n1249 = call "simple Shift string array.vi"("Element in"=w2407, "Array in"=w2409) -> ("Array out"=w2408:string[])  [unwired: 8 in, 1 out]
                  }
                }
                n1250 = Bundle By Name(cluster=w2253, "Rotator"=w2250) -> (w2251:T8)
              }
              frame "Emty", Default {
                n1251 = Format Into String(w2433) -> (resulting string=w2432:string)  [unwired: 3 in, 1 out]
                n1252 = call <vilib>:"Space Constant.vi"() -> ("String"=w2434:string)
                n1253 = Concatenate Strings(w2432, w2434, w2431) -> (w2430:string)
                n1254 = call "simple Shift string array.vi"("Element in"=w2430, "Array in"=w2436) -> ("Array out"=w2435:string[])  [unwired: 8 in, 1 out]
              }
            }
          }
          frame True {
          }
        }
        "Instr info" <- w1257
        n1255 = local read "Busy"() -> (w1265:bool)
        n1256 = Unbundle By Name(w1256) -> ("Experiment state"=w1255:T28)
        n1257 = Not(x=w1265) -> (.not. x?=w1263:bool)
        n1258 = Greater?(x=w1268, y=2) -> (0:w1266:bool)
        n1259 = And(x=w1266, y=w1263) -> (x .and. y?=w1264:bool)
        n1260 = case shown="True" w1264 {
          selector: w1264 -> [w1283 w1284]
          tunnel: [w1281 TopStates."Check message" ("State")] -> w1262
          tunnel: w1255 -> [w1277 _]
          frame False {
            n1261 = local write "Busy"(w1283) -> ()
            n1262 = Equal?(x=w1277, y=experiment_state."Setup" ("Value")) -> (x = y?=w1279:bool)
            n1263 = Select(t=TopStates."Wait for Event" ("State"), s=w1279, f=TopStates."Check measurement") -> (s? t:f=w1281:T30)
          }
          frame True {
            "Busy" <- w1284
          }
        }
      }
      frame "Check measurement" {
        n1264 = Unbundle By Name(w2442) -> ("Experiment state"=w2444:T28, "Remains"=w2443:dbl)
        n1265 = case shown="\"Preparation\"" w2444 {
          tunnel: w2449 -> [_ w2478 w2514 _ _ w2673]
          tunnel: w2446 -> [w2452 w2467 w2509 w2579 w2585 w2674]
          tunnel: w2448 -> [w2453 w2487 w2513 w2580 w2590 w2707]
          tunnel: [w2453 w2485 w2512 w2580 w2590 w2706] -> w2447
          tunnel: [w2451 w2484 w2511 w2577 w2587 w2676] -> w2441
          tunnel: [w2452 w2467 w2508 w2579 w2585 w2675] -> w2445
          tunnel: w2440 -> [_ w2456 w2507 _ w2583 _]
          tunnel: w2443 -> [_ _ _ _ _ _]
          tunnel: w2442 -> [w2451 w2471 w2499 w2578 w2581 w2680]
          frame "Setup", Default {
            # "here can be implemented check of input parameters before measurement"
          }
          frame "Preparation" {
            n1266 = local read "VID control"() -> (w2457:T17)
            n1267 = property on="Script array" class="Arr (strict)"() -> ("Selection Start []"=w2474:u32[])  [unwired: 2 in, 2 out]
            n1268 = Unbundle By Name(w2467) -> ("F_start [GHz]"=w2462:dbl, "F_end [GHz]"=w2463:dbl, "Points [-]"=w2459:u32)
            n1269 = Index Array(array=w2474) -> (element=w2472:u32)  [unwired: 1 in]
            n1270 = Number To Decimal String(number=w2472) -> (decimal integer string=w2473:string)  [unwired: 1 in]
            n1271 = local read "tdms FDMR file ref"() -> (w2476:refnum<k34>)
            n1272 = Unbundle By Name(w2467) -> ("ModA [G]"=w2469:dbl)
            n1273 = local read "Acquisition controls"() -> (w2455:T14)
            n1274 = Unbundle By Name(w2455) -> ("Sample holder"=w2454:T16)
            n1275 = call "FDMR+ save measurement properties.vi"("FDMR+ script line"=w2467, "Description"=w2473, "Sample holder"=w2454, "Refnum in"=w2476) -> ("error out"=w2475:errorcluster)  [unwired: 6 in, 1 out]
            n1276 = call "Prepare FDMR plus measurement.vi"("Instr info"=w2456, "error in (no error)"=w2475, "Setup"=w2467, "VID control"=w2457, "Referencies in"=w2478) -> ("error out"=w2477:errorcluster)  [unwired: 6 in]
            n1277 = Quotient & Remainder(x=w2459, y=u32 8192) -> (floor(x/y)=w2460:u32)  [unwired: 1 out]
            n1278 = Bundle By Name(cluster=w2455, "Desired [G]"=w2469, "Adj mod"=TRUE ("AutoAdjust")) -> (w2470:T14)
            n1279 = Less Or Equal To 0?(x=w2460) -> (x <= 0?=w2461:bool)
            n1280 = case shown="True" w2461 {
              tunnel: w2460 -> [w2491 _]
              tunnel: w2459 -> [w2490 w2492]
              tunnel: [w2489 w2492] -> w2458
              frame False {
                n1281 = Divide(x=w2490, y=w2491) -> (x/y=w2489:dbl)
              }
              frame True {
              }
            }
            n1282 = local write "Acquisition controls"(w2470) -> ()
            n1283 = Subtract(x=w2463, y=w2462) -> (x-y=w2464:dbl)
            n1284 = Divide(x=w2464, y=w2458) -> (x/y=w2465:dbl)
            n1285 = property on="Live spectrum" class="WFGraph (strict)"("XScale.Offset"=w2462, "XScale.Multiplier"=w2465) -> ()  [unwired: 2 in, 2 out]
            n1286 = property on="Accumulated Spectrum" class="WFGraph (strict)"("XScale.Offset"=w2462, "XScale.Multiplier"=w2465) -> ()  [unwired: 2 in, 2 out]
            n1287 = call "Add actual date time to string.vi"("String in"="Preparing for measurement") -> ("String out"=w2488:string)  [unwired: 4 in]
            n1288 = call "simple Shift string array.vi"("Element in"=w2488, "Array in"=w2487) -> ("Array out"=w2485:string[])  [unwired: 8 in, 1 out]
            n1289 = Select(t=experiment_state."Setup", s=w2477, f=experiment_state."Stabilization" ("Value")) -> (s? t:f=w2479:T28)
            n1290 = Bundle By Name(cluster=w2471, "Experiment state"=w2479) -> (w2484:T27)
            "VTI tmp reached" <- FALSE ("VTI tmp reached")
            "Tmp reched time" <- u32 0 ("Tmp reched time")
          }
          frame "Stabilization" {
            n1291 = local read "VTI tmp reached"() -> (w2520:bool)
            n1292 = Unbundle By Name(w2507) -> ("Magnet.Field [T]"=w2502:dbl, "VTI.VTI [K]"=w2506:dbl, "PMD.Position [°]"=w2497:dbl)
            n1293 = Unbundle By Name(w2509) -> ("Angle [°]"=w2494:dbl, "Field [T]"=w2503:dbl, "Tmp [K]"=w2522:dbl, "Wait [min]"=w2505:dbl)
            n1294 = Not(x=w2520) -> (.not. x?=w2518:bool)
            n1295 = call "Is equal in tolerance.vi"("Absolut tolerance"=0.5, "Reference value"=w2522, "Input value"=w2506) -> ("Is in range"=w2517:bool)  [unwired: 1 in]
            n1296 = And(x=w2517, y=w2518) -> (x .and. y?=w2519:bool)
            n1297 = case shown="False" w2519 {
              tunnel: w2517 -> [w2559 _]
              tunnel: w2505 -> [w2558 w2571]
              tunnel: [w2557 FALSE] -> w2516
              tunnel: [w2556 w2571] -> w2504
              frame False {
                n1298 = case shown="True" w2559 {
                  selector: w2559 -> [w2561 _]
                  tunnel: w2558 -> [w2560 w2566]
                  tunnel: [w2561 w2564] -> w2557
                  tunnel: [w2560 w2562] -> w2556
                  frame False {
                    n1299 = local write "VTI tmp reached"(w2561) -> ()
                  }
                  frame True {
                    n1300 = local read "Tmp reched time"() -> (w2570:dbl)
                    n1301 = Get Date/Time In Seconds() -> (seconds since 1Jan1904=w2563:timestamp)
                    n1302 = To Double Precision Float(number=w2563) -> (double precision float=w2568:dbl)
                    n1303 = Multiply(x=w2566, y=60.0) -> (x*y=w2565:dbl)
                    n1304 = Subtract(x=w2568, y=w2570) -> (x-y=w2567:dbl)
                    n1305 = Subtract(x=w2565, y=w2567) -> (x-y=w2562:dbl)
                    n1306 = Less Or Equal To 0?(x=w2562) -> (x <= 0?=w2564:bool)
                  }
                }
              }
              frame True {
                n1307 = Get Date/Time In Seconds() -> (seconds since 1Jan1904=w2573:timestamp)
                n1308 = To Double Precision Float(number=w2573) -> (double precision float=w2572:dbl)
                n1309 = local write "VTI tmp reached"(TRUE ("VTI tmp reached")) -> ()
                n1310 = local write "Tmp reched time"(w2572) -> ()
              }
            }
            n1311 = call "Is equal in tolerance.vi"("Absolut tolerance"=0.1, "Reference value"=w2494, "Input value"=w2497) -> ("Is in range"=w2496:bool)  [unwired: 1 in]
            n1312 = call "Is equal in tolerance.vi"("Absolut tolerance"=0.01, "Reference value"=w2503, "Input value"=w2502) -> ("Is in range"=w2501:bool)  [unwired: 1 in]
            n1313 = Less Than 0?(x=w2494) -> (x < 0?=w2495:bool)
            n1314 = Or(x=w2496, y=w2495) -> (x .or. y?=w2493:bool)
            n1315 = Compound Arithmetic op=AND(w2493, w2501, w2516) -> (w2515:bool)
            n1316 = case shown="True" w2515 {
              tunnel: w2509 -> [w2523 w2532]
              tunnel: w2514 -> [_ w2539]
              tunnel: w2513 -> [w2525 w2545]
              tunnel: [w2525 w2544] -> w2512
              tunnel: [experiment_state."Stabilization" ("Value") w2542] -> w2510
              tunnel: [w2523 w2532] -> w2508
              frame False {
              }
              frame True {
                n1317 = Unbundle By Name(w2532) -> ("Points [-]"=w2528:u32)
                n1318 = local read "VID control"() -> (w2538:T17)
                n1319 = Quotient & Remainder(x=w2528, y=u32 8192) -> (floor(x/y)=w2530:u32)  [unwired: 1 out]
                n1320 = Initialize Array(sgl 0.0, w2528) -> (w2527:sgl[])
                n1321 = Less Or Equal To 0?(x=w2530) -> (x <= 0?=w2531:bool)
                n1322 = case shown="False" w2531 {
                  tunnel: w2530 -> [w2552 _]
                  tunnel: w2527 -> [w2554 w2555]
                  tunnel: [w2553 w2555] -> w2526
                  frame False {
                    n1323 = call-poly <vilib>:"Decimate (single shot).vi"("decimating factor"=w2552, "X"=w2554) -> ("Decimated Array"=w2553:dbl[])  [unwired: 8 in, 1 out]
                  }
                  frame True {
                  }
                }
                n1324 = call "Add actual date time to string.vi"("String in"="Starting measurement") -> ("String out"=w2546:string)  [unwired: 4 in]
                n1325 = call "simple Shift string array.vi"("Element in"=w2546, "Array in"=w2545) -> ("Array out"=w2544:string[])  [unwired: 8 in, 1 out]
                n1326 = disable-structure shown="Disabled" {
                  disable-tunnel: w2539 -> [w2551 _]
                  disable-tunnel: w2538 -> [w2550 _]
                  disable-tunnel: [w2549 _] -> w2537
                  disable-tunnel: w2532 -> [w2548 _]
                  frame Disabled {
                    n1327 = call "Begin FDMR plus measurement.vi"("VID control"=w2550, "FDMR+ script line"=w2548, "Referencies in"=w2551) -> ("error out"=w2549:errorcluster)  [unwired: 8 in]
                  }
                  frame Enabled {
                  }
                }
                n1328 = Build Array(w2526, w2526) -> (w2534:dbl[][])
                n1329 = Build Array(w2527, w2527) -> (→"Acummulated data":sgl[][])
                n1330 = local write "Accumulated Spectrum"(w2534) -> ()
                n1331 = Select(t=experiment_state."Save" ("Value"), s=w2537, f=experiment_state."Begin" ("Value")) -> (s? t:f=w2542:T28)
                "Running experiment" <- TRUE ("Running experiment")
                "Round" <- 0 ("Averages done")
              }
            }
            n1332 = Bundle By Name(cluster=w2499, "Remains"=w2504, "Experiment state"=w2510) -> (w2511:T27)
          }
          frame "Begin" {
            n1333 = Bundle By Name(cluster=w2578, "Experiment state"=experiment_state."Acquisition") -> (w2577:T27)
          }
          frame "Acquisition" {
            n1334 = local read "New data"() -> (w2584:bool)
            n1335 = case shown="True" w2584 {
              selector: w2584 -> [_ w2660]
              tunnel: [FALSE w2648] -> w2591
              tunnel: w2585 -> [_ w2649]
              tunnel: w2583 -> [_ w2661]
              tunnel: w2581 -> [w2593 _]
              tunnel: [w2592 w2645] -> w2582
              frame False {
                n1336 = Unbundle By Name(w2593) -> ("Remains"=w2592:dbl)
              }
              frame True {
                w2616 = TRUE ("averaging")
                w2635 = sgl 0.0  # background
                n1337 = Unbundle By Name(w2649) -> ("Repeat [-]"=w2608:i32, "Points [-]"=w2604:u32, "Sampling Rate"=w2614:T26, "Comment"=w2615:string)
                n1338 = Not(x=w2660) -> (.not. x?=w2659:bool)
                n1339 = local read "SMU controls"() -> (w2599:T21)
                n1340 = local write "New data"(w2659) -> ()
                n1341 = local read "Acquisition controls"() -> (w2658:T14)
                n1342 = Unbundle By Name(w2661) -> ("VTI.VTI [K]"=w2654:dbl, "Magnet.Field [T]"=w2657:dbl, "VTI.Sample [K]"=w2595:dbl)
                n1343 = Unbundle By Name(w2658) -> ("Modulation [A]"=w2653:dbl)
                n1344 = property on="Script array" class="Arr (strict)"() -> ("Selection Start []"=w2642:u32[])  [unwired: 2 in, 2 out]
                n1345 = local read "Acummulated data"() -> (w2628:sgl[][])
                n1346 = Unbundle By Name(w2599) -> ("B[T]"=w2598:dbl)
                n1347 = Index Array(array=w2642) -> (element=w2640:u32)  [unwired: 1 in]
                n1348 = Scale By Power Of 2(n=w2614, x=1.0) -> (x*2^n=w2612:dbl)
                n1349 = Number To Decimal String(number=w2640) -> (decimal integer string=w2639:string)  [unwired: 1 in]
                n1350 = Multiply(x=w2604, y=w2612) -> (x*y=w2611:dbl)
                n1351 = local read "Lock-in data"() -> (w2638:T2)
                n1352 = Quotient & Remainder(x=w2604, y=u32 8192) -> (floor(x/y)=w2602:u32)  [unwired: 1 out]
                n1353 = Divide(x=w2611, y=60000000.0) -> (x/y=w2606:dbl)
                n1354 = Concatenate Strings(w2639, "_" ("string"), w2615) -> (w2643:string)
                n1355 = local read "tdms FDMR file ref"() -> (w2647:refnum<k34>)
                n1356 = Unbundle(w2638) -> ("X"=w2637:sgl[], "Y"=w2636:sgl[])
                n1357 = local read "Round"() -> (w2607:i32)
                n1358 = Subtract(x=w2636, y=w2635) -> (x-y=w2632:sgl[])
                n1359 = Subtract(x=w2637, y=w2635) -> (x-y=w2633:sgl[])
                n1360 = Build Array(w2653, w2654, w2657, w2595, w2598) -> (w2655:dbl[])
                n1361 = To Single Precision Float(number=w2655) -> (single precision float=w2652:sgl[])
                n1362 = Build Array(w2633, w2632) -> (w2631:sgl[][])
                n1363 = Format Into String(w2607) -> (resulting string=w2629:string)  [unwired: 3 in, 1 out]
                n1364 = Add(x=w2628, y=w2631) -> (x+y=w2627:sgl[][])
                n1365 = Increment(x=w2607) -> (x+1=w2650:i32)
                n1366 = call "Normalize 1D float array.vi"("Signal treat"=T72."None", "Data in"=w2633) -> ("Data out"=w2623:sgl[])  [unwired: 9 in]
                n1367 = call "Normalize 1D float array.vi"("Signal treat"=T72."None", "Data in"=w2632) -> ("Data out"=w2622:sgl[])  [unwired: 9 in]
                n1368 = local write "Acummulated data"(w2627) -> ()
                n1369 = Index Array(array=w2627) -> (element #1=w2617:sgl[], element #2=w2620:sgl[])  [unwired: 4 in]
                n1370 = local write "Round"(w2650) -> ()
                n1371 = TDMS Write(0:w2647, 1:enum16{"decimated", "interleaved"}."interleaved" ("data layout (0:decimated)"), 5:w2643, 7:string[] ["Modulation", "VTI", "Field", "Sample", "Field sensor"] ("group name in (Untitled)"), 9:w2652) -> (4:w2646:refnum<k34>, 6:w2644:string)  [unwired: 1 in, 2 out]
                n1372 = Less Or Equal To 0?(x=w2602) -> (x <= 0?=w2603:bool)
                n1373 = Build Array(w2623, w2622) -> (w2625:sgl[][])
                n1374 = Select(t=u32 1, s=w2603, f=w2602) -> (s? t:f=w2601:u32)
                n1375 = case shown="False" "Save data option" {
                  tunnel: w2646 -> [w2671 w2672]
                  tunnel: w2644 -> [w2669 _]
                  tunnel: w2629 -> [w2665 _]
                  tunnel: w2625 -> [w2662 _]
                  frame False {
                    n1376 = Concatenate Strings("X", w2665) -> (w2664:string)
                    n1377 = Concatenate Strings("Y", w2665) -> (w2663:string)
                    n1378 = Build Array(w2664, w2663) -> (w2668:string[])
                    n1379 = TDMS Write(0:w2671, 5:w2669, 7:w2668, 9:w2662) -> (4:w2670:refnum<k34>)  [unwired: 2 in, 3 out]
                    n1380 = local write "tdms FDMR file ref"(w2670) -> ()
                  }
                  frame True {
                    n1381 = local write "tdms FDMR file ref"(w2672) -> ()
                  }
                }
                n1382 = Subtract(x=w2608, y=w2607) -> (x-y=w2609:i32)
                n1383 = Compound Arithmetic op=MULTIPLY(w2609, w2606) -> (w2645:dbl)
                n1384 = call-poly <vilib>:"Decimate (single shot).vi"("averaging"=w2616, "decimating factor"=w2601, "X"=w2617) -> ("Decimated Array"=w2618:dbl[])  [unwired: 7 in, 1 out]
                n1385 = call-poly <vilib>:"Decimate (single shot).vi"("averaging"=w2616, "decimating factor"=w2601, "X"=w2620) -> ("Decimated Array"=w2619:dbl[])  [unwired: 7 in, 1 out]
                n1386 = call-poly <vilib>:"Decimate (single shot).vi"("averaging"=w2616, "decimating factor"=w2601, "X"=w2623) -> ("Decimated Array"=w2624:dbl[])  [unwired: 7 in, 1 out]
                n1387 = call-poly <vilib>:"Decimate (single shot).vi"("averaging"=w2616, "decimating factor"=w2601, "X"=w2622) -> ("Decimated Array"=w2621:dbl[])  [unwired: 7 in, 1 out]
                n1388 = Build Array(w2618, w2619) -> (→"Accumulated Spectrum":dbl[][])
                n1389 = Build Array(w2624, w2621) -> (→"Live spectrum":dbl[][])
                n1390 = Less Or Equal To 0?(x=w2609) -> (x <= 0?=w2648:bool)
              }
            }
            n1391 = Select(t=experiment_state."Save" ("Value"), s=w2591, f=experiment_state."Acquisition" ("Value")) -> (s? t:f=w2586:T28)
            n1392 = Bundle By Name(cluster=w2581, "Experiment state"=w2586, "Remains"=w2582) -> (w2587:T27)
          }
          frame "Save" {
            n1393 = Unbundle By Name(w2674) -> ("Comment"=w2689:string)
            n1394 = property on="Script array" class="Arr (strict)"() -> ("Selection Start []"=w2692:u32[])  [unwired: 2 in, 2 out]
            n1395 = local read "Script array"() -> (w2685:T25[])
            n1396 = Index Array(array=w2692) -> (element=w2687:u32)  [unwired: 1 in]
            n1397 = Increment(x=w2687) -> (x+1=w2684:u32)
            n1398 = Number To Decimal String(number=w2687) -> (decimal integer string=w2691:string)  [unwired: 1 in]
            n1399 = local read "Run FDMR+ btn"() -> (w2681:bool)
            n1400 = Array Size(array=w2685) -> (size(s)=w2686:i32)
            n1401 = Concatenate Strings(w2691, "_" ("string"), w2689) -> (w2688:string)
            n1402 = Greater?(x=w2686, y=w2684) -> (0:w2683:bool)
            n1403 = And(x=w2681, y=w2683) -> (x .and. y?=w2682:bool)
            n1404 = local read "Instr control refs"() -> (w2698:refnum<vi>[])
            n1405 = control-ref of="Run FDMR+ btn"() -> (w2696:refnum<vi>)
            n1406 = local read "Acummulated data"() -> (w2695:sgl[][])
            n1407 = local read "tdms FDMR file ref"() -> (w2710:refnum<k34>)
            n1408 = Build Array (concatenate)(w2696, w2698) -> (w2699:refnum<vi>[])
            n1409 = call "Dis- or en- able controls.vi"("Disabled"=T33."Enabled", "Control referencies"=w2699) -> ("error out"=w2693:errorcluster)  [unwired: 9 in]
            n1410 = TDMS Write(0:w2710, 5:w2688, 7:string[] ["X sum", "Y sum"] ("group name in (Untitled)"), 9:w2695, 11:w2693) -> (4:w2679:refnum<k34>, 15:w2678:errorcluster)  [unwired: 1 in, 2 out]
            n1411 = TDMS Close(8:w2678, 11:w2679) -> (3:w2677:path)  [unwired: 1 out]
            n1412 = case shown="True" w2682 {
              tunnel: w2684 -> [_ w2725]
              tunnel: w2685 -> [_ w2726]
              tunnel: w2680 -> [w2716 w2723]
              tunnel: [w2715 w2722] -> w2676
              tunnel: w2677 -> [_ w2720]
              tunnel: [w2713 w2719] -> w2675
              tunnel: w2674 -> [w2713 w2718]
              tunnel: w2673 -> [_ w2717]
              frame False {
                n1413 = property on="Script array" class="Arr (strict)"("Selection Start []"=u32[] [0] ("Selection Start[]")) -> ()  [unwired: 2 in, 2 out]
                n1414 = local write "Run FDMR+ btn"(FALSE ("Run FDMR+ btn")) -> ()
                n1415 = Bundle By Name(cluster=w2716, "Experiment state"=experiment_state."Setup") -> (w2715:T27)
              }
              frame True {
                n1416 = Array Subset(array=w2726, index=w2725) -> (w2727:T25[])  [unwired: 1 in]
                n1417 = for {
                  tunnel: w2727 -> [w2754] mode=indexing
                  tunnel: [w2756] -> w2724
                  tunnel: [w2755] -> w2728
                  tunnel: [w2754] -> w2719
                  i -> [w2755]
                  stop <- w2756 stop-if-true
                  n1418 = Unbundle By Name(w2754) -> ("Execute"=w2756:bool)
                }
                n1419 = Add(x=w2725, y=w2728) -> (x+y=w2721:u32)
                n1420 = case shown="True" w2724 {
                  tunnel: w2723 -> [w2749 w2753]
                  tunnel: [w2747 w2751] -> w2722
                  tunnel: w2721 -> [w2746 _]
                  tunnel: w2720 -> [w2744 _]
                  tunnel: w2719 -> [w2741 _]
                  tunnel: w2718 -> [w2740 _]
                  tunnel: w2717 -> [w2736 _]
                  frame True {
                    n1421 = Build Array(w2746) -> (w2745:u32[])
                    n1422 = Unbundle By Name(w2741) -> ("Field [T]"=w2739:dbl)
                    n1423 = Unbundle By Name(w2740) -> ("Field [T]"=w2738:dbl)
                    n1424 = property on="Script array" class="Arr (strict)"("Selection Start []"=w2745) -> ()  [unwired: 2 in, 2 out]
                    n1425 = call "Is equal in tolerance.vi"("Absolut tolerance"=0.01, "Reference value"=w2738, "Input value"=w2739) -> ("Is in range"=w2731:bool)  [unwired: 1 in]
                    n1426 = TDMS Open(10:T73."open" ("operation (0:open)"), 11:w2744) -> (3:w2742:refnum<k34>)  [unwired: 5 in, 1 out]
                    n1427 = local write "tdms FDMR file ref"(w2742) -> ()
                    n1428 = Bundle By Name(cluster=w2749, "Experiment state"=experiment_state."Preparation" ("Value")) -> (w2747:T27)
                    n1429 = Unbundle By Name(w2736) -> ("Field_C"=w2735:refnum<queue>)
                    n1430 = Select(t=Magnet_mode_public."Persistant" ("Mode"), s=w2731, f=Magnet_mode_public."Ramping" ("Mode")) -> (s? t:f=w2732:T34)
                    n1431 = Bundle By Name(cluster=T37 {"Command"=enum."Switch mode", "Data"=variant} ("MSG to magnet"), "Data"=w2732) -> (w2733:T37)
                    n1432 = call "Put in mailbox.vi"("Message"=w2733, "Queue in"=w2735) -> ()  [unwired: 7 in, 3 out]
                  }
                  frame False {
                    n1433 = Bundle By Name(cluster=w2753, "Experiment state"=experiment_state."Setup" ("Value")) -> (w2751:T27)
                    n1434 = local write "Run FDMR+ btn"(FALSE ("Run FDMR+ btn")) -> ()
                  }
                }
              }
            }
            n1435 = Path To String(path=w2677) -> (string=w2704:string)
            n1436 = Concatenate Strings("Measurrement finished " ("String in"), w2704) -> (w2705:string)
            n1437 = call "Add actual date time to string.vi"("String in"=w2705) -> ("String out"=w2709:string)  [unwired: 4 in]
            n1438 = call "simple Shift string array.vi"("Element in"=w2709, "Array in"=w2707) -> ("Array out"=w2706:string[])  [unwired: 8 in, 1 out]
            n1439 = Unbundle By Name(w2673) -> ("Data_Aq"=w2702:refnum<queue>)
            n1440 = Bundle By Name(cluster=T50 {"Command"=enum."Set individual parameters", "Data"=variant} ("MSG for  ACQ"), "Data"=T47 {"parameter"=enum."scope_trigEn", "value"=0.0} ("Parameter to set")) -> (w2700:T50)
            n1441 = call "Put in mailbox.vi"("Message"=w2700, "Queue in"=w2702) -> ()  [unwired: 7 in, 3 out]
          }
        }
      }
      frame "Stop" {
        n1442 = call "simple Shift string array.vi"("Element in"="Program stopped", "Array in"=w2762) -> ("Array out"=w2761:string[])  [unwired: 8 in, 1 out]
      }
      frame "Restart" {
        n1443 = Build Array("Program restarted") -> (w2767:string[])
      }
    }
    n1444 = Tick Count (ms)() -> (millisecond timer value=w20:u32)
    n1445 = Subtract(x=w20, y=w19) -> (x-y=→"1 round\ntime":u32)
  }
  n1446 = case shown="True" "Real instruments" {
    tunnel: w10 -> [w2779 w2787]
    frame True {
      n1447 = Unbundle By Name(w2779) -> ("Mod_M"=w2772:refnum<queue>, "Field_C"=w2774:refnum<queue>, "MW_C"=w2776:refnum<queue>, "Angle_C"=w2777:refnum<queue>, "Table_C"=w2778:refnum<queue>, "Data_Aq"=w2773:refnum<queue>, "Tmp_C"=w2775:refnum<queue>, "TOP"=w2771:refnum<queue>)
      n1448 = call "TemperatureController main.vi"("Supervising module"=w2771, "Controller module"=w2775) -> ()  [unwired: 10 in]
      n1449 = call "MFLI module main.vi"("Master mailbox"=w2771, "Module mailbox"=w2773) -> ()  [unwired: 10 in]
      n1450 = call "Servo main.vi"("Queue to UI"=w2771, "Module queue servo"=w2778) -> ()  [unwired: 10 in]
      n1451 = call "PiezoController main.vi"("Top"=w2771, "Rotator"=w2777) -> ()  [unwired: 9 in, 1 out]
      n1452 = call "Module for RF and LO synthesizer.vi"("Main controller mailbox"=w2771, "THz module mailbox"=w2776) -> ()  [unwired: 10 in]
      n1453 = call "MagnetTop.vi"("Queue to UI"=w2771, "Module queue"=w2774) -> ()  [unwired: 10 in]
      n1454 = call "SMU 2450 main.vi"("update time (100ms)"=u32 500, "Mailbox address Top"=w2771, "Module mailbox"=w2772) -> ()  [unwired: 7 in, 2 out]
    }
    frame False {
      n1455 = Unbundle By Name(w2787) -> ("Field_C"=w2782:refnum<queue>, "MW_C"=w2784:refnum<queue>, "Angle_C"=w2785:refnum<queue>, "Table_C"=w2786:refnum<queue>, "Data_Aq"=w2781:refnum<queue>, "Tmp_C"=w2783:refnum<queue>, "TOP"=w2780:refnum<queue>)
      n1456 = call "Fake VTI module.vi"("Top address in"=w2780, "VTI Module ref"=w2783) -> ()  [unwired: 10 in]
      n1457 = call "fake lock-in module.vi"("Master mailbox"=w2780, "Module mailbox"=w2781) -> ()  [unwired: 10 in]
      n1458 = call "fake Servo modue.vi"("Queue to UI"=w2780, "Module queue servo"=w2786) -> ()  [unwired: 10 in]
      n1459 = call "fake SampleRotator module.vi"("Top"=w2780, "Rotator"=w2785) -> ()  [unwired: 8 in, 2 out]
      n1460 = call "fake THz module.vi"("Main controller mailbox"=w2780, "THz module mailbox"=w2784) -> ()  [unwired: 10 in]
      n1461 = call "fake main magnet module.vi"("Queue to UI"=w2780, "Module queue"=w2782) -> ()  [unwired: 10 in]
    }
  }
  n1462 = flat-sequence {
    tunnel: w5 -> [_]
    frame #0 {
      n1463 = Stop(stop? (T)=TRUE) -> ()
    }
  }
